vi "DialogCreateMethod.vi"(0 "ClassWriterNative":refnum<class "ClassWriterNative.lvclass">, 1 "ClassItemRefIn":refnum<vi>, 5 "error in (no error)":errorcluster) -> (14 "ClassWriterNative":refnum<class "ClassWriterNative.lvclass">, 15 "ClassItemRefOut":refnum<vi>, 16 "CreateMethodData":T3={"MethodName"="", "RelativeMethodPath"=path "", "MethodDescription"="", "Scope/Visibility"=enum."Use Parent Folder Scope", "MethodTemplateName"="", "IconOut"=[], "RelativeProjectClassPath"="", "OpenViAfterCreation"=FALSE, "DynamicDispatchVi"=FALSE, "ExtraCreateParameters"=variant, "MustOverride"=FALSE, "MustCallParent"=FALSE, "IconDetails"={"IconSize"=enum."1 c-term high", "ImageRows(32)"=32, "ConnectorPaneHeight"=[]}, "AF-Option"=variant, "TemplatePath"=path ""} {"IconOut" format="%x"}, 17 "Cancelled":bool, 19 "error out":errorcluster)   [LabVIEW 2020, in "ClassWriterNative.lvclass"]
uses:
  <resource>/Framework/Providers/Open_GDS/ClassProviders/Provider_LvNativeClass/ClassWriterNative_class/ClassWriterNative.lvclass
  <resource>/Framework/Providers/Open_GDS/ClassProviders/Common/LvIcon_class/GDSLvIcon_ColorControl.ctl
  <resource>/Framework/Providers/Open_GDS/ClassProviders/Provider_BaseClassInterface/CreateMethodData.ctl
  <resource>/Framework/Providers/Open_GDS/ClassProviders/Provider_EndevoGOOP300/GOOP300_SubVIs/GOOP300_MethodScopeType.ctl
  <resource>/Framework/Providers/Open_GDS/ClassProviders/Provider_LvNativeClass/ClassWriterNative_class/IconDetails.ctl
  <resource>/Framework/Providers/Open_GDS/ClassProviders/Provider_LvNativeClass/ClassWriterNative_class/IconSize.ctl
  <resource>/Framework/Providers/Open_GDS/ClassProviders/Common/LvClass_class/GDSLvClass_PlugIn.ctl
  <resource>/Framework/Providers/Open_GDS/ClassProviders/Common/LvClass_class/GDSLvClass_PlugInTypes.ctl
  <resource>/Framework/Providers/Open_GDS/ClassProviders/Provider_LvNativeClass/ClassWriterNative_class/MethodInfo.ctl
  <resource>/Framework/Providers/Open_GDS/ClassProviders/Provider_LvNativeClass/ClassWriterNative_class/MethodType.ctl
  <vilib>/Utility/miscctls.llb/LVPoint32TypeDef.ctl
  <vilib>/picture/picture.llb/imagedata.ctl
  <resource>/Framework/Providers/Open_GDS/ClassProviders/Provider_BaseClassInterface/ClassWriter_class/TemplateSettings.ctl
  <vilib>/Utility/miscctls.llb/LVRectTypeDef.ctl
  <resource>/Framework/Providers/Open_GDS/ClassProviders/Provider_EndevoGOOP400/EndevoG4ProviderName.ctl
  <vilib>/event_ctls.llb/lveventtype.ctl
  <resource>/Framework/Providers/Open_GDS/ClassProviders/Common/IconEditor/private/GDSIconEditor_IconDialog_Input.vi
  <resource>/Framework/Providers/Open_GDS/ClassProviders/Common/LvIcon_class/subvis/GDSLvIcon_TextDataType.ctl
  <resource>/Framework/Providers/Open_GDS/ClassProviders/Common/LvIcon_class/GDSLvIcon_WordCompressionType.ctl
  <resource>/Framework/Providers/Open_GDS/ClassProviders/Common/LvIcon_class/GDSLvIcon_TextAlignment.ctl
  <vilib>/Utility/miscctls.llb/LVPositionTypeDef.ctl
  <vilib>/Utility/miscctls.llb/LVPointTypeDef.ctl
  55204018-4493-42a1-99d2-4693747e47a6.vi
  5ca582aa-8486-41e5-93f7-81c5295e79eb.vi
  <vilib>/Utility/config.llb/Read Key (String).vi
  <vilib>/Comparison/Equal/Equal Functor/Equal Functor.lvclass
  <vilib>/regexp/Match Regular Expression.xnode
  <resource>/Framework/Providers/Open_GDS/ClassProviders/Provider_BaseClassInterface/ClassWriter_class/ClassWriter.lvclass
  <vilib>/Utility/lvfile.llb/NI_FileType.lvlib
  <resource>/Framework/Providers/Open_GDS/ClassProviders/Provider_EndevoGOOP400/ClassWriterGOOP400_class/ClassWriterGOOP400.lvclass
  <vilib>/Utility/config.llb/NI_LVConfig.lvlib
  <resource>/Framework/Providers/Open_GDS/ClassProviders/Provider_EndevoGOOP300/ClassWriterGOOP300_class/ClassWriterGOOP300.lvclass
panel:
  out "MethodTemplateImage":picture
  in  "_AddFolder":bool
  in  "Filter":string
  in  ".vim":bool
  out "_MethodsLlocationOverrideInfo":string=" \n\n" caption="The methods location is controlled by\nthe method you override."
  out "ProductPicture":picture
  out "_IconPreview":picture caption="Icon Preview"
  out "DragIcon":picture
  in  "_AddMessageClass":bool
  in  "FloodFillMask":bool
  out "_IconName":string
  in  "_IconSearchText":string caption="Icon search text"
  in  "_Manage":bool
  in  "_Folders":u16(ring) caption="Folders" items=["<All icons>", "C:\\Users\\Mikael\\Documents\\LabVIEW Data\\Glyphs", "...EW 2010\\resource\\Framework\\Providers\\Icons", "...\\Framework\\Providers\\Symbio_GDS_SVN\\Glyphs", "...e\\Framework\\Providers\\Symbio_GDS_SVN\\Icons"]
  out "Icons":picture
  in  "_MethodIcons":bool
  in  "_TextAlignment":u16(ring) caption="Text Alignment" items=["Center", "Left", "Right"]
  in  "_IconSize":u16(ring) caption="Icon Size" items=["Full", "1 c-term high", "2 c-term high", "3 c-term high"]
  in  "_MustCallParent":bool caption="Must Call Parent"
  in  "_MustOverride":bool caption="Must Override"
  out "_VisibilityAndLlocationGrouping":string caption="Visibility and location"
  out "_IconGrouping":string caption="Icon"
  in  "_MethodSignature":u16(ring) caption="Method signature" items=["No signature", "-", "Add signature"]
  in  "_ShowContextHelp":bool
  in  "Help":bool
  in  "_CreateOpenClass":bool
  in  "_MethodIconName":string caption="Body Text"
  in  "_BodyBk":T1 caption="Body Background"
  in  "_BodyText":T1 caption="Body text"
  in  "_FontCompression":enum16{"Auto", "On", "Off"}(ring) caption="Font Compression"
  in  "_CapitalOnly":bool=TRUE caption="Force Capital Letters"
  out "_DubMethodName":string caption="This method already exists in the class"
  out "_Loading":string caption="Loading..."
  in  "_OverrideMethods":i32(listbox) caption="Override Methods"
  in  "_MethodType":T2(radio) caption="Method Type"
  in  "_Property":string[](tree) caption="Data Fields/Attributes"
  in  "_DynamicDispatch":bool caption="Dynamic Dispatch"
  in  "_Visibility":T7(radio) caption="Visibility"
  in  "_MethodLocation":i32(listbox) caption="Method Location"
  in  "_MethodName":string caption="Method Name"
  in  "_Cancel":bool
  in  "_CreateMethod":bool
  in  "_MethodDescription":string caption="Method description"
  in  "_Method":i32[](listbox) caption="Method Template"
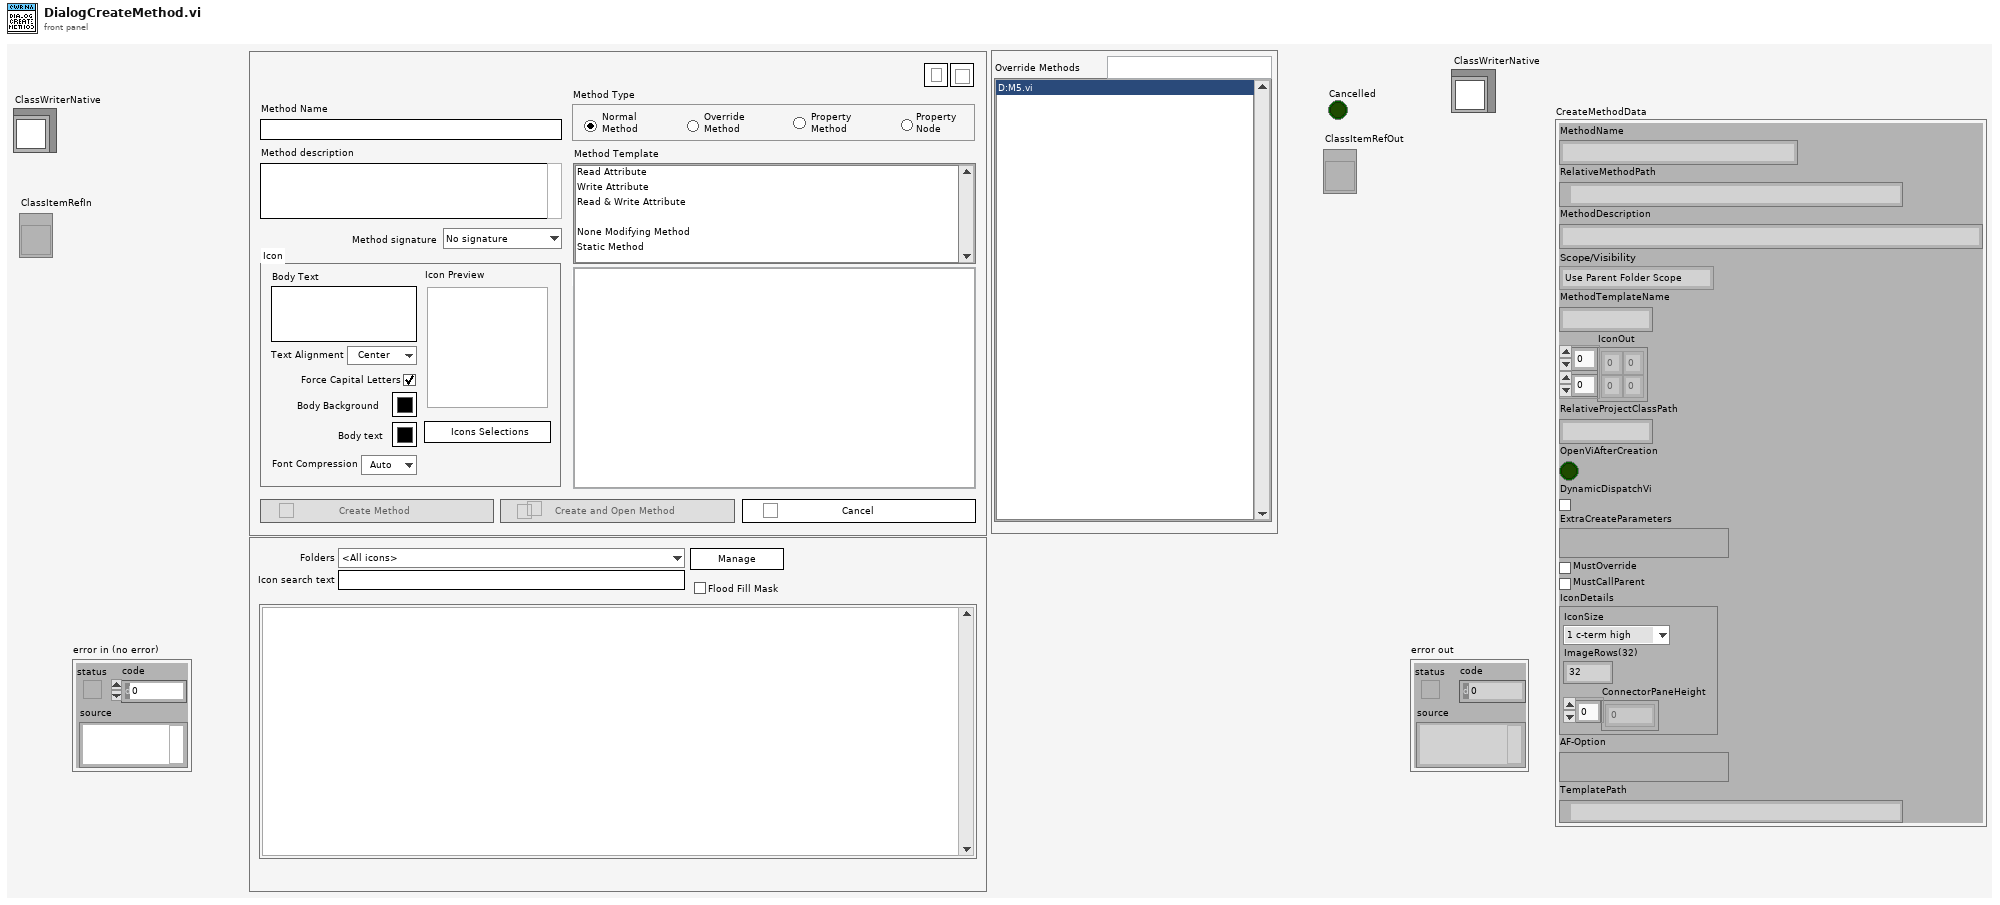
[diagram p1: front panel]
types:
  T1 = typedef "GDSLvIcon_ColorControl.ctl" = cluster{"Decal":bool, "Color":u32}
  T2 = enum32{"Normal Method", "Override Method", "Property Method", "Property Node"}
  T3 = typedef "ClassWriter.lvclass/CreateMethodData.ctl" = cluster{"MethodName":string, "RelativeMethodPath":path, "MethodDescription":string, "Scope/Visibility":T4, "MethodTemplateName":string, "IconOut":u8[][], "RelativeProjectClassPath":string, "OpenViAfterCreation":bool, "DynamicDispatchVi":bool, "ExtraCreateParameters":variant, "MustOverride":bool, "MustCallParent":bool, "IconDetails":T5, "AF-Option":variant, "TemplatePath":path}
  T4 = typedef "GOOP300_MethodScopeType.ctl" = enum16{"Use Parent Folder Scope", "Public", "Protected", "Private", "Community"}
  T5 = typedef "ClassWriterNative.lvclass/IconDetails.ctl" = cluster{"IconSize":T6, "ImageRows(32)":i32, "ConnectorPaneHeight":i32[]}
  T6 = typedef "ClassWriterNative.lvclass/IconSize.ctl" = enum16{"Full", "1 c-term high", "2 c-term high", "3 c-term high"}
  T7 = enum32{"Public", "Community", "Protected", "Private"}
  T8 = cluster{"Font Name":string, "Size":u16, "Bold":bool, "Italic":bool, "Underline":bool, "Strikeout":bool, "Color":u32}
  T9 = cluster{"AttributeNames":string[], "PropertyNode":bool, "FolderNames":string[]}
  T10 = typedef "GDSLvClass_PlugIn.ctl" = cluster{"Type":T11, "ID":string, "Version":string, "Path":path, "Name":string, "Data":variant}
  T11 = typedef "GDSLvClass_PlugInTypes.ctl" = enum16{"DesignPattern", "MethodTypes"}
  T12 = typedef "ClassWriterNative.lvclass/MethodInfo.ctl" = cluster{"Type":T13, "Name":string, "Path":path, "ExtraName":string, "Data":variant}
  T13 = typedef "ClassWriterNative.lvclass/MethodType.ctl" = enum16{"Normal", "MethodPlugIn", "DesignPattern", "AF-Method"}
  T14 = typedef "LVPoint32TypeDef.ctl" = cluster{"Horizontal":i32, "Vertical":i32}
  T15 = typedef "imagedata.ctl" = cluster{"image type":i32, "image depth":i32, "image":u8[], "mask":u8[], "colors":u32[], "Rectangle":cluster{"left":i16, "top":i16, "right":i16, "bottom":i16}}
  T16 = typedef "ClassWriter.lvclass/TemplateSettings.ctl" = cluster{"CommonClassTemplate":bool, "DynamicDispatch":enum8{"False", "True", "Mixed"}, "MustOverride":enum8{"False", "True", "Mixed"}, "MustCallParent":enum8{"False", "True", "Mixed"}, "OnlyNormalMethod":bool, "OnlyPublic":bool}
  T17 = cluster{"Cancel":bool, "FolderNames":string[], "FolderPath":path[], "FolderType":enum32{"invalid scope", "public", "private", "protected", "community"}[], "ClassName":string, "ColorProtected":u32, "ColorPrivate":u32, "ColorPublic":u32, "Frame":u32, "Frame thickness":i32, "HeaderIcon":u8[][], "BodyIconHeight":i32, "BodyIconWidth":i32, "RelFolderPath":path[], "MethodIcon":u8[][], "OverRideLookUpDone":bool, "PropertyLookUpDone":bool, "AllOverrideMethods":path[], "ClassVIs":string[], "Open":bool, "OverrideScope":enum32{"invalid scope", "public", "private", "protected", "community"}[], "Signatures":cluster{"SignatureName":string[], "SignatureText":string[], "Current":i32}, "DesignPatterns":T10[], "NormalMethods":T12[], "OverrideMethods":T12[], "PropertyMethods":T12[], "MethodNames":string[], "ConnectorPaneHeight":i32[], "IconDetails":T5, "Offset":cluster{"X":i32, "Y":i32}, "OldOffset":cluster{"X":i32, "Y":i32}, "TextBounds":cluster{"FirstRow":i32, "FirstColumn":i32, "LastRow":i32, "LastColumn":i32}, "DraggingText":bool, "StartTextDraggingPos":T14, "Folders":path[], "IconPaths":cluster{i32, "path out":path}[], "Icons":T15[], "IconNames":string[], "DraggingIcon":bool, "StartTextDraggingPos 2":T14, "BgIconOffset":cluster{"X":i32, "Y":i32}, "Offset 2":cluster{"X":i32, "Y":i32}, "OldOffset 2":cluster{"X":i32, "Y":i32}, "CurrentIcon":cluster{"BgIcon":u8[][], "BgIconOffset":cluster{"X":i32, "Y":i32}, "BgIconMask":u8[], "ColorsOkayforiconToBeOnTopOf":u8[]}, "BgIconMask":u8[], "BodyIcon":u8[][], "BgIcon":u8[][], "HeaderBkColor":u32, "IconOut":u8[][], "IconSelected":i32, "IconDropped":i32, "Moving":bool, "IconPos":cluster{"left":i16, "top":i16, "right":i16, "bottom":i16}[], "BodyIconOut":u8[][], "AF":bool, "ActorVersion":string, "AF-MethodNames":string[], "AF-Methods":cluster{T12[]}[], "AF-Method":i32, "PropertyNodeMethods":T12[], "MethodLocation":string[][], "MethodCaptionName":string, "IsAPropertyDefinitionVI":bool[], "TemplateSettings":T16, "OverrideMethod":path, "Interface":bool, "RowStart(0)":i32, "ImageRows(32)":i32, "MethodVIs":path[], "MethodItemNames":string[], "OverrideMethodsNames":string[], "OverrideMethodsIdx":i32[]}
  T18 = typedef "LVBoundsTypeDef.ctl" = cluster{"Width":u32, "Height":u32}
  T19 = enum8{"Enabled", "Disabled", "Disabled and Grayed Out"}
  T20 = enum16{"Full", "1 c-term high", "2 c-term high", "3 c-term high", "Off"}
  T21 = typedef "EndevoG4ProviderName.ctl" = enum16{"EndevoGOOP400"}
  T22 = enum32{"invalid scope", "public", "private", "protected", "community"}
  T23 = typedef "LVRectTypeDef.ctl" = cluster{"Left":i16, "Top":i16, "Right":i16, "Bottom":i16}
  T24 = typedef "lveventtype.ctl" = enum32{"Null", "Timeout", "Annotation Menu Selection", "Annotation Menu Selection?", "App Instance Close", "App Instance Close?", "Autoscale Range Change", "Bookmark Info Change", "Cell Edit", "Cell Edit?", "Cursor Grab", "Cursor Grab?", "Cursor Menu Selection", "Cursor Menu Selection?", "Cursor Move", "Cursor Release", "Data Change", "Direction Change", "Display State Change", "Drag Ended", "Drag Enter", "Drag Leave", "Drag Over", "Drag Source Update", "Drag Starting", "Drag Starting?", "Drop", "Exec State Change", "Key Down", "Key Down?", "Key Repeat", "Key Repeat?", "Key Up", "Listbox Double Click", "Menu Activation?", "Menu Selection (App)", "Menu Selection? (App)", "Menu Selection (User)", "Mouse Down", "Mouse Down?", "Mouse Enter", "Mouse Leave", "Mouse Move", "Mouse Up", "Mouse Wheel", "NI Security User Change (App)", "Pane Size", "Panel Close", "Panel Close?", "Panel Resize", "Plot Attribute Change", "Scale Range Change", "Shortcut Menu Activation?", "Shortcut Menu Selection (App)", "Shortcut Menu Selection? (App)", "Shortcut Menu Selection (User)", "Tree Double Click", "Tree Drag", "Tree Drag?", "Tree Drop", "Tree Drop?", "Tree Item Close", "Tree Item Close?", "Tree Item Open", "Tree Item Open?", "User Event", "Value Change"}
  T25 = typedef "GDSIconEditor_IconDialog_Input.vi" = cluster{"HeaderIcon":u8[][], "RowStart(0)":i32, "ImageRows(32)":i32, "FrameThickness(1)":u32, "FrameColor":u32, "IconTextDataType":T26, "BodyTextColor":u32, "BodyBackgroundColor":u32, "BodyIconHeight":i32, "BodyIconWidth":i32, "HeaderBackgroundColor":u32, "BodyIcon":u8[][], "Offset":cluster{"X":i32, "Y":i32}, "CurrentIcon":cluster{"BgIcon":u8[][], "BgIconOffset":cluster{"X":i32, "Y":i32}, "BgIconMask":u8[], "ColorsOkayforiconToBeOnTopOf":u8[]}}
  T26 = typedef "GDSLvIcon_TextDataType.ctl" = cluster{"Text":string, "Allow Only Capital Chars":bool, "Compression":T27, "Alignment":T28}
  T27 = typedef "GDSLvIcon_WordCompressionType.ctl" = enum16{"Auto", "On", "Off"}
  T28 = typedef "GDSLvIcon_TextAlignment.ctl" = enum16{"Center", "Left", "Right"}
  T29 = typedef "LVPositionTypeDef.ctl" = cluster{"Left":i32, "Top":i32}
  T30 = typedef "LVPointTypeDef.ctl" = cluster{"Horizontal":i16, "Vertical":i16}
  T31 = enum32{"invalid scope", "public", "private", "protected", "community"}[]
  T32 = typedef "GOOP400_Options.ctl" = cluster{"FlatFolderStructure":bool}
  T33 = cluster{"Major":u16, "Minor":u16, "Fix":u16, "Build":u16}
  T34 = typedef "AF_ClassType.ctl" = enum16{"NA", "Actor", "Message"}
  T35 = typedef "GDSLvClass_IconSettingsType.ctl" = cluster{"Frame":u32, "Frame thickness":u8, "Header Background":u32, "Header Text":u32, "ColorPublic":u32, "ColorProtected":u32, "ColorPrivate":u32, "Body Text":u32, "ClassBodyIcon":string}
  T36 = cluster{"SignatureName":string[], "SignatureText":string[], "Current":i32}
  T37 = typedef "BaseProvider_IniFileSettings.ctl" = cluster{"ClassFolderSuffix":string, "InterfaceFolderSuffix":string, "InterfaceIcon":string, "FileNamingOption":T38}
  T38 = typedef "BaseProvider_FileNamingOption.ctl" = enum16{"CamelCase", "Space", "Underscore"}
  T39 = typedef "eventvkey.ctl" = enum16{"ASCII", "Enter", "Return", "Shift", "Ctrl", "Alt", "Cmd", "Opt", "Caps", "NumLock", "Clear", "Break", "Up", "Down", "Left", "Right", "Insert", "Delete", "Home", "End", "PageUp", "PageDown", "Escape", "Help", "Pause", "ScrollLock", "F1", "F2", "F3", "F4", "F5", "F6", "F7", "F8", "F9", "F10", "F11", "F12", "F13", "F14", "F15", "F16", "F17", "F18", "F19", "F20", "F21", "F22", "F23", "F24", "Play", "VolumeUp", "VolumeDown", "Mute", "Two Byte Char"}
  T40 = cluster{"BgIcon":u8[][], "BgIconOffset":cluster{"X":i32, "Y":i32}, "BgIconMask":u8[], "ColorsOkayforiconToBeOnTopOf":u8[]}
  T41 = cluster{"left":i16, "top":i16, "right":i16, "bottom":i16}[]
  T42 = typedef "LVMouseTypeDef.ctl" = cluster{"Mouse Position":cluster{"X":i32, "Y":i32}, "Mouse Modifiers":cluster{"Button Down":bool, "Shift Mod":bool, "Menu Mod":bool, "Option Mod":bool}}
  T43 = cluster{"FirstRow":i32, "FirstColumn":i32, "LastRow":i32, "LastColumn":i32}
  T44 = typedef "ColorControl.ctl" = cluster{"Decal":bool, "Color":u32}
  T45 = cluster{"left":i16, "top":i16, "right":i16, "bottom":i16}
  T46 = typedef "NI_LVConfig.lvlib/Config Data RefNum.ctl" = refnum<k1>
  T47 = cluster{"PlugInName":string, "MethodSelected":string}
  T48 = cluster{"SignatureName":string[], "SignatureText":string[], i32}
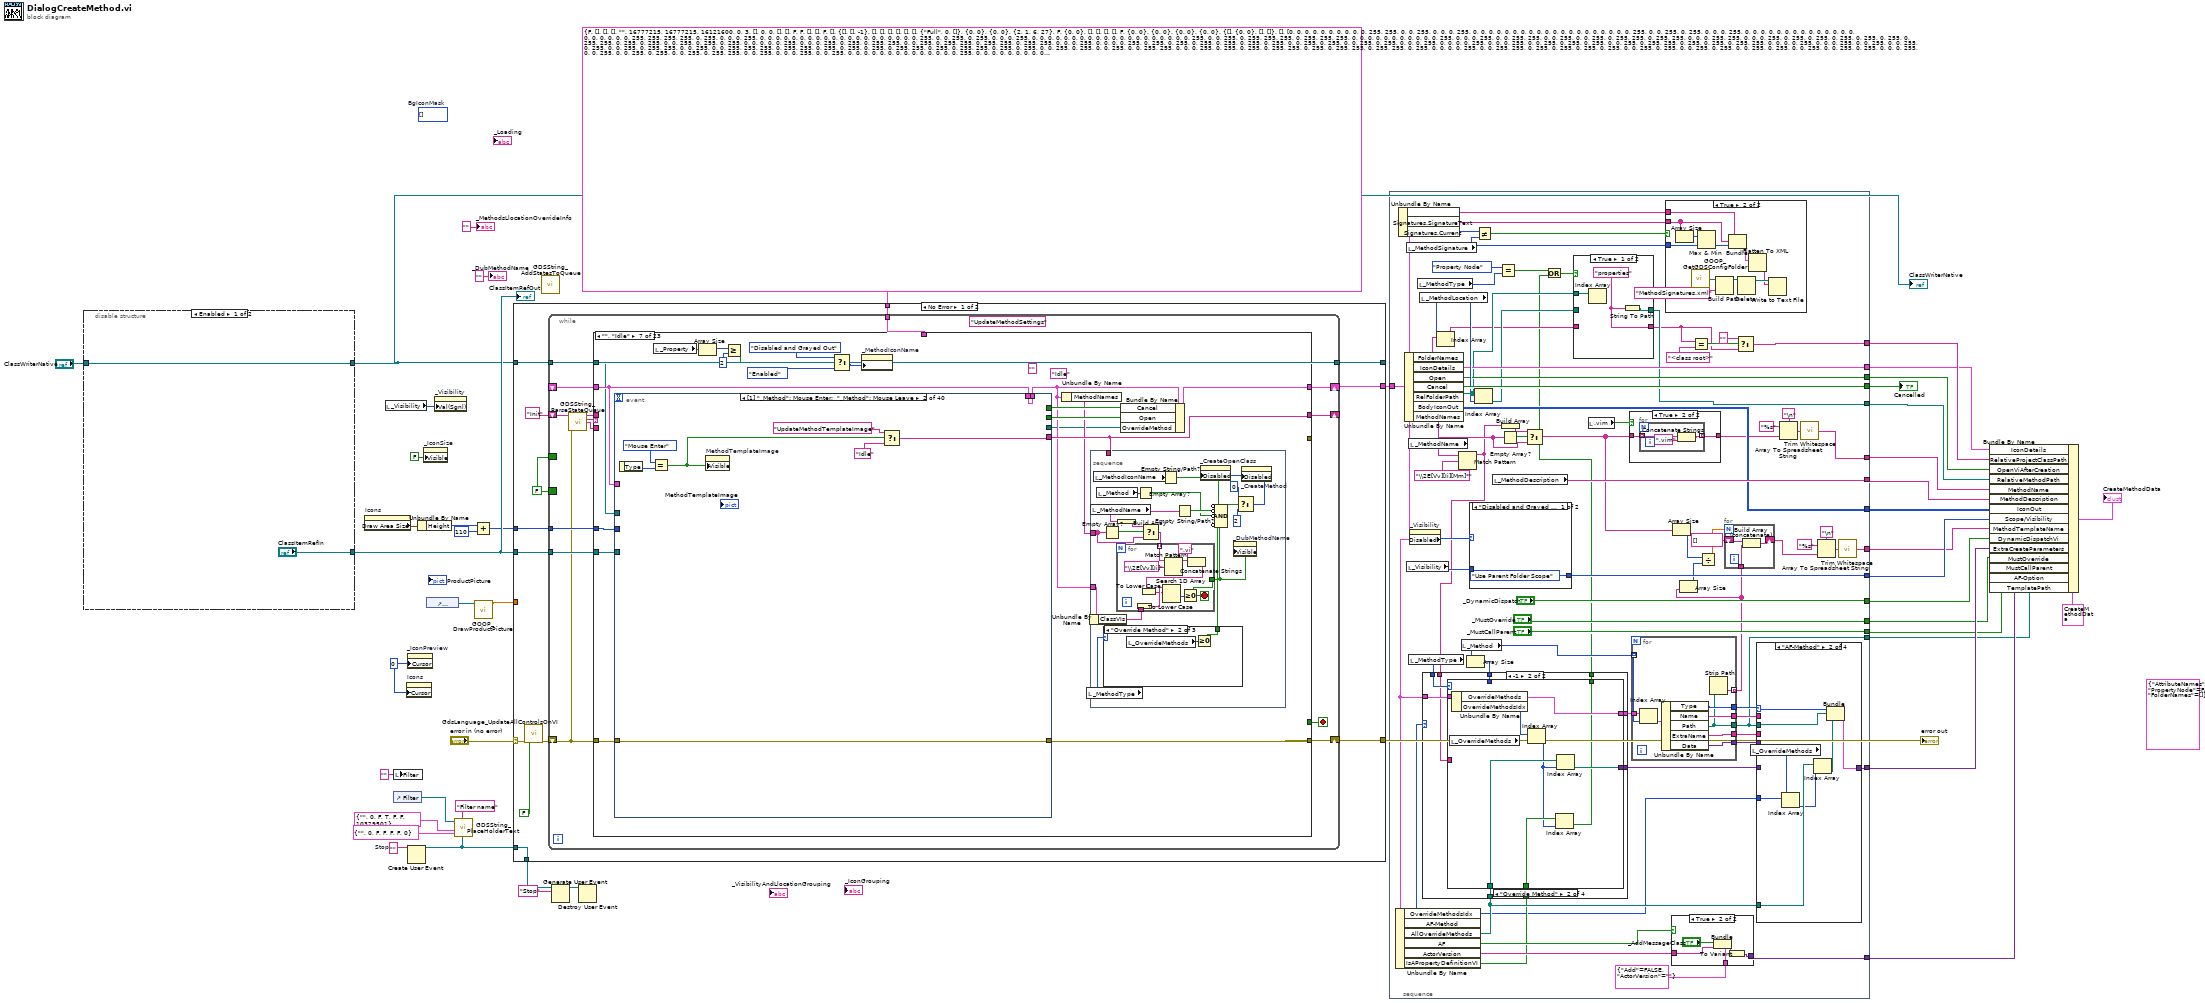
[diagram p0: block diagram]
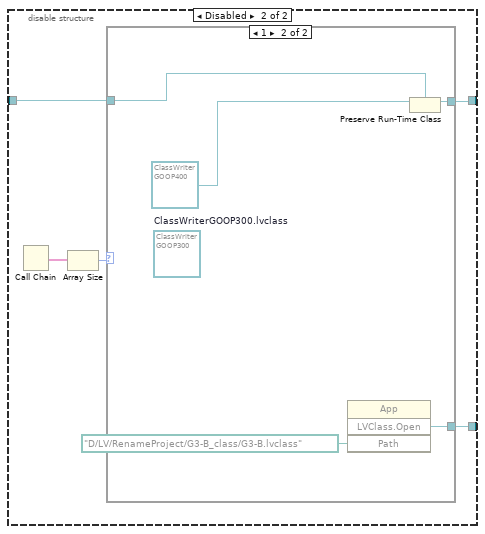
[diagram p2: hidden frame]
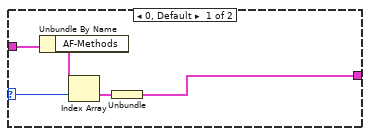
[diagram p6: hidden frame]
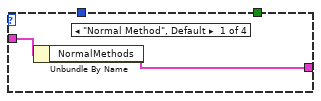
[diagram p7: hidden frame]
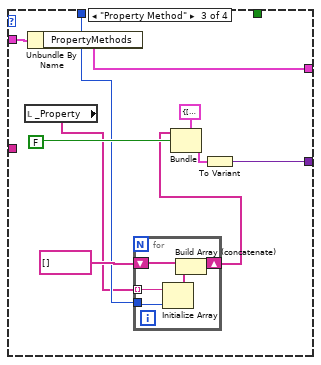
[diagram p8: hidden frame]
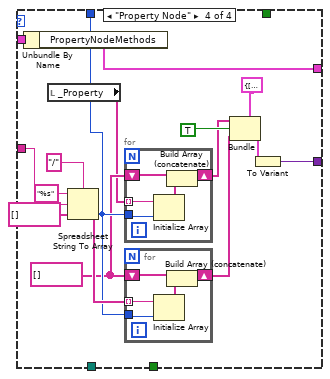
[diagram p9: hidden frame]
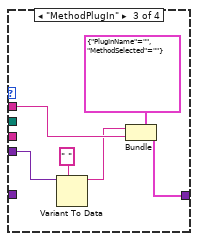
[diagram p12: hidden frame]
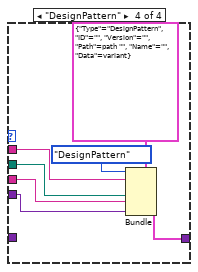
[diagram p13: hidden frame]
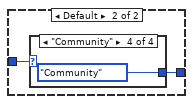
[diagram p15: hidden frame]
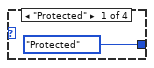
[diagram p16: hidden frame]
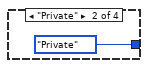
[diagram p17: hidden frame]
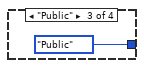
[diagram p18: hidden frame]
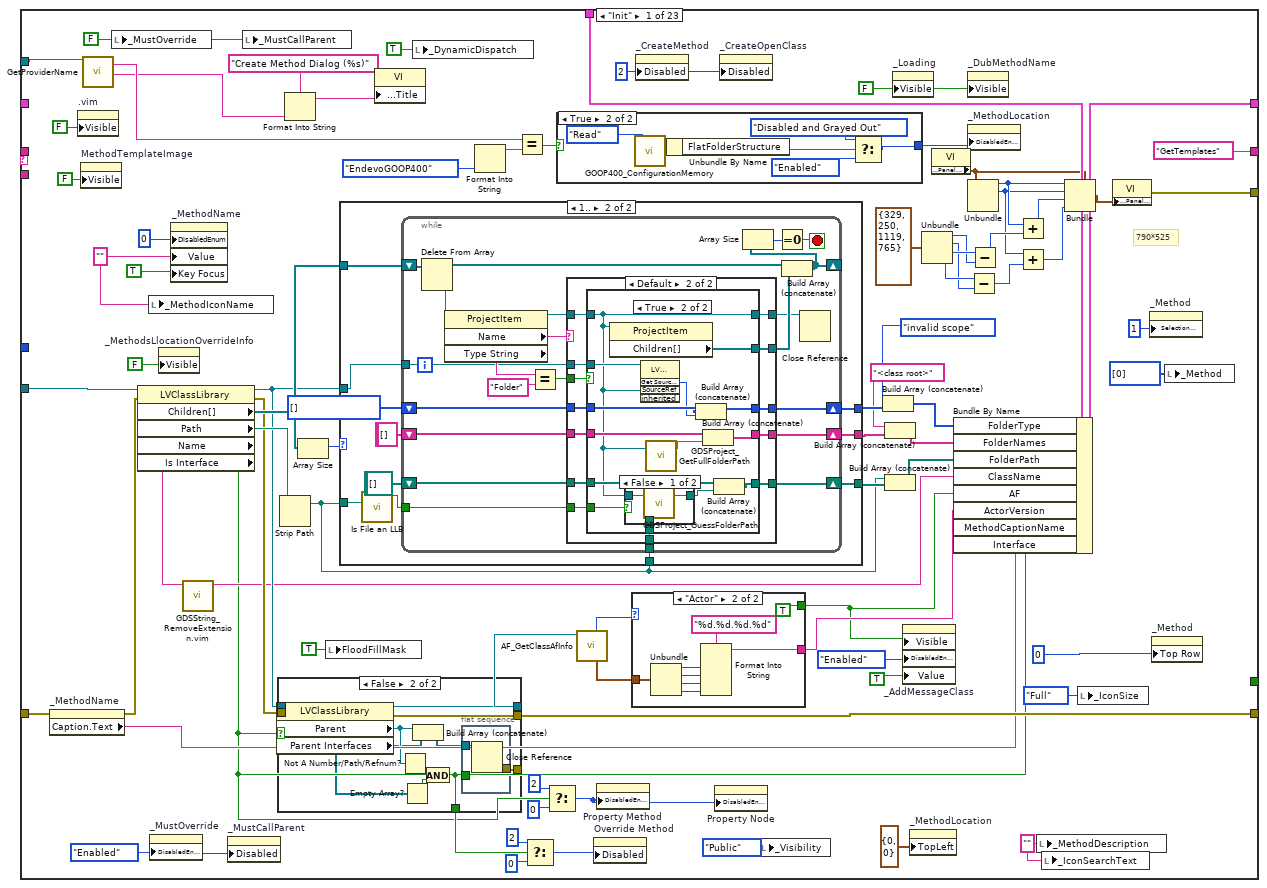
[diagram p19: hidden frame]
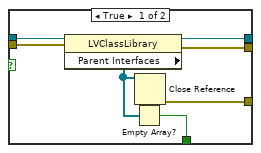
[diagram p20: hidden frame]
diagram:
  w8 = ""  # Stop
  (unwired) T9 {"AttributeNames"=[], "PropertyNode"=FALSE, "FolderNames"=[]} ("cluster")
  w18 = 0 ("Cursor")
  (unwired) u8[] []  # BgIconMask
  n1 = disable-structure shown="Enabled" {
    disable-tunnel: [w47 w52] -> w13
    disable-tunnel: ["ClassItemRefIn" w53] -> w28
    disable-tunnel: "ClassWriterNative" -> [w47 w51]
    frame Enabled {
    }
    frame Disabled {
      n2 = Call Chain() -> (call chain=w50:string[])
      n3 = Array Size(array=w50) -> (size(s)=w49:i32)
      n4 = case shown="1" w49 {
        tunnel: [_ w59] -> w53
        tunnel: [w54 w57] -> w52
        tunnel: w51 -> [w54 w56]
        frame Default {
        }
        frame 1 {
          (unwired) refnum<class "ClassWriterGOOP300.lvclass"> refnum  # ClassWriterGOOP300.lvclass
          n5 = invoke class="App" method="LVClass.Open"("Path"=path "D:/LV/RenameProject/G3-B_class/G3-B.lvclass") -> ("LVClass.Open"=w59:refnum<vi>)  [unwired: 3 in, 3 out]
          n6 = Preserve Run-Time Class(object in=refnum<class "ClassWriterGOOP400.lvclass"> refnum, 2:w56) -> (object out=w57:refnum<class "ClassWriterNative.lvclass">)  [unwired: 1 in, 1 out]
        }
      }
    }
  }
  "ClassWriterNative" <- w13
  "ClassItemRefOut" <- w28
  n7 = property on="Icons" class="Pict"() -> ("Draw Area Size"=w24:T18)  [unwired: 2 in, 2 out]
  n8 = local read "_Visibility"() -> (w11:T7)
  n9 = control-ref of="Filter"() -> (w2:refnum<vi>)
  n10 = local write "Filter"("" ("Filter")) -> ()
  n11 = property on="Icons" class="Pict"("Cursor"=w18) -> ()  [unwired: 2 in, 2 out]
  n12 = property on="_IconPreview" class="Pict"("Cursor"=w18) -> ()  [unwired: 2 in, 2 out]
  n13 = Create User Event(user event datatype=w8) -> (user event=w4:refnum<user-event>)  [unwired: 1 in, 1 out]
  n14 = Unbundle By Name(w24) -> ("Height"=w22:u32)
  n15 = property on="_IconSize" class="Ring (strict)"("Visible"=FALSE) -> ()  [unwired: 2 in, 2 out]
  n16 = control-ref of="ProductPicture"() -> (w17:refnum<vi>)
  n17 = property on="_Visibility" class="RadioBtnsControl (strict)"("Val(Sgnl)"=w11) -> ()  [unwired: 2 in, 2 out]
  n18 = call <resource>:"GDSString_PlaceHolderText.vi"("BooleanUserEventToStopPlaceHolderVI"=w4, "PlaceholderText"="Filter name" ("InterfaceFilter"), "PlaceholderTextFont(Grey,Italic)"=T8 {"Font Name"="", "Size"=0, "Bold"=FALSE, "Italic"=TRUE, "Underline"=FALSE, "Strikeout"=FALSE, "Color"=10329501}, "NormalTextFont(Black)"=T8 {"Font Name"="", "Size"=0, "Bold"=FALSE, "Italic"=FALSE, "Underline"=FALSE, "Strikeout"=FALSE, "Color"=0}, "PlaceholderStringRef"=w2) -> ()  [unwired: 6 in, 1 out]
  n19 = Add(x=w22, y=u32 110) -> (x+y=w21:u32)
  n20 = call <resource>:"GOOP_DrawProductPicture.vi"("ProductPictureControl"=w17) -> ("Zoom Factor"=w16:sgl)  [unwired: 10 in]
  n21 = case shown="No Error" "error in (no error)" {
    selector: "error in (no error)" -> [w66 w2849]
    tunnel: w13 -> [w70 w2848]
    tunnel: [w72 w2849] -> w32
    tunnel: [w71 w2848] -> _
    tunnel: T17 {"Cancel"=FALSE, "FolderNames"=[], "FolderPath"=[], "FolderType"=[], "ClassName"="", "ColorProtected"=16777215, "ColorPrivate"=16777215, "ColorPublic"=16121600, "Frame"=0, "Frame thickness"=3, "HeaderIcon"=[], "BodyIconHeight"=0, "BodyIconWidth"=0, "RelFolderPath"=[], "MethodIcon"=[], "OverRideLookUpDone"=FALSE, "PropertyLookUpDone"=FALSE, "AllOverrideMethods"=[], "ClassVIs"=[], "Open"=FALSE, "OverrideScope"=[], "Signatures"={"SignatureName"=[], "SignatureText"=[], "Current"=-1}, "DesignPatterns"=[], "NormalMethods"=[], "OverrideMethods"=[], "PropertyMethods"=[], "MethodNames"=[], "ConnectorPaneHeight"=[], "IconDetails"={"IconSize"=enum."Full", "ImageRows(32)"=0, "ConnectorPaneHeight"=[]}, "Offset"={"X"=0, "Y"=0}, "OldOffset"={"X"=0, "Y"=0}, "TextBounds"={"FirstRow"=2, "FirstColumn"=1, "LastRow"=6, "LastColumn"=27}, "DraggingText"=FALSE, "StartTextDraggingPos"={"Horizontal"=0, "Vertical"=0}, "Folders"=[], "IconPaths"=[], "Icons"=[], "IconNames"=[], "DraggingIcon"=FALSE, "StartTextDraggingPos 2"={"Horizontal"=0, "Vertical"=0}, "BgIconOffset"={"X"=0, "Y"=0}, "Offset 2"={"X"=0, "Y"=0}, "OldOffset 2"={"X"=0, "Y"=0}, "CurrentIcon"={"BgIcon"=[], "BgIconOffset"={"X"=0, "Y"=0}, "BgIconMask"=[], "ColorsOkayforiconToBeOnTopOf"=[]}, "BgIconMask"=[], "BodyIcon"=[[0, 0, 0, 0, 0, 0, 0, 0, 0, 0, 255, 255, 0, 0, 255, 0, 0, 0, 255, 0, 0, 0, 0, 0, 0, 0, 0, 0, 0, 0], [0, 0, 0, 0, 0, 0, 0, 0, 0, 255, 0, 0, 255, 0, 255, 0, 0, 0, 255, 0, 0, 0, 0, 0, 0, 0, 0, 0, 0, 0], [0, 0, 0, 0, 0, 0, 0, 0, 0, 255, 255, 255, 255, 0, 255, 0, 0, 0, 255, 0, 0, 0, 0, 0, 0, 0, 0, 0, 0, 0], [0, 0, 0, 0, 0, 0, 0, 0, 0, 255, 0, 0, 255, 0, 255, 0, 0, 0, 255, 0, 0, 0, 0, 0, 0, 0, 0, 0, 0, 0], [0, 0, 0, 0, 0, 0, 0, 0, 0, 255, 0, 0, 255, 0, 255, 255, 255, 0, 255, 255, 255, 0, 0, 0, 0, 0, 0, 0, 0, 0], [0, 0, 255, 0, 0, 0, 255, 0, 0, 255, 255, 0, 0, 255, 0, 0, 255, 0, 255, 255, 0, 255, 255, 0, 0, 0, 255, 255, 0, 0], [0, 255, 0, 255, 0, 255, 0, 255, 0, 255, 0, 255, 0, 255, 255, 0, 255, 0, 255, 0, 0, 255, 0, 255, 0, 255, 0, 0, 0, 0], [0, 255, 0, 0, 0, 255, 0, 255, 0, 255, 255, 0, 0, 255, 0, 255, 255, 0, 255, 255, 0, 255, 255, 0, 0, 0, 255, 0, 0, 0], [0, 255, 0, 255, 0, 255, 0, 255, 0, 255, 0, 255, 0, 255, 0, 0, 255, 0, 255, 0, 0, 255, 0, 255, 0, 0, 0, 255, 0, 0], [0, 0, 255, 0, 0, 0, 255, 0, 0, 255, 0, 255, 0, 255, 0, 0, 255, 0, 255, 255, 0, 255, 0, 255, 0, 255, 255, 0, 0, 0], [0, 255, 0, 0, 0, 255, 0, 0, 255, 0, 0, 255, 0, 255, 0, 0, 255, 0, 255, 255, 0, 0, 255, 0, 0, 255, 255, 255, 0, 255], [255, 0, 255, 0, 255, 0, 255, 0, 255, 255, 0, 255, 0, 255, 255, 0, 255, 0, 255, 0, 0, 255, 0, 255, 0, 0, 255, 0, 0, 255], [255, 0, 0, 0, 255, 0, 255, 0, 255, 0, 255, 255, 0, 255, 0, 255, 255, 0, 255, 255, 0, 255, 0, 0, 0, 0, 255, 0, 0, 255], [255, 0, 255, 0, 255, 0, 255, 0, 255, 0, 0, 255, 0, 255, 0, 0, 255, 0, 255, 0, 0, 255, 0, 255, 0, 0, 255, 0, 0, 255], [0, 255, 0, 0, 0, 255, 0, 0, 255, 0, 0, 255, 0, 255, 0, 0, 255, 0, 255, 255, 0, 0, 255, 0, 0, 0, 255, 0, 0, 255], [0, 0, 0, 0, 0, 0, 0, 0, 0, 0, 0, 0, 0, 0, 255, 0, 0, 0, 0, 0, 0, 0, 0, 0, 0, 0, 0, 0, 0, 0], [0, 0, 0, 0, 0, 0, 0, 0, 0, 0, 0, 0, 0, 255, 0, 0, 0, 0, 0, 0, 0, 0, 0, 0, 0, 0, 0, 0, 0, 0], [0, 0, 0, 0, 0, 0, 0, 0, 0, 0, 0, 0, 0, 255, 255, 0, 0, 0, 0, 0, 0, 0, 0, 0, 0, 0, 0, 0, 0, 0], [0, 0, 0, 0, 0, 0, 0, 0, 0, 0, 0, 0, 0, 255, 0, 255, 0, 0, 0, 0, 0, 0, 0, 0, 0, 0, 0, 0, 0, 0], [0, 0, 0, 0, 0, 0, 0, 0, 0, 0, 0, 0, 0, 0, 255, 0, 0, 0, 0, 0, 0, 0, 0, 0, 0, 0, 0, 0, 0, 0], [0, 0, 0, 0, 0, 0, 0, 0, 0, 0, 0, 0, 0, 0, 0, 0, 0, 0, 0, 0, 0, 0, 0, 0, 0, 0, 0, 0, 0, 0], [0, 0, 0, 0, 0, 0, 0, 0, 0, 0, 0, 0, 0, 0, 0, 0, 0, 0, 0, 0, 0, 0, 0, 0, 0, 0, 0, 0, 0, 0]], "BgIcon"=[], "HeaderBkColor"=0, "IconOut"=[], "IconSelected"=0, "IconDropped"=-1, "Moving"=FALSE, "IconPos"=[], "BodyIconOut"=[], "AF"=TRUE, "ActorVersion"="", "AF-MethodNames"=[], "AF-Methods"=[], "AF-Method"=-1, "PropertyNodeMethods"=[], "MethodLocation"=[], "MethodCaptionName"=" ", "IsAPropertyDefinitionVI"=[], "TemplateSettings"={"CommonClassTemplate"=FALSE, "DynamicDispatch"=enum."False", "MustOverride"=enum."False", "MustCallParent"=enum."False", "OnlyNormalMethod"=FALSE, "OnlyPublic"=FALSE}, "OverrideMethod"=path "", "Interface"=TRUE, "RowStart(0)"=0, "ImageRows(32)"=32, "MethodVIs"=[], "MethodItemNames"=[], "OverrideMethodsNames"=[], "OverrideMethodsIdx"=[]} ("output cluster") -> [w69 _]
    tunnel: w28 -> [w68 _]
    tunnel: [w67 _] -> w44
    tunnel: w21 -> [w62 _]
    tunnel: w16 -> [_ _]
    tunnel: [w60 w2847] -> w5
    tunnel: w4 -> [w60 w2847]
    frame No Error {
      w61 = FALSE
      n22 = call <resource>:"GdsLanguage_UpdateAllControlsOnVI.vi"("error in (no error)"=w66, "CreateLanguageFile(Use this to create a languageFile)"=FALSE) -> ("error out"=w65:errorcluster)  [unwired: 16 in, 1 out]
      n23 = while {
        shift-right: [w84] -> w72
        shift-left: w65 -> [w74]
        shift-right: [w79] -> _
        shift-left: "Init" -> [w77]
        shift-right: [w85] -> w67
        shift-left: _ -> [w86]
        tunnel: w70 -> [w83]
        tunnel: [w83] -> w71
        tunnel: w69 -> [w82]
        tunnel: w68 -> [w81]
        tunnel: w62 -> [w80]
        border: w61 -> [_]
        border: w61 -> [_]
        stop <- w78 stop-if-true
        (unwired) "UpdateMethodSettings"
        n24 = call <resource>:"GDSString_ParseStateQueue.vi"("State Queue"=w77, "Error In (no error)"=w74) -> ("Remaining States"=w75:string, "Current State"=w73:string, "Arguments"=w76:string)  [unwired: 9 in, 2 out]
        n25 = case shown="\"\", \"Idle\"" w73 {
          selector: w73 -> [_ _ _ _ _ _ _ _ _ _ _ _ _ w1978 _ _ _ _ _ _ _ w2798 _]
          tunnel: w86 -> [_ w275 w357 w392 w409 w479 w512 w1702 w1777 w1828 w1839 w1928 w1972 w1981 w2109 w2422 w2460 w2487 w2582 w2688 w2741 w2796 w2842]
          tunnel: [w166 w309 w356 w391 w443 w476 w525 w1702 w1777 w1826 w1838 w1927 w1973 w1980 w2147 w2421 w2459 w2514 w2585 w2690 w2751 w2796 w2845] -> w85
          tunnel: w74 -> [w103 w306 w361 w385 w444 w486 w509 w1730 w1800 w1824 w1842 w1931 w1970 w1982 w2146 w2427 w2463 w2522 w2587 w2693 w2745 w2794 w2843]
          tunnel: [w109 w280 w361 w384 w403 w486 w510 w1730 w1800 w1824 w1841 w1930 w1970 w1979 w2145 w2420 w2454 w2523 w2587 w2692 w2737 w2794 w2843] -> w84
          tunnel: w83 -> [w128 w307 _ _ _ _ w508 _ _ _ _ _ _ _ _ _ w2456 _ _ _ _ _ _]
          tunnel: ["GetTemplates" w310 w352 "GetClassColors" "UpdateMethodSignatures" "UpdateIcon" w526 w1731 w1783 "UpdateIcon:2" ("y") "ReadIcons" "DrawIcons" ("y") "Generate icon" "Idle" ("y") "Exit" "Idle" "UpdateIcon" w2527 "Idle" "Idle" ("item tag") "Idle" ("item tag") w2797 "Exit"] -> w79
          tunnel: w82 -> [w164 _ _ _ _ _ _ _ _ _ _ _ _ _ _ _ _ _ _ _ _ _ _]
          tunnel: w81 -> [w165 w304 w365 w387 w413 _ w507 _ _ _ _ _ _ _ _ w2426 w2462 _ w2596 _ _ _ _]
          tunnel: w80 -> [_ _ _ _ _ _ w520 _ _ _ _ _ _ _ _ _ _ _ _ _ _ _ _]
          tunnel: [w95 _ _ _ _ _ _ _ _ _ _ _ _ _ _ _ _ _ _ _ _ _ _] -> _
          tunnel: [_ _ _ _ _ _ _ _ _ _ _ _ _ _ _ _ _ _ _ _ _ _ TRUE ("Cancel")] -> w78
          tunnel: w76 -> [_ _ _ _ _ _ _ _ _ _ _ _ _ _ _ _ _ _ _ _ _ _ _]
          tunnel: w75 -> [_ _ w351 _ _ _ _ w1731 w1783 _ _ _ _ _ _ _ _ _ _ _ _ _ _]
          frame "Init" {
            w100 = FALSE ("Dynamic dispatch")
            w123 = T19."Enabled" ("Disabled")
            w112 = "" ("Method description")
            w139 = FALSE ("Visible")
            w131 = u8 2 ("Disabled")
            w132 = "" ("Method Name")
            # "790*525"
            n26 = property on="_MethodName" class="Str"(error in=w103) -> (error out=w102:errorcluster, "Caption.Text"=w101:string)  [unwired: 1 in, 1 out]
            n27 = property on=".vim" class="Bool (strict)"("Visible"=FALSE) -> ()  [unwired: 2 in, 2 out]
            n28 = property on="MethodTemplateImage" class="Pict"("Visible"=FALSE) -> ()  [unwired: 2 in, 2 out]
            n29 = call-dynamic "GetProviderName.vi"("ClassWriterNative in"=w128) -> ("ProviderName"=w90:string, "TranslatedProviderName"=w87:string)  [unwired: 15 in, 2 out]
            n30 = local write "_MustOverride"(w100) -> ()
            n31 = property class="LVClassLibrary"(reference=w165, error in=w102) -> (reference out=w138:refnum<vi>, error out=w137:errorcluster, "Children[]"=w162:refnum<vi>[], "Path"=w153:path, "Name"=w98:string, "Is Interface"=w92:bool)
            n32 = local write "_MethodIconName"(w132) -> ()
            n33 = property on="_MustOverride" class="Bool (strict)"("DisabledEnum"=w123) -> ()  [unwired: 2 in, 2 out]
            n34 = property on="_MethodsLlocationOverrideInfo" class="Str"("Visible"=FALSE) -> ()  [unwired: 2 in, 2 out]
            n35 = property on="_MethodName" class="Str"("DisabledEnum"=u8 0 ("Disabled"), "Value"=w132, "Key Focus"=TRUE) -> ()  [unwired: 2 in, 2 out]
            n36 = call "GDSString_RemoveExtension.vim"("NameWithExtension"=w98) -> ("NameWithoutExtension"=w97:string)  [unwired: 9 in, 1 out]
            n37 = property on="_MustCallParent" class="Bool (strict)"("Disabled"=w123) -> ()  [unwired: 2 in, 2 out]
            n38 = local write "_MustCallParent"(w100) -> ()
            n39 = case shown="False" w92 {
              tunnel: w138 -> [w174 w185]
              tunnel: w137 -> [w173 w184]
              tunnel: [w171 w183] -> w109
              tunnel: [w170 w182] -> w108
              tunnel: [w169 w175] -> w96
              tunnel: [w168 w181] -> _
              frame True {
                n40 = property class="LVClassLibrary"(reference=w174, error in=w173) -> (reference out=w170:refnum<vi>, error out=w171:errorcluster, "Parent Interfaces"=w172:refnum<vi>[])
                n41 = Empty Array?(array=w172) -> (empty?=w169:bool)
                n42 = Close Reference(reference=w172) -> (error out=w168:errorcluster)  [unwired: 1 in]
              }
              frame False {
                n43 = property class="LVClassLibrary"(reference=w185, error in=w184) -> (reference out=w182:refnum<vi>, error out=w183:errorcluster, "Parent"=w179:refnum<vi>, "Parent Interfaces"=w178:refnum<vi>[])
                n44 = Not A Number/Path/Refnum?(number/path/refnum=w179) -> (NaN/Path/Refnum?=w177:bool)
                n45 = Empty Array?(array=w178) -> (empty?=w176:bool)
                n46 = Build Array (concatenate)(w179, w178) -> (w180:refnum<vi>[])
                n47 = And(x=w177, y=w176) -> (x .and. y?=w175:bool)
                n48 = flat-sequence {
                  tunnel: [w187] -> w181
                  tunnel: w180 -> [w186]
                  tunnel: w175 -> [_]
                  frame #0 {
                    n49 = Close Reference(reference=w186) -> (error out=w187:errorcluster)  [unwired: 1 in]
                  }
                }
              }
            }
            n50 = Strip Path(path=w153) -> (stripped path=w124:path)  [unwired: 1 out]
            n51 = Format Into String(format string="Create Method Dialog (%s)", w87) -> (resulting string=w130:string)  [unwired: 2 in, 1 out]
            n52 = Array Size(array=w162) -> (size(s)=w161:i32)
            n53 = local write "FloodFillMask"(TRUE ("FloodFillMask")) -> ()
            n54 = case shown="1.." w161 {
              tunnel: w162 -> [_ w213]
              tunnel: [_ w211] -> w159
              tunnel: [_ w210] -> w155
              tunnel: [_ w207] -> w157
              tunnel: w138 -> [_ w206]
              tunnel: w124 -> [_ w205]
              tunnel: w124 -> [_ w203]
              frame 0, Default {
              }
              frame 1.. {
                w208 = T31 [] items=["invalid scope", "public", "private", "protected", "community"]
                (unwired) path[] []
                (unwired) string[] []
                n55 = call <vilib>:"Is File an LLB.vi"("path"=w205) -> ("Is LLB?"=w204:bool)  [unwired: 9 in, 1 out]
                n56 = while {
                  shift-right: [w216] -> _
                  shift-left: w213 -> [w235]
                  shift-right: [w225] -> w211
                  shift-left: path[] [] -> [w224]
                  shift-right: [w218] -> w210
                  shift-left: string[] [] -> [w221]
                  shift-right: [w219] -> w207
                  shift-left: w208 -> [w220]
                  tunnel: w206 -> [w217]
                  tunnel: w204 -> [w215]
                  tunnel: w203 -> [w214]
                  stop <- w232 stop-if-true
                  n57 = Delete From Array(array=w235) -> (deleted portion=w231:refnum<vi>, array with subset deleted=w234:refnum<vi>[])  [unwired: 2 in]
                  n58 = property class="ProjectItem"(reference=w231) -> (reference out=w227:refnum<vi>, "Name"=w222:string, "Type String"=w230:string)  [unwired: 1 in, 1 out]
                  n59 = Equal?(x=w230, y="Folder") -> (x = y?=w228:bool)
                  n60 = case shown="Default" w222 {
                    tunnel: w228 -> [_ w252]
                    tunnel: w227 -> [w238 w251]
                    tunnel: [_ w250] -> w226
                    tunnel: [w236 w243] -> w218
                    tunnel: [w239 w249] -> w225
                    tunnel: w224 -> [w239 w248]
                    tunnel: [w238 w247] -> w223
                    tunnel: w221 -> [w236 w246]
                    tunnel: w220 -> [w237 w245]
                    tunnel: [w237 w244] -> w219
                    tunnel: w217 -> [_ w242]
                    tunnel: w215 -> [_ w241]
                    tunnel: w214 -> [_ w240]
                    frame "Util", "Utils" {
                    }
                    frame Default {
                      n61 = case shown="True" w252 {
                        tunnel: w251 -> [w255 w260]
                        tunnel: [_ w270] -> w250
                        tunnel: [w253 w269] -> w243
                        tunnel: w248 -> [w256 w267]
                        tunnel: [w256 w268] -> w249
                        tunnel: [w255 w260] -> w247
                        tunnel: w246 -> [w253 w263]
                        tunnel: w245 -> [w254 w265]
                        tunnel: [w254 w264] -> w244
                        tunnel: w242 -> [_ w262]
                        tunnel: w241 -> [_ w258]
                        tunnel: w240 -> [_ w257]
                        frame False {
                        }
                        frame True {
                          n62 = property class="ProjectItem"(reference=w260) -> ("Children[]"=w270:refnum<vi>[])  [unwired: 1 in, 2 out]
                          n63 = case shown="False" w258 {
                            tunnel: [w272 w273] -> w266
                            tunnel: w260 -> [w271 _]
                            tunnel: w257 -> [_ w273]
                            frame False {
                              n64 = call <resource>:"GDSProject_GuessFolderPath.vi"("ProjectItem"=w271) -> ("Path"=w272:path)  [unwired: 15 in, 3 out]
                            }
                            frame True {
                            }
                          }
                          n65 = invoke class="LVClassLibrary" method="Get Source Scope"(reference=w262, "SourceRef"=w260) -> ("GetSourceScope"=w261:T22)  [unwired: 3 in, 4 out]
                          n66 = call <resource>:"GDSProject_GetFullFolderPath.vi"("Folder Item"=w260) -> ("ProjectClassPath"=w259:string)  [unwired: 17 in, 1 out]
                          n67 = Build Array (concatenate)(w265, w261) -> (w264:T31)
                          n68 = Build Array (concatenate)(w263, w259) -> (w269:string[])
                          n69 = Build Array (concatenate)(w267, w266) -> (w268:path[])
                        }
                      }
                    }
                  }
                  n70 = Build Array (concatenate)(w234, w226) -> (w216:refnum<vi>[])
                  n71 = Array Size(array=w216) -> (size(s)=w233:i32)
                  n72 = Equal To 0?(x=w233) -> (x = 0?=w232:bool)
                  n73 = Close Reference(reference=w223) -> ()  [unwired: 1 in, 1 out]
                }
              }
            }
            n74 = property class="VI"("Front Panel.Title"=w130) -> ()  [unwired: 2 in, 2 out]
            n75 = local write "_DynamicDispatch"(TRUE ("Dynamic dispatch")) -> ()
            n76 = Format Into String(EndevoG4ProviderName."EndevoGOOP400" ("ProviderName")) -> (resulting string=w119:string)  [unwired: 3 in, 1 out]
            n77 = Equal?(x=w90, y=w119) -> (x = y?=w118:bool)
            n78 = Select(t=u8 2 ("Disabled"), s=w96, f=u8 0 ("Disabled")) -> (s? t:f=w136:u8)
            n79 = Select(t=u8 2 ("Disabled"), s=w92, f=u8 0 ("Disabled")) -> (s? t:f=w91:u8)
            n80 = case shown="True" w118 {
              tunnel: [T19."Enabled" ("Disabled") w198] -> w117
              frame False {
              }
              frame True {
                n81 = call <resource>:"GOOP400_ConfigurationMemory.vi"("Action"=enum16{"Read", "Load", "Save"}."Read") -> ("OptionsOut"=w201:T32)  [unwired: 17 in, 1 out]
                n82 = Unbundle By Name(w201) -> ("FlatFolderStructure"=w200:bool)
                n83 = Select(t=T19."Disabled and Grayed Out", s=w200, f=T19."Enabled" ("Disabled")) -> (s? t:f=w198:T19)
              }
            }
            n84 = call <resource>:"AF_GetClassAfInfo.vi"("DeriveFromClassRef"=w108) -> ("AF Library Version"=w107:T33, "ClassType"=w105:T34)  [unwired: 5 in, 4 out]
            n85 = property on="Override Method" class="Bool (strict)"("Disabled"=w136) -> ()  [unwired: 2 in, 2 out]
            n86 = property on="Property Method" class="Bool (strict)"("DisabledEnum"=w91) -> ()  [unwired: 2 in, 2 out]
            n87 = case shown="\"Actor\"" w105 {
              tunnel: w107 -> [_ w190]
              tunnel: [_ w189] -> w106
              tunnel: [_ TRUE ("LimitToSpecificProviderTypeOfSameType(True)")] -> w104
              frame "NA", Default {
              }
              frame "Actor" {
                n88 = Unbundle(w190) -> ("Major"=w194:u16, "Minor"=w193:u16, "Fix"=w192:u16, "Build"=w191:u16)
                n89 = Format Into String(format string="%d.%d.%d.%d", w194, w193, w192, w191) -> (resulting string=w189:string)  [unwired: 2 in, 1 out]
              }
            }
            n90 = property on="_CreateMethod" class="Bool"("Disabled"=w131) -> ()  [unwired: 2 in, 2 out]
            n91 = property on="Property Node" class="Bool (strict)"("DisabledEnum"=w91) -> ()  [unwired: 2 in, 2 out]
            n92 = property on="_CreateOpenClass" class="Bool"("Disabled"=w131) -> ()  [unwired: 2 in, 2 out]
            n93 = local write "_Visibility"(T7."Public" ("_Visibility")) -> ()
            n94 = Build Array (concatenate)(T22."invalid scope" ("Source Scope:Get"), w157) -> (w156:T31)
            n95 = Build Array (concatenate)("<class root>" ("Name"), w155) -> (w160:string[])
            n96 = Build Array (concatenate)(w124, w159) -> (w158:path[])
            n97 = property on="_Loading" class="Str"("Visible"=w139) -> ()  [unwired: 2 in, 2 out]
            n98 = property on="_AddMessageClass" class="Bool (strict)"("Visible"=w104, "DisabledEnum"=T19."Enabled" ("Disabled"), "Value"=TRUE ("LimitToSpecificProviderTypeOfSameType(True)")) -> ()  [unwired: 2 in, 2 out]
            n99 = property on="_MethodLocation" class="MCListbox (strict)"("TopLeft"=cluster{"Row":u32, "Column":u32} {"Row"=0, "Column"=0} ("Top Left Visible Cell")) -> ()  [unwired: 2 in, 2 out]
            n100 = Unbundle(T23 {"Left"=329, "Top"=250, "Right"=1119, "Bottom"=765} ("Front Panel Window:Panel Bounds")) -> ("Left"=w150:i16, "Top"=w148:i16, "Right"=w151:i16, "Bottom"=w149:i16)
            n101 = property class="VI"() -> ("Front Panel.PanelBounds"=w145:T23)  [unwired: 2 in, 2 out]
            n102 = Bundle By Name(cluster=w164, "FolderType"=w156, "FolderNames"=w160, "FolderPath"=w158, "ClassName"=w97, "AF"=w104, "ActorVersion"=w106, "MethodCaptionName"=w101, "Interface"=w92) -> (w166:T17)
            n103 = property on="_DubMethodName" class="Str"("Visible"=w139) -> ()  [unwired: 2 in, 2 out]
            n104 = property on="_MethodLocation" class="MCListbox (strict)"("DisabledEnum"=w117) -> ()  [unwired: 2 in, 2 out]
            n105 = Unbundle(w145) -> ("Left"=w144:i16, "Top"=w143:i16)  [unwired: 2 out]
            n106 = Subtract(x=w149, y=w148) -> (x-y=w146:i16)
            n107 = Subtract(x=w151, y=w150) -> (x-y=w147:i16)
            n108 = Add(x=w144, y=w147) -> (x+y=w142:i16)
            n109 = Add(x=w143, y=w146) -> (x+y=w141:i16)
            n110 = local write "_MethodDescription"(w112) -> ()
            n111 = local write "_IconSearchText"(w112) -> ()
            n112 = Bundle(cluster=w145, "Left"=w144, "Top"=w143, "Right"=w142, "Bottom"=w141) -> (w140:T23)
            n113 = local write "_IconSize"(T20."Full" ("_IconSize")) -> ()
            n114 = property class="VI"("Front Panel.PanelBounds"=w140) -> (error out=w95:errorcluster)  [unwired: 2 in, 1 out]
            n115 = property on="_Method" class="LstBox (strict)"("Selection Mode"=1) -> ()  [unwired: 2 in, 2 out]
            n116 = property on="_Method" class="LstBox (strict)"("Top Row"=u8 0 ("Disabled")) -> ()  [unwired: 2 in, 2 out]
            n117 = local write "_Method"(i32[] [0] ("_Method")) -> ()
          }
          frame "GetTemplates" {
            n118 = call <resource>:"GetAllMethodsTypesForClass.vi"("ClassWriterNative"=w307, "ClassItemRefIn"=w304, "error in"=w306) -> ("DesignPattern"=w305:T10[], "NormalMethods"=w300:T12[], "OverrideMethods"=w303:T12[], "PropertyMethods"=w302:T12[], "ConnectorPaneHeight"=w299:i32[], "TemplateSettings"=w296:T16, "PropertyNodeMethods"=w298:T12[], "error out"=w280:errorcluster)  [unwired: 4 in, 1 out]
            n119 = Unbundle By Name(w296) -> ("OnlyNormalMethod"=w295:bool, "DynamicDispatch"=w291:enum8{"False", "True", "Mixed"}, "MustOverride"=w284:enum8{"False", "True", "Mixed"}, "MustCallParent"=w283:enum8{"False", "True", "Mixed"}, "OnlyPublic"=w282:bool)
            n120 = case shown="False" w282 {
              tunnel: [w313 w314] -> w281
              tunnel: [T19."Enabled" ("Disabled") w314] -> w278
              frame False {
                n121 = property on="_MethodLocation" class="MCListbox (strict)"() -> ("DisabledEnum"=w313:T19)  [unwired: 2 in, 2 out]
              }
              frame True {
                w314 = T19."Disabled and Grayed Out" ("Disabled")
              }
            }
            n122 = Array Size(array=w298) -> (size(s)=w297:i32)
            n123 = case shown="False" w295 {
              tunnel: w297 -> [w336 _]
              tunnel: [w335 T19."Enabled" ("Disabled")] -> w294
              tunnel: [T19."Enabled" ("Disabled") T19."Disabled and Grayed Out" ("Disabled")] -> w293
              tunnel: [T2."Normal Method" ("_MethodType") T2."Normal Method" ("_MethodType")] -> w292
              frame False {
                n124 = case shown="0" w336 {
                  tunnel: [T19."Enabled" ("Disabled") T19."Disabled and Grayed Out" ("Disabled")] -> w335
                  frame Default {
                  }
                  frame 0 {
                  }
                }
              }
              frame True {
              }
            }
            n125 = property on="_MethodLocation" class="MCListbox (strict)"("DisabledEnum"=w281) -> ()  [unwired: 2 in, 2 out]
            n126 = property on="_Visibility" class="RadioBtnsControl (strict)"("Disabled"=w278, "Value"=T7."Public" ("_Visibility")) -> ()  [unwired: 2 in, 2 out]
            n127 = for {
              tunnel: w300 -> [w344] mode=indexing
              tunnel: [w345] -> w301 mode=indexing
              tunnel: [w343] -> w276 mode=indexing
              tunnel: [w342] -> w277 mode=indexing
              n128 = Unbundle(w344) -> ("Name"=w343:string, "Path"=w342:path)  [unwired: 3 out]
              n129 = case shown="\"\"" w343 {
                tunnel: [0 -1] -> w345
                frame Default {
                }
                frame "" {
                }
              }
            }
            n130 = case shown="\"Mixed\"" w291 {
              tunnel: [T19."Enabled" ("Disabled") T19."Disabled and Grayed Out" ("Disabled") T19."Disabled and Grayed Out" ("Disabled")] -> w290
              tunnel: [TRUE TRUE FALSE] -> w289
              frame "Mixed" {
              }
              frame "True" {
              }
              frame "False" {
              }
            }
            n131 = case shown="\"Mixed\"" w284 {
              tunnel: [T19."Enabled" ("Disabled") T19."Disabled and Grayed Out" ("Disabled") T19."Disabled and Grayed Out" ("Disabled")] -> w287
              tunnel: [FALSE TRUE FALSE] -> w288
              frame "Mixed" {
              }
              frame "True" {
              }
              frame "False" {
              }
            }
            n132 = case shown="\"Mixed\"" w283 {
              tunnel: [T19."Enabled" ("Disabled") T19."Disabled and Grayed Out" ("Disabled") T19."Disabled and Grayed Out" ("Disabled")] -> w286
              tunnel: [FALSE TRUE FALSE] -> w285
              frame "Mixed" {
              }
              frame "True" {
              }
              frame "False" {
              }
            }
            n133 = property on="_Method" class="LstBox (strict)"("Item Names"=w276, "Item Symbols"=w301) -> ()  [unwired: 2 in, 2 out]
            n134 = Bundle By Name(cluster=w275, "DesignPatterns"=w305, "NormalMethods"=w300, "OverrideMethods"=w303, "PropertyMethods"=w302, "MethodVIs"=w277, "MethodItemNames"=w276, "ConnectorPaneHeight"=w299, "PropertyNodeMethods"=w298, "TemplateSettings"=w296) -> (w309:T17)
            n135 = Array Size(array=w300) -> (size(s)=w308:i32)
            n136 = property on="_MethodType" class="RadioBtnsControl (strict)"("DisabledEnum"=w293, "Value"=w292) -> ()  [unwired: 2 in, 2 out]
            n137 = property on="_DynamicDispatch" class="Bool (strict)"("Disabled"=w290, "Value"=w289) -> ()  [unwired: 2 in, 2 out]
            n138 = property on="_MustOverride" class="Bool (strict)"("Disabled"=w287, "Value"=w288) -> ()  [unwired: 2 in, 2 out]
            n139 = property on="_MustCallParent" class="Bool (strict)"("Disabled"=w286, "Value"=w285) -> ()  [unwired: 2 in, 2 out]
            n140 = Unbundle By Name(w275) -> ("Interface"=w274:bool)
            n141 = case shown="1.." w308 {
              tunnel: ["Exit" "UpdateScopeList"] -> w310
              frame 0, Default {
                n142 = One Button Dialog(message="No method templates where found for this class" ("format string")) -> ()  [unwired: 1 in, 1 out]
              }
              frame 1.. {
              }
            }
            n143 = case shown="False" w274 {
              tunnel: w294 -> [w311 _]
              frame False {
                n144 = property on="Property Node" class="Bool (strict)"("DisabledEnum"=w311) -> ()  [unwired: 2 in, 2 out]
              }
              frame True {
              }
            }
          }
          frame "UpdateScopeList" {
            n145 = property class="LVClassLibrary"(reference=w365) -> ("Path"=w360:path)  [unwired: 1 in, 2 out]
            n146 = Unbundle By Name(w357) -> ("FolderNames"=w363:string[], "FolderPath"=w364:path[], "FolderType"=w362:T31)
            n147 = Strip Path(path=w360) -> (stripped path=w359:path)  [unwired: 1 out]
            n148 = for {
              tunnel: w364 -> [w380] mode=indexing
              tunnel: w359 -> [w379]
              tunnel: w363 -> [w366] mode=indexing
              tunnel: w362 -> [w370] mode=indexing
              tunnel: [w372] -> w354 mode=indexing
              tunnel: [w367] -> w355 mode=indexing
              n149 = Path To String(path=w379) -> (string=w377:string)
              n150 = Path To String(path=w380) -> (string=w378:string)
              n151 = Search and Replace String(input string=w378, search string=w377) -> (result string=w376:string)  [unwired: 6 in, 3 out]
              n152 = case shown="Default" w370 {
                selector: w370 -> [_ w383]
                tunnel: ["<any scope>" w382] -> w369
                frame "invalid scope" {
                }
                frame Default {
                  n153 = Format Into String(w383) -> (resulting string=w382:string)  [unwired: 3 in, 1 out]
                }
              }
              n154 = String Subset(string=w376, offset (0)=1) -> (substring=w368:string)  [unwired: 1 in]
              n155 = String To Path(string=w368) -> (path=w367:path)
              n156 = Empty String/Path?(string/path=w368) -> (empty?=w374:bool)
              n157 = Select(t=".", s=w374, f=w368) -> (s? t:f=w371:string)
              n158 = Build Array(w366, w371, w369) -> (w372:string[])
            }
            n159 = Bundle By Name(cluster=w357, "RelFolderPath"=w355, "MethodLocation"=w354) -> (w356:T17)
            n160 = property on="_MethodLocation" class="MCListbox (strict)"("ItemNames"=w354, "Value"=0 ("Method Location")) -> ()  [unwired: 2 in, 2 out]
            n161 = call <resource>:"GDSString_AddStatesToQueue.vi"("EmptyQueueNextState"="GetCurrentClassMethods", "State(s) in (\"\")"=w351) -> ("States Out"=w352:string)  [unwired: 13 in]
          }
          frame "GetCurrentClassMethods" {
            n162 = invoke class="LVClassLibrary" method="Get All Descendents"(reference=w387, error in=w385, "Type"="VI") -> (error out=w384:errorcluster, "All Descendents"=w388:refnum<vi>[])  [unwired: 4 in, 5 out]
            n163 = for {
              tunnel: w388 -> [w402] mode=indexing
              tunnel: [w394] -> w386 mode=indexing
              n164 = property class="ProjectItem"(reference=w402) -> (reference out=w397:refnum<vi>, error out=w399:errorcluster, "Reference"=w396:refnum<vi>)  [unwired: 1 in]
              n165 = property class="VI"(reference=w396, error in=w399) -> (reference out=w400:refnum<vi>, error out=w401:errorcluster, "Name"=w395:string)
              n166 = Close Reference(reference=w400, error in (no error)=w401) -> (error out=w398:errorcluster)
              n167 = Close Reference(reference=w397, error in (no error)=w398) -> ()  [unwired: 1 out]
              n168 = Match Pattern(string=w395, regular expression=":") -> (after substring=w394:string)  [unwired: 1 in, 3 out]
            }
            n169 = Bundle By Name(cluster=w392, "ClassVIs"=w386) -> (w391:T17)
          }
          frame "GetClassColors" {
            w434 = u8 32 ("x")
            n170 = Unbundle By Name(w409) -> ("Interface"=w408:bool)
            n171 = call <resource>:"GDSLvClass_ReadClassColors.vi"("Library Refnum"=w413, "error in (no error)"=w444) -> ("LvClassIconSettings"=w425:T35, "error out"=w435:errorcluster)  [unwired: 12 in, 4 out]
            n172 = Unbundle By Name(w425) -> ("ColorProtected"=w422:u32, "ColorPrivate"=w423:u32, "ColorPublic"=w418:u32, "Frame"=w424:u32, "Frame thickness"=w421:u8, "Body Text"=w420:u32)
            n173 = case shown="False" w408 {
              tunnel: w435 -> [w445 w456]
              tunnel: w413 -> [w446 w455]
              tunnel: [w446 w454] -> w410
              tunnel: [_ w452] -> w407
              tunnel: [_ w451] -> w406
              tunnel: [_ w450] -> w405
              tunnel: [w445 w447] -> w404
              frame True {
              }
              frame False {
                n174 = property class="LVClassLibrary"(reference=w455, error in=w456) -> (reference out=w454:refnum<vi>, error out=w453:errorcluster, "Member Data"=w449:refnum<vi>)
                n175 = call <resource>:"GDSLvIcon_AnalyseViIcon.vi"("ViRef/LvCLassRef/LvLibRef/ViPath/2D_Image"=w449, "error in (no error)"=w453) -> ("ValidHeaderIcon"=w452:bool, "HeaderIcon"=w451:u8[][], "HeaderBkColor"=w450:u32, "error out"=w448:errorcluster)  [unwired: 5 in, 9 out]
                n176 = Close Reference(reference=w449, error in (no error)=w448) -> (error out=w447:errorcluster)
              }
            }
            n177 = Equal?(x=w418, y=w420) -> (x = y?=w431:bool)
            n178 = Bundle(FALSE, "ColorPublic"=w418) -> (w419:cluster{bool, "ColorPublic":u32})  [unwired: 1 in]
            n179 = Equal?(x=u32 0 ("Frame"), y=w418) -> (x = y?=w430:bool)
            n180 = local write "_BodyBk"(w419) -> ()
            n181 = Select(t=u32 16777215 ("Frame"), s=w430, f=u32 0 ("Frame")) -> (s? t:f=w426:u32)
            n182 = Select(t=w426, s=w431, f=w420) -> (s? t:f=w415:u32)
            n183 = Bundle(FALSE, "Body Text"=w415) -> (w414:cluster{bool, "Body Text":u32})  [unwired: 1 in]
            n184 = local write "_BodyText"(w414) -> ()
            n185 = case shown="False" w407 {
              tunnel: w406 -> [_ w473]
              tunnel: w405 -> [_ w472]
              tunnel: [w459 w473] -> w412
              tunnel: [w460 w472] -> w411
              tunnel: w404 -> [w466 w471]
              tunnel: w410 -> [w465 _]
              tunnel: [w464 w471] -> w403
              frame False {
                n186 = call <resource>:"GDSLvIcon_AnalyseViIcon.vi"("ViRef/LvCLassRef/LvLibRef/ViPath/2D_Image"=w465, "error in (no error)"=w466) -> ("ValidHeaderIcon"=w463:bool, "HeaderIcon"=w462:u8[][], "HeaderBkColor"=w461:u32, "BodyIcon"=w458:u8[][], "BodyBkColor"=w457:u32, "error out"=w464:errorcluster)  [unwired: 5 in, 7 out]
                n187 = case shown="False" w463 {
                  tunnel: w462 -> [_ w469]
                  tunnel: [w467 w470] -> w460
                  tunnel: w461 -> [_ w470]
                  tunnel: [w468 w469] -> w459
                  tunnel: w458 -> [w468 _]
                  tunnel: w457 -> [w467 _]
                  frame False {
                  }
                  frame True {
                  }
                }
              }
              frame True {
              }
            }
            n188 = Array Size(array=w412) -> (size(s)=w441:i32[])
            n189 = Multiply(x=w421, y=u8 2) -> (x*y=w437:u8)
            n190 = Index Array(array=w441) -> (element #1=w438:i32)  [unwired: 2 in, 1 out]
            n191 = Add(x=w438, y=w437) -> (x+y=w436:i32)
            n192 = Increment(x=w436) -> (x+1=w433:i32)
            n193 = Subtract(x=w434, y=w433) -> (x-y=w432:i32)
            n194 = Subtract(x=w434, y=w437) -> (x-y=w439:u8)
            n195 = Bundle By Name(cluster=w409, "ColorProtected"=w422, "ColorPrivate"=w423, "ColorPublic"=w418, "Frame"=w424, "Frame thickness"=w421, "HeaderBkColor"=w411, "HeaderIcon"=w412, "BodyIconHeight"=w432, "BodyIconWidth"=w439) -> (w443:T17)
          }
          frame "UpdateMethodSignatures" {
            w489 = 0  # Current
            w491 = string[] []  # SignatureText
            w492 = string[] []  # SignatureName
            n196 = call <resource>:"GOOP_GetGDSConfigFolder.vi"() -> ("GDSFolderPath"=w496:path)
            n197 = Build Path(base path=w496, name or relative path="MethodSignatures.xml") -> (appended path=w494:path)
            n198 = Read from Text File(file (use dialog)=w494) -> (text=w493:string)  [unwired: 3 in, 3 out]
            n199 = Bundle("SignatureName"=w492, "SignatureText"=w491, "Current"=w489) -> (w490:T36)  [unwired: 1 in]
            n200 = Unflatten From XML(xml string=w493, type=w490) -> (value=w488:T36)  [unwired: 1 in, 1 out]
            n201 = Unbundle By Name(w479) -> ("Signatures.Current"=w475:i32)
            n202 = Unbundle By Name(w488) -> ("SignatureName"=w483:string[], "Current"=w481:i32, "SignatureText"=w474:string[])
            n203 = Greater Or Equal To 0?(x=w475) -> (x >= 0?=w478:bool)
            n204 = Array Size(array=w483) -> (size(s)=w482:i32)
            n205 = Bundle By Name(cluster=w479, "Signatures"=w488) -> (w477:T17)
            n206 = Max & Min(x=w482, y=w481) -> (min(x,y)=w480:i32)  [unwired: 1 out]
            n207 = case shown="False" w478 {
              tunnel: w477 -> [w498 w501]
              tunnel: [w498 w500] -> w476
              tunnel: w475 -> [_ w499]
              frame False {
              }
              frame True {
                n208 = Bundle By Name(cluster=w501, "Signatures.Current"=w499) -> (w500:T17)
              }
            }
            n209 = Build Array (concatenate)("No signature", w483, string[] ["-", "Add signature"] ("array")) -> (w484:string[])
            n210 = case shown="1.." w480 {
              selector: w480 -> [_ w506]
              tunnel: w474 -> [_ w505]
              frame 0, Default {
              }
              frame 1.. {
                n211 = Decrement(x=w506) -> (x-1=w502:i32)
                n212 = Index Array(array=w505, index=w502) -> (element=w504:string)
                n213 = call <resource>:"UpdateMethodSignatureText.vi"("TagCodedStringIn"=w504) -> ("StringOut"=w503:string)  [unwired: 10 in]
                n214 = local write "_MethodDescription"(w503) -> ()
              }
            }
            n215 = property on="_MethodSignature" class="Ring (strict)"("Strings []"=w484, "Value"=w480) -> ()  [unwired: 2 in, 2 out]
          }
          frame "", "Idle" {
            (unwired) "Idle"
            (unwired) ""
            n216 = event shown="[1] \"_Method\": Mouse Enter;  \"_Method\": Mouse Leave" {
              selector: _ -> [_ _ _ _ _ _ _ _ _ _ _ _ _ _ _ _ _ _ _ _ _ _ _ _ _ _ _ _ _ _ _ _ _ _ _ _ _ _ _ _]
              dyn-events: _ -> [_ _ _ _ _ _ _ _ _ _ _ _ _ _ _ _ _ _ _ _ _ _ _ _ _ _ _ _ _ _ _ _ _ _ _ _ _ _ _ _]
              timeout: _ -> [_ _ _ _ _ _ _ _ _ _ _ _ _ _ _ _ _ _ _ _ _ _ _ _ _ _ _ _ _ _ _ _ _ _ _ _ _ _ _ _]
              tunnel: [w574 w599 w622 w674 w750 "Idle" w803 "ReadIcons" "DrawIcons:NoBusy" ("y") "GetImageData" ("y") w839 "Idle" ("t") "Idle" ("t") "UpdateIcon:2" ("y") w907 "Exit" "Exit" w961 w986 "UpdateIconFromParentMethod" "Idle" w1070 "Idle" "UpdateMethodSettings\nUpdateIcon" "UpdateIcon" w1374 "Idle" "Idle" w1447 "Idle" "UpdateIcon" "UpdateMethodSettings\nUpdateIcon" "UpdateIcon" w1546 "UpdateMethodSettings\nUpdateIcon" "Idle" w1635 "UpdateMethodSettings" ("y") "Idle" "Idle"] -> w526
              tunnel: [_ _ _ _ _ _ _ _ _ _ _ _ _ _ _ TRUE w951 _ _ _ _ _ _ _ _ _ _ _ _ _ _ _ _ _ _ _ _ _ _ _] -> w524
              tunnel: w512 -> [w573 _ w624 w669 w752 w797 _ _ _ w816 w834 w874 w882 w891 w905 _ _ _ _ w1037 w1056 _ _ w1135 _ w1376 w1432 w1439 w1446 w1471 _ w1487 _ w1545 w1549 w1584 w1614 _ _ _]
              tunnel: [_ _ _ _ _ _ _ _ _ _ _ _ _ _ _ _ _ "_CreateOpenClass" _ _ _ _ _ _ _ _ _ _ _ _ _ _ _ _ _ _ _ _ _ _] -> w523
              tunnel: w512 -> [w571 w605 w626 w672 w754 w801 w807 w810 w813 w819 w838 w877 w883 w889 w895 w946 w950 w962 w977 w1030 w1059 w1076 w1105 w1116 w1371 w1379 w1436 w1442 w1449 w1474 w1485 w1494 w1538 w1547 w1556 w1585 w1617 w1693 w1695 w1699]
              tunnel: [w570 w605 w625 w673 w753 w800 w807 w810 w813 w818 w837 w876 w883 w890 w895 w946 w950 w962 w976 w1030 w1055 w1075 w1105 w1115 w1371 w1378 w1435 w1441 w1448 w1473 w1483 w1494 w1538 w1547 w1556 w1585 w1616 w1693 w1695 w1699] -> w522
              tunnel: w520 -> [_ _ _ w675 _ _ _ _ _ _ _ _ _ _ _ _ _ _ _ _ _ _ _ _ _ _ _ _ _ _ _ _ _ _ _ _ _ _ _ _]
              tunnel: [_ _ _ _ w749 w796 _ _ _ w815 w835 w873 w880 _ _ _ _ _ _ w1028 _ _ _ _ _ _ _ w1438 w1445 w1470 _ _ _ w1541 _ w1583 _ _ _ _] -> w511
              tunnel: [w568 w604 w606 w671 w748 w795 w802 w808 w811 w814 w833 w872 w879 w886 w894 w945 w949 w953 w969 w1029 w1058 w1073 w1104 w1112 w1370 w1373 w1430 w1437 w1444 w1469 w1481 w1486 w1537 w1540 w1548 w1582 w1598 w1692 w1694 w1698] -> w510
              tunnel: w509 -> [w568 w604 w606 w670 w748 w795 w802 w808 w811 w814 w833 w872 w879 w886 w894 w945 w949 w953 w969 w1029 w1058 w1072 w1104 w1112 w1370 w1373 w1430 w1437 w1444 w1469 w1481 w1486 w1537 w1540 w1548 w1582 w1598 w1692 w1694 w1698]
              tunnel: w508 -> [_ w598 _ _ _ _ _ _ _ _ _ _ _ _ _ _ _ _ _ _ _ _ _ _ _ _ _ _ _ _ _ _ _ _ _ _ _ _ _ _]
              tunnel: [_ w598 _ _ _ _ _ _ _ _ _ _ _ _ _ _ _ _ _ _ _ _ _ _ _ _ _ _ _ _ _ _ _ _ _ _ _ _ _ _] -> _
              tunnel: w507 -> [_ _ _ _ _ _ _ _ _ _ _ _ _ _ _ _ _ _ _ _ _ w1071 _ _ _ _ _ _ _ _ _ _ _ _ _ _ _ _ _ _]
              event "_Method": Value Change {
                n217 = event-data() -> ()  [unwired: 1 in, 1 out]
                n218 = local read "_MethodType"() -> (w575:T2)
                n219 = case shown="\"Property Method\", \"Property Node\"" w575 {
                  selector: w575 -> [_ _ w585]
                  tunnel: "_Method" -> [_ _ w589]
                  tunnel: ["UpdateMethodTemplateImage" "UpdateMethodTemplateImage" "UpdateMethodTemplateImage\nUpdateIcon"] -> w574
                  tunnel: w573 -> [_ _ _]
                  tunnel: [_ _ w586] -> w569
                  frame "Normal Method" {
                  }
                  frame "Override Method" {
                  }
                  frame "Property Method", "Property Node" {
                    n220 = call <resource>:"BaseProvider_IniFileSettings.vi"() -> ("IniFileSettings"=w579:T37)  [unwired: 18 in, 1 out]
                    n221 = local read "_Property"() -> (w590:string[])
                    n222 = Unbundle By Name(w579) -> ("FileNamingOption"=w578:T38)
                    n223 = property on="_Method" class="LstBox (strict)"() -> ("Item Names"=w587:string[])  [unwired: 2 in, 2 out]
                    n224 = Equal?(x=w585, y=T2."Property Node") -> (x = y?=w581:bool)
                    n225 = call <resource>:"CreateMethodNames.vi"("_Method"=w589, "FileNamingOption"=w578, "_Property"=w590, "Item Names"=w587, "Use Read/Write"=w581) -> ("MethodNames"=w586:string[], "Attribute/PropertyNames"=w582:string[])
                    n226 = Index Array(array=w586) -> (element=w583:string)  [unwired: 1 in]
                    n227 = case shown="True" w581 {
                      tunnel: w583 -> [w591 _]
                      tunnel: [w591 w592] -> w580
                      tunnel: w582 -> [_ w596]
                      frame False {
                      }
                      frame True {
                        n228 = Array To Spreadsheet String(delimiter (Tab)="/", array=w596, 3:"%s" ("format string")) -> (spreadsheet string=w593:string)
                        n229 = call <vilib>:"Trim Whitespace.vi"("string"=w593) -> ("trimmed string"=w592:string)  [unwired: 1 in]
                      }
                    }
                    n230 = local write "_MethodIconName"(w583) -> ()
                    n231 = local write "_MethodName"(w580) -> ()
                  }
                }
                n232 = Bundle By Name(cluster=w571, "MethodNames"=w569) -> (w570:T17)
              }
              event "_Method": Mouse Enter; "_Method": Mouse Leave {
                n233 = event-data() -> ("Type"=w603:T24)  [unwired: 1 in]
                n234 = Equal?(x=lveventtype."Mouse Enter" ("y"), y=w603) -> (x = y?=w602:bool)
                n235 = property on="MethodTemplateImage" class="Pict"("Visible"=w602) -> ()  [unwired: 2 in, 2 out]
                n236 = Select(t="UpdateMethodTemplateImage", s=w602, f="Idle") -> (s? t:f=w599:string)
              }
              event Key Down? {
                (unwired) TRUE
                n237 = event-data() -> ("VKey"=w621:T39, "PlatMods.Ctrl"=w610:bool)  [unwired: 1 in]
                n238 = property on="_MethodName" class="Str"() -> ("Key Focus"=w607:bool)  [unwired: 2 in, 2 out]
                n239 = property on="_FontCompression" class="Enum (strict)"() -> ("Key Focus"=w620:bool)  [unwired: 2 in, 2 out]
                n240 = property on="_TextAlignment" class="Ring (strict)"() -> ("Key Focus"=w619:bool)  [unwired: 2 in, 2 out]
                n241 = property on="_IconSize" class="Ring (strict)"() -> ("Key Focus"=w618:bool)  [unwired: 2 in, 2 out]
                n242 = property on="_MethodLocation" class="MCListbox (strict)"() -> ("Key Focus"=w617:bool)  [unwired: 2 in, 2 out]
                n243 = property on="_OverrideMethods" class="LstBox (strict)"() -> ("Key Focus"=w616:bool)  [unwired: 2 in, 2 out]
                n244 = property on="_Property" class="Tree (strict)"() -> ("Key Focus"=w615:bool)  [unwired: 2 in, 2 out]
                n245 = property on="_MethodDescription" class="Str"() -> ("Key Focus"=w614:bool)  [unwired: 2 in, 2 out]
                n246 = property on="_MethodIconName" class="Str"() -> ("Key Focus"=w613:bool)  [unwired: 2 in, 2 out]
                n247 = property on="_Method" class="LstBox (strict)"() -> ("Key Focus"=w612:bool)  [unwired: 2 in, 2 out]
                n248 = property on="_MethodSignature" class="Ring (strict)"() -> ("Key Focus"=w611:bool)  [unwired: 2 in, 2 out]
                n249 = Unbundle By Name(w624) -> ("Offset.X"=w628:i32, "Offset.Y"=w627:i32)
                n250 = Compound Arithmetic op=OR(w620, w619, w618, w617, w616, w615, w615, w614, w613, w612, w611, w607) -> (w609:bool)
                n251 = Compound Arithmetic op=OR(w610, invert w609) -> (w608:bool)
                n252 = case shown="True" w608 {
                  tunnel: w626 -> [w630 w634]
                  tunnel: [w630 w638] -> w625
                  tunnel: w621 -> [_ w637]
                  tunnel: w627 -> [_ w631]
                  tunnel: w628 -> [_ w632]
                  tunnel: ["Idle" w636] -> w622
                  tunnel: [_ w635] -> w623
                  frame False {
                  }
                  frame True {
                    n253 = Bundle By Name(cluster=w634, "OldOffset.X"=w632, "OldOffset.Y"=w631) -> (w633:T17)
                    n254 = case shown="\"Left\"" w637 {
                      tunnel: w633 -> [w645 w647 w654 w661 w668]
                      tunnel: [w644 w647 w653 w660 w667] -> w638
                      tunnel: w631 -> [w643 _ w652 w658 w665]
                      tunnel: w632 -> [w641 _ w650 w659 w666]
                      tunnel: ["UpdateIcon" "Idle" "UpdateIcon" "UpdateIcon" "UpdateIcon"] -> w636
                      tunnel: [TRUE _ TRUE TRUE TRUE] -> w635
                      frame "Up" {
                        n255 = Decrement(x=w643) -> (x-1=w642:i32)
                        n256 = Bundle By Name(cluster=w645, "Offset.X"=w641, "Offset.Y"=w642) -> (w644:T17)
                      }
                      frame Default {
                      }
                      frame "Down" {
                        n257 = Increment(x=w652) -> (x+1=w651:i32)
                        n258 = Bundle By Name(cluster=w654, "Offset.X"=w650, "Offset.Y"=w651) -> (w653:T17)
                      }
                      frame "Left" {
                        n259 = Decrement(x=w659) -> (x-1=w657:i32)
                        n260 = Bundle By Name(cluster=w661, "Offset.X"=w657, "Offset.Y"=w658) -> (w660:T17)
                      }
                      frame "Right" {
                        n261 = Increment(x=w666) -> (x+1=w664:i32)
                        n262 = Bundle By Name(cluster=w668, "Offset.X"=w664, "Offset.Y"=w665) -> (w667:T17)
                      }
                    }
                  }
                }
                n263 = event-data("Discard?"=w623) -> ()  [unwired: 1 in, 1 out]
              }
              event "_MethodIcons": Value Change {
                n264 = event-data() -> ()  [unwired: 1 in, 1 out]
                n265 = disable-structure shown="Disabled" {
                  disable-tunnel: w675 -> [w681 _]
                  disable-tunnel: [w679 w721] -> w674
                  disable-tunnel: w672 -> [_ w723]
                  disable-tunnel: [_ w722] -> w673
                  disable-tunnel: [_ w720] -> w671
                  disable-tunnel: w670 -> [_ w719]
                  disable-tunnel: w669 -> [_ w718]
                  frame Disabled {
                    n266 = property class="VI"() -> ("Front Panel.WinBounds"=w677:T23)  [unwired: 2 in, 2 out]
                    n267 = Bundle By Name(cluster=T23 {"Left"=0, "Top"=0, "Right"=0, "Bottom"=0} ("y"), "Bottom"=w681) -> (w682:T23)
                    n268 = feedback #1() -> (w676:T23)  [unwired: 1 in]
                    n269 = feedback-in #1(w677) -> ()
                    n270 = case shown="True" {
                      selector: _ -> [_ _]
                      tunnel: w681 -> [_ _]
                      tunnel: w682 -> [w686 w699]
                      tunnel: [w685 w698] -> _
                      tunnel: ["Idle" "UpdateIconFolderList"] -> w679
                      tunnel: w677 -> [_ w696]
                      tunnel: w676 -> [w683 _]
                      frame False {
                        n271 = property class="VI"() -> ("Front Panel.WinBounds"=w687:T23)  [unwired: 2 in, 2 out]
                        n272 = Subtract(x=w687, y=w686) -> ()  [unwired: 1 out]
                        n273 = property class="VI"("Front Panel.WinBounds"=w683) -> (error out=w685:errorcluster)  [unwired: 2 in, 1 out]
                      }
                      frame True {
                        w688 = i16 50 ("y")
                        n274 = property class="App"() -> ("Disp.WkSpace"=w694:T23)  [unwired: 2 in, 2 out]
                        n275 = Add(x=w696, y=w699) -> (x+y=w692:T23)
                        n276 = Unbundle By Name(w692) -> ("Bottom"=w689:i16)
                        n277 = Unbundle By Name(w694) -> ("Bottom"=w690:i16)
                        n278 = Add(x=w689, y=w688) -> (x+y=w695:i16)
                        n279 = Greater?(x=w695, y=w690) -> (0:w693:bool)
                        n280 = case shown="True" w693 {
                          tunnel: w692 -> [w700 w709]
                          tunnel: [w700 w708] -> w691
                          tunnel: w690 -> [_ w705]
                          tunnel: w689 -> [_ w704]
                          tunnel: w688 -> [_ w701]
                          frame False {
                          }
                          frame True {
                            n281 = Subtract(x=w704, y=w705) -> (x-y=w703:i16)
                            n282 = Add(x=w703, y=w701) -> (x+y=w702:i16)
                            n283 = Bundle By Name(cluster=T23 {"Left"=0, "Top"=0, "Right"=0, "Bottom"=0} ("y"), "Top"=w702, "Bottom"=w702) -> (w706:T23)
                            n284 = Subtract(x=w709, y=w706) -> (x-y=w708:T23)
                          }
                        }
                        n285 = property class="VI"("Front Panel.WinBounds"=w691) -> (error out=w698:errorcluster)  [unwired: 2 in, 1 out]
                      }
                    }
                    n286 = local write "_IconName"("") -> ()
                  }
                  frame Enabled {
                    n287 = Unbundle By Name(w718) -> ("HeaderIcon"=w711:u8[][])
                    n288 = Unbundle By Name(w718) -> ("RowStart(0)"=w727:i32, "ImageRows(32)"=w728:i32, "Frame thickness"=w726:i32, "Frame"=w729:u32)
                    n289 = Unbundle By Name(w718) -> ("BodyIconHeight"=w732:i32, "BodyIconWidth"=w733:i32, "HeaderBkColor"=w734:u32, "Offset"=w740:cluster{"X":i32, "Y":i32}, "CurrentIcon"=w710:T40)
                    n290 = local read "_FontCompression"() -> (w715:enum16{"Auto", "On", "Off"})
                    n291 = local read "_MethodIconName"() -> (w717:string)
                    n292 = local read "_TextAlignment"() -> (w714:u16)
                    n293 = local read "_CapitalOnly"() -> (w716:bool)
                    n294 = local read "_BodyText"() -> (w713:T1)
                    n295 = local read "_BodyBk"() -> (w712:T1)
                    n296 = Unbundle By Name(w713) -> ("Color"=w730:u32)
                    n297 = Unbundle By Name(w712) -> ("Color"=w731:u32)
                    n298 = Bundle By Name(cluster=T25 {"HeaderIcon"=[], "RowStart(0)"=0, "ImageRows(32)"=32, "FrameThickness(1)"=1, "FrameColor"=0, "IconTextDataType"={"Text"="", "Allow Only Capital Chars"=FALSE, "Compression"=enum."Auto", "Alignment"=enum."Center"}, "BodyTextColor"=0, "BodyBackgroundColor"=0, "BodyIconHeight"=0, "BodyIconWidth"=0, "HeaderBackgroundColor"=0, "BodyIcon"=[[0, 0, 0, 0, 0, 0, 0, 0, 0, 0, 255, 255, 0, 0, 255, 0, 0, 0, 255, 0, 0, 0, 0, 0, 0, 0, 0, 0, 0, 0], [0, 0, 0, 0, 0, 0, 0, 0, 0, 255, 0, 0, 255, 0, 255, 0, 0, 0, 255, 0, 0, 0, 0, 0, 0, 0, 0, 0, 0, 0], [0, 0, 0, 0, 0, 0, 0, 0, 0, 255, 255, 255, 255, 0, 255, 0, 0, 0, 255, 0, 0, 0, 0, 0, 0, 0, 0, 0, 0, 0], [0, 0, 0, 0, 0, 0, 0, 0, 0, 255, 0, 0, 255, 0, 255, 0, 0, 0, 255, 0, 0, 0, 0, 0, 0, 0, 0, 0, 0, 0], [0, 0, 0, 0, 0, 0, 0, 0, 0, 255, 0, 0, 255, 0, 255, 255, 255, 0, 255, 255, 255, 0, 0, 0, 0, 0, 0, 0, 0, 0], [0, 0, 255, 0, 0, 0, 255, 0, 0, 255, 255, 0, 0, 255, 0, 0, 255, 0, 255, 255, 0, 255, 255, 0, 0, 0, 255, 255, 0, 0], [0, 255, 0, 255, 0, 255, 0, 255, 0, 255, 0, 255, 0, 255, 255, 0, 255, 0, 255, 0, 0, 255, 0, 255, 0, 255, 0, 0, 0, 0], [0, 255, 0, 0, 0, 255, 0, 255, 0, 255, 255, 0, 0, 255, 0, 255, 255, 0, 255, 255, 0, 255, 255, 0, 0, 0, 255, 0, 0, 0], [0, 255, 0, 255, 0, 255, 0, 255, 0, 255, 0, 255, 0, 255, 0, 0, 255, 0, 255, 0, 0, 255, 0, 255, 0, 0, 0, 255, 0, 0], [0, 0, 255, 0, 0, 0, 255, 0, 0, 255, 0, 255, 0, 255, 0, 0, 255, 0, 255, 255, 0, 255, 0, 255, 0, 255, 255, 0, 0, 0], [0, 255, 0, 0, 0, 255, 0, 0, 255, 0, 0, 255, 0, 255, 0, 0, 255, 0, 255, 255, 0, 0, 255, 0, 0, 255, 255, 255, 0, 255], [255, 0, 255, 0, 255, 0, 255, 0, 255, 255, 0, 255, 0, 255, 255, 0, 255, 0, 255, 0, 0, 255, 0, 255, 0, 0, 255, 0, 0, 255], [255, 0, 0, 0, 255, 0, 255, 0, 255, 0, 255, 255, 0, 255, 0, 255, 255, 0, 255, 255, 0, 255, 0, 0, 0, 0, 255, 0, 0, 255], [255, 0, 255, 0, 255, 0, 255, 0, 255, 0, 0, 255, 0, 255, 0, 0, 255, 0, 255, 0, 0, 255, 0, 255, 0, 0, 255, 0, 0, 255], [0, 255, 0, 0, 0, 255, 0, 0, 255, 0, 0, 255, 0, 255, 0, 0, 255, 0, 255, 255, 0, 0, 255, 0, 0, 0, 255, 0, 0, 255], [0, 0, 0, 0, 0, 0, 0, 0, 0, 0, 0, 0, 0, 0, 255, 0, 0, 0, 0, 0, 0, 0, 0, 0, 0, 0, 0, 0, 0, 0], [0, 0, 0, 0, 0, 0, 0, 0, 0, 0, 0, 0, 0, 255, 0, 0, 0, 0, 0, 0, 0, 0, 0, 0, 0, 0, 0, 0, 0, 0], [0, 0, 0, 0, 0, 0, 0, 0, 0, 0, 0, 0, 0, 255, 255, 0, 0, 0, 0, 0, 0, 0, 0, 0, 0, 0, 0, 0, 0, 0], [0, 0, 0, 0, 0, 0, 0, 0, 0, 0, 0, 0, 0, 255, 0, 255, 0, 0, 0, 0, 0, 0, 0, 0, 0, 0, 0, 0, 0, 0], [0, 0, 0, 0, 0, 0, 0, 0, 0, 0, 0, 0, 0, 0, 255, 0, 0, 0, 0, 0, 0, 0, 0, 0, 0, 0, 0, 0, 0, 0], [0, 0, 0, 0, 0, 0, 0, 0, 0, 0, 0, 0, 0, 0, 0, 0, 0, 0, 0, 0, 0, 0, 0, 0, 0, 0, 0, 0, 0, 0], [0, 0, 0, 0, 0, 0, 0, 0, 0, 0, 0, 0, 0, 0, 0, 0, 0, 0, 0, 0, 0, 0, 0, 0, 0, 0, 0, 0, 0, 0]], "Offset"={"X"=0, "Y"=0}, "CurrentIcon"={"BgIcon"=[], "BgIconOffset"={"X"=0, "Y"=0}, "BgIconMask"=[], "ColorsOkayforiconToBeOnTopOf"=[]}} ("IconInfo"), "HeaderIcon"=w711, "RowStart(0)"=w727, "ImageRows(32)"=w728, "FrameThickness(1)"=w726, "FrameColor"=w729, "IconTextDataType.Text"=w717, "IconTextDataType.Allow Only Capital Chars"=w716, "IconTextDataType.Compression"=w715, "IconTextDataType.Alignment"=w714, "BodyTextColor"=w730, "BodyBackgroundColor"=w731, "BodyIconHeight"=w732, "BodyIconWidth"=w733, "HeaderBackgroundColor"=w734, "Offset"=w740, "CurrentIcon"=w710) -> (w725:T25)
                    n299 = call <resource>:"GDSIconEditor_IconDialog.vi"("error in (no error)"=w719, "IconInfo"=w725) -> ("error out"=w720:errorcluster, "Icon exist"=w739:bool, "CurrentIcon"=w738:T40, "Cancelled"=w737:bool, "Offset"=w736:cluster{"X":i32, "Y":i32}, "BodyIcon"=w735:u8[][])  [unwired: 4 in]
                    n300 = case shown="False" w737 {
                      tunnel: w723 -> [w746 w747]
                      tunnel: [w745 w747] -> w722
                      tunnel: w735 -> [w744 _]
                      tunnel: w736 -> [w743 _]
                      tunnel: w738 -> [w742 _]
                      tunnel: w739 -> [_ _]
                      tunnel: ["Generate icon" _] -> w721
                      frame False {
                        n301 = Bundle By Name(cluster=w746, "BodyIcon"=w744, "Offset"=w743, "CurrentIcon"=w742) -> (w745:T17)
                      }
                      frame True {
                      }
                    }
                  }
                }
              }
              event Mouse Move {
                n302 = event-data() -> ("Coords"=w751:T14)  [unwired: 1 in]
                n303 = Unbundle By Name(w752) -> ("DraggingText"=w756:bool, "DraggingIcon"=w755:bool)
                n304 = Unbundle By Name(w752) -> ("OverrideMethod"=w749:path, "StartTextDraggingPos"=w757:T14)
                n305 = case shown="False" w755 {
                  tunnel: w754 -> [w763 w787]
                  tunnel: [w762 w786] -> w753
                  tunnel: w751 -> [w759 w782]
                  tunnel: w752 -> [w758 _]
                  tunnel: [w761 "UpdateIcon:2" ("y")] -> w750
                  tunnel: w756 -> [w764 _]
                  tunnel: w757 -> [w760 _]
                  frame False {
                    n306 = case shown="False" w764 {
                      tunnel: w763 -> [w766 w780]
                      tunnel: [w766 w779] -> w762
                      tunnel: ["Idle" "Generate icon"] -> w761
                      tunnel: w760 -> [_ w776]
                      tunnel: w759 -> [_ w777]
                      tunnel: w758 -> [_ w775]
                      frame False {
                      }
                      frame True {
                        n307 = Subtract(x=w777, y=w776) -> (x-y=w772:T14)
                        n308 = Unbundle By Name(w775) -> ("Offset.X"=w770:i32, "Offset.Y"=w769:i32)
                        n309 = Divide(x=w772, y=u8 4 ("f")) -> (x/y=w771:cluster{"Horizontal":dbl, "Vertical":dbl})
                        n310 = Unbundle By Name(w771) -> ("Horizontal"=w768:dbl, "Vertical"=w767:dbl)
                        n311 = Bundle By Name(cluster=w780, "Offset.X"=w770, "Offset.Y"=w769) -> (w774:T17)
                        n312 = Bundle By Name(cluster=w774, "Offset.X"=w768, "Offset.Y"=w767) -> (w779:T17)
                      }
                    }
                  }
                  frame True {
                    n313 = property on="DragIcon" class="Pict"() -> ("Draw Area Size"=w792:T18)  [unwired: 2 in, 2 out]
                    n314 = property on="_IconPreview" class="Pict"() -> ("Position"=w790:T29)  [unwired: 2 in, 2 out]
                    n315 = Divide(x=w792, y=2.0 ("Waveform Chart")) -> (x/y=w793:cluster{"Width":dbl, "Height":dbl})
                    n316 = Add(x=w790, y=T29 {"Left"=0, "Top"=16}) -> (x+y=w789:T29)
                    n317 = Subtract(x=w782, y=w793) -> (x-y=w781:cluster{dbl, dbl})
                    n318 = Subtract(x=w781, y=w789) -> (x-y=w784:cluster{dbl, dbl})
                    n319 = property on="DragIcon" class="Pict"("Position"=w781) -> ()  [unwired: 2 in, 2 out]
                    n320 = Divide(x=w784, y=u8 4 ("Disabled")) -> (x/y=w783:cluster{dbl, dbl})
                    n321 = Bundle By Name(cluster=w787, "BgIconOffset"=w783) -> (w786:T17)
                  }
                }
              }
              event Mouse Up; Mouse Leave {
                w798 = FALSE ("DraggingText")
                n322 = event-data() -> ()  [unwired: 1 in, 1 out]
                n323 = Unbundle By Name(w797) -> ("OverrideMethod"=w796:path)
                n324 = property on="DragIcon" class="Pict"("Visible"=w798) -> ()  [unwired: 2 in, 2 out]
                n325 = Bundle By Name(cluster=w801, "DraggingText"=w798) -> (w800:T17)
              }
              event "_Manage": Value Change {
                n326 = event-data() -> ()  [unwired: 1 in, 1 out]
                n327 = call <resource>:"GDSLvIcon_ManageIconFolderDialog.vi"() -> ("Cancelled"=w806:bool)  [unwired: 10 in, 1 out]
                n328 = Select(t="Idle", s=w806, f="UpdateIconFolderList" ("y")) -> (s? t:f=w803:string)
              }
              event "_Folders": Value Change {
                n329 = event-data() -> ()  [unwired: 1 in, 1 out]
              }
              event "_IconSearchText": Value Change {
                n330 = event-data() -> ()  [unwired: 1 in, 1 out]
              }
              event "DragIcon": Mouse Down {
                n331 = event-data() -> ("Coords"=w817:T14)  [unwired: 1 in]
                n332 = Unbundle By Name(w816) -> ("OverrideMethod"=w815:path)
                n333 = property on="DragIcon" class="Pict"() -> ("Draw Area Size"=w831:T18)  [unwired: 2 in, 2 out]
                n334 = Divide(x=w831, y=2) -> (x/y=w829:cluster{"Width":dbl, "Height":dbl})
                n335 = property on="_IconPreview" class="Pict"() -> ("Position"=w827:T29)  [unwired: 2 in, 2 out]
                n336 = Subtract(x=w817, y=w829) -> (x-y=w823:cluster{dbl, dbl})
                n337 = Add(x=w827, y=T29 {"Left"=0, "Top"=16}) -> (x+y=w826:T29)
                n338 = Subtract(x=w823, y=w826) -> (x-y=w824:cluster{dbl, dbl})
                n339 = Divide(x=w824, y=u8 4 ("Disabled")) -> (x/y=w822:cluster{dbl, dbl})
                n340 = property on="DragIcon" class="Pict"("Position"=w823, "Visible"=TRUE) -> ()  [unwired: 2 in, 2 out]
                n341 = Bundle By Name(cluster=w819, "DraggingIcon"=TRUE ("Draging"), "BgIconOffset"=w822) -> (w818:T17)
              }
              event "DragIcon", "Icons": Mouse Move {
                n342 = event-data() -> ("Coords"=w836:T14)  [unwired: 1 in]
                n343 = Unbundle By Name(w834) -> ("DraggingIcon"=w840:bool)
                n344 = Unbundle By Name(w834) -> ("OverrideMethod"=w835:path)
                n345 = case shown="False" w840 {
                  tunnel: w838 -> [w853 w871]
                  tunnel: [w852 w871] -> w837
                  tunnel: [w850 "Idle" ("t")] -> w839
                  tunnel: w836 -> [w848 _]
                  tunnel: w834 -> [w845 _]
                  frame False {
                    n346 = Unbundle By Name(w845) -> ("IconPos"=w854:T41)
                    n347 = property on="Icons" class="Pict"() -> ("Position"=w849:T29)  [unwired: 2 in, 2 out]
                    n348 = property on="Icons" class="Pict"() -> ("Origin"=w844:T30)  [unwired: 2 in, 2 out]
                    n349 = Subtract(x=w848, y=w849) -> (x-y=w843:T14)
                    n350 = Add(x=w844, y=w843) -> (x+y=w842:T14)
                    n351 = for {
                      tunnel: w854 -> [w864] mode=indexing
                      tunnel: w842 -> [w866]
                      tunnel: [w856] -> w851
                      tunnel: [w855] -> w847
                      i -> [w855]
                      stop <- w856 stop-if-true
                      n352 = Unbundle(w864) -> ("left"=w863:i16, "top"=w859:i16, "right"=w862:i16, "bottom"=w861:i16)
                      n353 = Unbundle(w866) -> ("Horizontal"=w865:i32, "Vertical"=w860:i32)
                      n354 = In Range and Coerce(upper limit=w862, x=w865, lower limit=w863) -> (In Range?=w857:bool)  [unwired: 1 out]
                      n355 = In Range and Coerce(upper limit=w861, x=w860, lower limit=w859) -> (In Range?=w858:bool)  [unwired: 1 out]
                      n356 = And(x=w857, y=w858) -> (x .and. y?=w856:bool)
                    }
                    n357 = Select(t=w847, s=w851, f=-1) -> (s? t:f=w841:i32)
                    n358 = case shown="True" w851 {
                      tunnel: ["Idle" ("t") "ShowDragIcon" ("t")] -> w850
                      frame False {
                        n359 = property on="DragIcon" class="Pict"("Visible"=FALSE) -> ()  [unwired: 2 in, 2 out]
                      }
                      frame True {
                      }
                    }
                    n360 = Bundle By Name(cluster=w853, "IconSelected"=w841) -> (w852:T17)
                  }
                  frame True {
                  }
                }
              }
              event "DragIcon": Mouse Up {
                w878 = FALSE ("Draging")
                n361 = event-data() -> ()  [unwired: 1 in, 3 out]
                n362 = Unbundle By Name(w874) -> ("OverrideMethod"=w873:path)
                n363 = Bundle By Name(cluster=w877, "DraggingIcon"=w878) -> (w876:T17)
                n364 = property on="DragIcon" class="Pict"("Visible"=w878) -> ()  [unwired: 2 in, 2 out]
              }
              event "DragIcon": Mouse Leave {
                n365 = event-data() -> ()  [unwired: 1 in, 1 out]
                n366 = Unbundle By Name(w882) -> ("OverrideMethod"=w880:path, "DraggingIcon"=w881:bool)
                n367 = case shown="False" w881 {
                  selector: w881 -> [w885 _]
                  frame False {
                    n368 = property on="DragIcon" class="Pict"("Visible"=w885) -> ()  [unwired: 2 in, 2 out]
                  }
                  frame True {
                  }
                }
              }
              event "FloodFillMask": Value Change {
                n369 = event-data() -> ()  [unwired: 1 in, 1 out]
                n370 = Unbundle By Name(w891) -> ("BgIcon"=w892:u8[][])
                n371 = call <resource>:"GDSIconEditor_CreateImageMask.vi"("Flood Fill"="FloodFillMask", "8-bit pixmap"=w892) -> ("Array"=w893:u8[])
                n372 = Bundle By Name(cluster=w889, "BgIconMask"=w893) -> (w890:T17)
              }
              event "_MethodSignature": Value Change {
                n373 = event-data() -> ("OldVal"=w904:u16)  [unwired: 1 in]
                n374 = Unbundle By Name(w905) -> ("Signatures.SignatureText"=w897:string[])  [unwired: 1 out]
                n375 = local read "_MethodDescription"() -> (w900:string)
                n376 = property on="_MethodSignature" class="Ring (strict)"() -> ("Strings []"=w911:string[])  [unwired: 2 in, 2 out]
                n377 = Decrement(x=w904) -> (x-1=w896:u16)
                n378 = Index Array(array=w897, index=w896) -> (element=w903:string)
                n379 = Greater Than 0?(x=w904) -> (x > 0?=w898:bool)
                n380 = Array Size(array=w911) -> (size(s)=w910:i32)
                n381 = call <resource>:"UpdateMethodSignatureText.vi"("TagCodedStringIn"=w903) -> ("StringOut"=w902:string)  [unwired: 10 in]
                n382 = Decrement(x=w910) -> (x-1=w909:i32)
                n383 = String Length(string=w902) -> (length=w901:i32)
                n384 = String Length(string=w900) -> (length=w899:i32)
                n385 = Equal?(x="_MethodSignature", y=w909) -> (x = y?=w908:bool)
                n386 = case shown="True" w908 {
                  tunnel: ["Idle" w942] -> w907
                  tunnel: "_MethodSignature" -> [w927 _]
                  tunnel: w901 -> [w925 _]
                  tunnel: w900 -> [w920 _]
                  tunnel: w899 -> [w926 _]
                  tunnel: w898 -> [w923 _]
                  tunnel: w897 -> [w921 _]
                  frame False {
                    n387 = Subtract(x=w926, y=w925) -> (x-y=w924:i32)
                    n388 = String Subset(string=w920, length (rest)=w924) -> (substring=w922:string)  [unwired: 1 in]
                    n389 = Select(t=w922, s=w923, f=w920) -> (s? t:f=w919:string)
                    n390 = String To Byte Array(string=w919) -> (unsigned byte array=w918:u8[])
                    n391 = Delete From Array(array=w918) -> (deleted portion=w917:u8)  [unwired: 2 in, 1 out]
                    n392 = Greater?(x=w917, y=u8 32) -> (0:w915:bool)
                    n393 = Select(t="\r", s=w915, f="") -> (s? t:f=w914:string)
                    n394 = case shown="0" w927 {
                      selector: w927 -> [w936 _]
                      tunnel: w921 -> [w935 _]
                      tunnel: w919 -> [w930 w938]
                      tunnel: w914 -> [w929 w937]
                      frame 1.., Default {
                        n395 = Decrement(x=w936) -> (x-1=w931:u16)
                        n396 = Index Array(array=w935, index=w931) -> (element=w934:string)
                        n397 = call <resource>:"UpdateMethodSignatureText.vi"("TagCodedStringIn"=w934) -> ("StringOut"=w933:string)  [unwired: 10 in]
                        n398 = Concatenate Strings(w930, w929, w933) -> (w932:string)
                        n399 = local write "_MethodDescription"(w932) -> ()
                      }
                      frame 0 {
                        n400 = Concatenate Strings(w938, w937) -> (w939:string)
                        n401 = local write "_MethodDescription"(w939) -> ()
                      }
                    }
                  }
                  frame True {
                    n402 = local write "_MethodSignature"(0) -> ()
                    n403 = call <resource>:"MethodSignatureDialogvi.vi"() -> ("Cancelled"=w941:bool)  [unwired: 11 in]
                    n404 = case shown="True" w941 {
                      tunnel: ["UpdateMethodSignatures" "Idle"] -> w942
                      frame False {
                      }
                      frame True {
                      }
                    }
                  }
                }
              }
              event "_Cancel": Value Change {
                n405 = event-data() -> ()  [unwired: 1 in, 2 out]
              }
              event Panel Close? {
                w951 = TRUE
                n406 = event-data() -> ()  [unwired: 1 in, 4 out]
                n407 = event-data("Discard?"=w951) -> ()  [unwired: 1 in, 1 out]
              }
              event "_CreateMethod", "_CreateOpenClass": Value Change {
                w957 = 2 ("y")
                n408 = event-data() -> ()  [unwired: 1 in, 2 out]
                n409 = local read "_Method"() -> (w963:i32[])
                n410 = local read "_Property"() -> (w960:string[])
                n411 = Array Size(array=w963) -> (size(s)=w959:i32)
                n412 = Array Size(array=w960) -> (size(s)=w958:i32)
                n413 = Greater Or Equal?(x=w959, y=w957) -> (x >= y?=w956:bool)
                n414 = Greater Or Equal?(x=w958, y=w957) -> (x >= y?=w955:bool)
                n415 = Or(x=w956, y=w955) -> (x .or. y?=w954:bool)
                n416 = case shown="True" w954 {
                  tunnel: ["Exit" "CreateMethodIcons"] -> w961
                  frame False {
                  }
                  frame True {
                    (unwired) "UpdateIcon:Quit"
                  }
                }
              }
              event "_Property": Value Change {
                n417 = event-data() -> ()  [unwired: 1 in, 1 out]
                n418 = property on="_Method" class="LstBox (strict)"() -> ("Item Names"=w973:string[])  [unwired: 2 in, 2 out]
                n419 = local read "_Method"() -> (w975:i32[])
                n420 = call <resource>:"BaseProvider_IniFileSettings.vi"() -> ("IniFileSettings"=w968:T37)  [unwired: 18 in, 1 out]
                n421 = local read "_MethodType"() -> (w972:T2)
                n422 = Unbundle By Name(w968) -> ("FileNamingOption"=w967:T38)
                n423 = Empty String/Path?(string/path="_Property") -> (empty?=w981:bool[])
                n424 = Index Array(array=w975) -> (element=w979:i32)  [unwired: 1 in]
                n425 = Equal?(x="_Property", y="ClassAttribute" ("Left Cell String(Main name)")) -> (x = y?=w982:bool[])
                n426 = Equal?(x="_Property", y="ObjectAttribute" ("Left Cell String(Main name)")) -> (x = y?=w983:bool[])
                n427 = Compound Arithmetic op=OR(w983, w982, w981) -> (w980:bool[])
                n428 = Index Array(array=w973, index=w979) -> (element=w987:string)
                n429 = Equal?(x=w972, y=T2."Property Node") -> (x = y?=w970:bool)
                n430 = Or Array Elements(Boolean array=w980) -> (logical OR=w978:bool)
                n431 = case shown="False" w978 {
                  tunnel: w987 -> [w996 _]
                  tunnel: [w995 "UpdateIcon"] -> w986
                  tunnel: w977 -> [w994 w1020]
                  tunnel: [w993 w1019] -> w976
                  tunnel: w975 -> [w992 _]
                  tunnel: "_Property" -> [w991 _]
                  tunnel: w973 -> [w990 _]
                  tunnel: w970 -> [w989 _]
                  tunnel: w967 -> [w988 _]
                  frame False {
                    n432 = case shown="Default" w996 {
                      tunnel: ["UpdateIcon" "Idle"] -> w995
                      tunnel: w994 -> [w1007 w1017]
                      tunnel: [w1006 w1016] -> w993
                      tunnel: w992 -> [w1004 _]
                      tunnel: w991 -> [w1003 _]
                      tunnel: w990 -> [w1002 _]
                      tunnel: w989 -> [w1001 _]
                      tunnel: w988 -> [w997 _]
                      frame Default {
                        n433 = call <resource>:"CreateMethodNames.vi"("_Method"=w1004, "FileNamingOption"=w997, "_Property"=w1003, "Item Names"=w1002, "Use Read/Write"=w1001) -> ("MethodNames"=w1005:string[], "Attribute/PropertyNames"=w998:string[])
                        n434 = Index Array(array=w1005) -> (element=w1000:string)  [unwired: 1 in]
                        n435 = case shown="True" w1001 {
                          tunnel: w1000 -> [w1009 _]
                          tunnel: [w1009 w1010] -> w999
                          tunnel: w998 -> [_ w1014]
                          frame False {
                          }
                          frame True {
                            n436 = Array To Spreadsheet String(delimiter (Tab)="/", array=w1014, 3:"%s" ("format string")) -> (spreadsheet string=w1011:string)
                            n437 = call <vilib>:"Trim Whitespace.vi"("string"=w1011) -> ("trimmed string"=w1010:string)  [unwired: 1 in]
                          }
                        }
                        n438 = local write "_MethodIconName"(w1000) -> ()
                        n439 = Bundle By Name(cluster=w1007, "MethodNames"=w1005) -> (w1006:T17)
                        n440 = local write "_MethodName"(w999) -> ()
                      }
                      frame "" {
                        n441 = Bundle By Name(cluster=w1017, "MethodNames"=string[] []) -> (w1016:T17)
                      }
                    }
                  }
                  frame True {
                    w1022 = "" ("Method Name")
                    n442 = local write "_MethodName"(w1022) -> ()
                    n443 = local write "_MethodIconName"(w1022) -> ()
                    n444 = Bundle By Name(cluster=w1020, "MethodNames"=string[] []) -> (w1019:T17)
                  }
                }
              }
              event "_OverrideMethods": Value Change {
                n445 = event-data() -> ()  [unwired: 1 in, 4 out]
                n446 = local read "_OverrideMethods"() -> (w1025:i32)
                n447 = Unbundle By Name(w1037) -> ("OverrideScope"=w1039:T31, "AllOverrideMethods"=w1041:path[], "OverrideMethodsIdx"=w1026:i32[])
                n448 = Unbundle By Name(w1037) -> ("ColorProtected"=w1036:u32, "ColorPrivate"=w1035:u32, "ColorPublic"=w1034:u32)
                n449 = Index Array(array=w1026, index=w1025) -> (element=w1024:i32)
                n450 = Index Array(array=w1041, index=w1024) -> (element=w1028:path)
                n451 = Index Array(array=w1039, index=w1024) -> (element=w1038:T22)
                n452 = case shown="\"invalid scope\", Default" w1038 {
                  tunnel: [w1042 w1043 w1044] -> w1031
                  tunnel: w1036 -> [_ w1043 _]
                  tunnel: w1034 -> [w1042 _ _]
                  tunnel: w1035 -> [_ _ w1044]
                  frame "invalid scope", Default {
                  }
                  frame "protected" {
                  }
                  frame "private" {
                  }
                }
                n453 = call <vilib>:"Get File Extension.vi"("file"=w1028) -> ("filename without extension"=w1027:string)  [unwired: 6 in, 4 out]
                n454 = local read "_BodyBk"() -> (w1032:T1)
                n455 = local write "_MethodName"(w1027) -> ()
                n456 = local write "_MethodIconName"(w1027) -> ()
                n457 = Bundle(cluster=w1032, "Color"=w1031) -> (w1033:T1)  [unwired: 1 in]
                n458 = call <vilib>:"Set Busy.vi"() -> ()  [unwired: 10 in, 2 out]
                n459 = local write "_BodyBk"(w1033) -> ()
              }
              event "Filter": Value Change {
                n460 = event-data() -> ()  [unwired: 1 in, 6 out]
                n461 = Unbundle By Name(w1056) -> ("OverrideMethodsNames"=w1051:string[])
                n462 = call <vilib>:"Trim Whitespace.vi"("string"="Filter") -> ("trimmed string"=w1049:string)  [unwired: 1 in]
                n463 = Empty String/Path?(string/path=w1049) -> (empty?=w1047:bool)
                n464 = Equal?(x=w1049, y="Filter name" ("InterfaceFilter")) -> (x = y?=w1046:bool)
                n465 = Or(x=w1047, y=w1046) -> (x .or. y?=w1045:bool)
                n466 = for {
                  tunnel: w1051 -> [w1063] mode=indexing
                  tunnel: w1049 -> [w1066]
                  tunnel: [w1063] -> w1050 mode=indexing if=w1061
                  tunnel: [w1062] -> w1053 mode=indexing if=w1061
                  tunnel: w1045 -> [w1060]
                  i -> [w1062]
                  n467 = Match Pattern(string=w1063, regular expression=w1066) -> (offset past match=w1065:i32)  [unwired: 1 in, 3 out]
                  n468 = Greater Or Equal To 0?(x=w1065) -> (x >= 0?=w1064:bool)
                  n469 = Or(x=w1064, y=w1060) -> (x .or. y?=w1061:bool)
                }
                n470 = property on="_OverrideMethods" class="LstBox (strict)"("Item Names"=w1050, "Top Row"=0) -> ()  [unwired: 2 in, 2 out]
                n471 = Bundle By Name(cluster=w1059, "OverrideMethodsIdx"=w1053) -> (w1055:T17)
              }
              event "_AddFolder": Value Change {
                n472 = event-data() -> ()  [unwired: 1 in, 6 out]
                n473 = call <resource>:"NewFolderDialog.vi"("error in"=w1072, "ClassItemRefIn"=w1071) -> ("error out"=w1073:errorcluster, "FolderNameOut"=w1069:string, "FolderSourceScope"=w1068:T22, "Cancelled"=w1074:bool, "FolderPath"=w1067:path)  [unwired: 5 in]
                n474 = case shown="False" w1074 {
                  tunnel: w1076 -> [w1088 w1103]
                  tunnel: [w1089 w1103] -> w1075
                  tunnel: [w1079 _] -> w1070
                  tunnel: w1069 -> [w1082 _]
                  tunnel: w1068 -> [w1084 _]
                  tunnel: w1067 -> [w1083 _]
                  frame False {
                    n475 = Unbundle By Name(w1088) -> ("FolderNames"=w1081:string[], "FolderPath"=w1086:path[], "FolderType"=w1085:T31)
                    n476 = call "Search Unsorted 1D Array.vim"("element"=w1082, "unsorted 1D array"=w1081) -> ("index of element"=w1080:i32)  [unwired: 9 in]
                    n477 = case shown="-1" w1080 {
                      tunnel: [w1092 w1102] -> w1087
                      tunnel: w1086 -> [w1091 w1101]
                      tunnel: [w1091 w1100] -> w1077
                      tunnel: w1085 -> [w1090 w1099]
                      tunnel: [w1090 w1098] -> w1078
                      tunnel: w1084 -> [_ w1097]
                      tunnel: w1083 -> [_ w1096]
                      tunnel: w1082 -> [_ w1095]
                      tunnel: w1081 -> [w1092 w1094]
                      tunnel: [_ "UpdateScopeList\nIdle"] -> w1079
                      frame 0, Default {
                      }
                      frame -1 {
                        n478 = Build Array (concatenate)(w1094, w1095) -> (w1102:string[])
                        n479 = Build Array (concatenate)(w1101, w1096) -> (w1100:path[])
                        n480 = Build Array (concatenate)(w1099, w1097) -> (w1098:T31)
                      }
                    }
                    n481 = Bundle By Name(cluster=w1088, "FolderNames"=w1087, "FolderPath"=w1077, "FolderType"=w1078) -> (w1089:T17)
                  }
                  frame True {
                  }
                }
              }
              event "_MethodDescription": Value Change {
                n482 = event-data() -> ()  [unwired: 1 in, 2 out]
              }
              event "_MethodName": Value Change {
                w1127 = TRUE ("ignore case? (F)")
                n483 = event-data() -> ()  [unwired: 1 in, 2 out]
                n484 = Unbundle By Name(w1135) -> ("ClassName"=w1118:string)
                n485 = local read "_MethodType"() -> (w1114:T2)
                n486 = case shown="Default" w1114 {
                  tunnel: [w1141 w1143] -> w1129
                  tunnel: "_MethodName" -> [w1141 w1142]
                  frame "Property Node" {
                  }
                  frame Default {
                    n487 = call <resource>:"GOOP300_RemoveUnwantedChars.vi"("StringIn"=w1142) -> ("StringOut"=w1143:string)  [unwired: 10 in]
                  }
                }
                n488 = Concatenate Strings(w1118, "[_ ]*" ("string")) -> (w1123:string)
                n489 = Match Pattern(string=w1129, regular expression="\\2E[Vv][Ii][Mm]*") -> (before substring=w1117:string, match substring=w1111:string)  [unwired: 1 in, 2 out]
                n490 = Concatenate Strings("^" ("string"), w1123) -> (w1126:string)
                n491 = Concatenate Strings(w1123, "$" ("string")) -> (w1122:string)
                n492 = To Lower Case(string=w1111) -> (all lower case string=w1110:string)
                n493 = xnode "Match Regular Expression"("input string"=w1117, "regular expression"=w1126, "ignore case? (F)"=w1127) -> ("before match"=w1132:string, "after match"=w1131:string)  [unwired: 3 in, 3 out]
                n494 = Concatenate Strings(w1132, w1131) -> (w1128:string)
                n495 = Match Pattern(string=w1110, regular expression="vim") -> (offset past match=w1108:i32)  [unwired: 1 in, 3 out]
                n496 = Greater Or Equal To 0?(x=w1108) -> (x >= 0?=w1107:bool)
                n497 = xnode "Match Regular Expression"("input string"=w1128, "regular expression"=w1122, "ignore case? (F)"=w1127) -> ("before match"=w1121:string, "after match"=w1120:string)  [unwired: 3 in, 3 out]
                n498 = case shown="True" w1107 {
                  tunnel: w1117 -> [_ w1136]
                  frame False {
                  }
                  frame True {
                    n499 = local write "_MethodName"(w1136) -> ()
                  }
                }
                n500 = property on=".vim" class="Bool (strict)"("Visible"=w1107, "Value"=w1107) -> ()  [unwired: 2 in, 2 out]
                n501 = Concatenate Strings(w1121, w1120) -> (w1113:string)
                n502 = case shown="\"Property Node\"" w1114 {
                  tunnel: w1113 -> [w1137 w1140]
                  tunnel: [w1137 w1138] -> _
                  frame Default {
                    n503 = local write "_MethodIconName"(w1137) -> ()
                  }
                  frame "Property Node" {
                    n504 = Match Pattern(string=w1140, regular expression="/") -> (before substring=w1138:string)  [unwired: 1 in, 3 out]
                  }
                }
                n505 = case shown="Default" w1114 {
                  tunnel: w1116 -> [w1144 w1147]
                  tunnel: [w1144 w1146] -> w1115
                  frame "Property Node" {
                  }
                  frame Default {
                    n506 = Bundle By Name(cluster=w1147, "MethodNames"=string[] []) -> (w1146:T17)
                  }
                }
              }
              event "_MethodIconName": Value Change {
                n507 = event-data() -> ()  [unwired: 1 in, 6 out]
              }
              event "_IconPreview": Mouse Down {
                w1392 = 4 ("y")
                n508 = event-data() -> ("Coords"=w1377:T14)  [unwired: 1 in]
                n509 = property on="_IconPreview" class="Pict"() -> ("Mouse"=w1381:T42)  [unwired: 2 in, 2 out]
                n510 = Unbundle By Name(w1376) -> ("IconDropped"=w1375:i32, "TextBounds"=w1383:T43)
                n511 = Unbundle(w1383) -> ("FirstRow"=w1385:i32, "FirstColumn"=w1386:i32, "LastRow"=w1384:i32, "LastColumn"=w1382:i32)
                n512 = Unbundle By Name(w1381) -> ("Mouse Position.X"=w1391:i32, "Mouse Position.Y"=w1389:i32)
                n513 = Divide(x=w1391, y=w1392) -> (x/y=w1393:dbl)
                n514 = Divide(x=w1389, y=w1392) -> (x/y=w1390:dbl)
                n515 = In Range and Coerce(upper limit=w1384, x=w1390, lower limit=w1385) -> (In Range?=w1387:bool)  [unwired: 1 out]
                n516 = In Range and Coerce(upper limit=w1382, x=w1393, lower limit=w1386) -> (In Range?=w1388:bool)  [unwired: 1 out]
                n517 = And(x=w1387, y=w1388) -> (x .and. y?=w1380:bool)
                n518 = case shown="False" w1380 {
                  tunnel: w1379 -> [w1396 w1422]
                  tunnel: [w1395 w1421] -> w1378
                  tunnel: w1377 -> [w1398 w1420]
                  tunnel: w1376 -> [_ w1419]
                  tunnel: w1375 -> [w1397 _]
                  tunnel: [w1394 "Idle"] -> w1374
                  frame False {
                    n519 = case shown="0.." w1397 {
                      selector: w1397 -> [_ w1402]
                      tunnel: w1396 -> [w1400 w1416]
                      tunnel: [w1400 w1415] -> w1395
                      tunnel: ["Idle" ("y") "ShowDragIcon:UpdateIcon" ("y")] -> w1394
                      tunnel: w1398 -> [_ w1401]
                      frame Default {
                      }
                      frame 0.. {
                        n520 = property on="DragIcon" class="Pict"() -> ("Draw Area Size"=w1413:T18)  [unwired: 2 in, 2 out]
                        n521 = Divide(x=w1413, y=2) -> (x/y=w1411:cluster{"Width":dbl, "Height":dbl})
                        n522 = Subtract(x=w1401, y=w1411) -> (x-y=w1405:cluster{dbl, dbl})
                        n523 = property on="_IconPreview" class="Pict"() -> ("Position"=w1409:T29)  [unwired: 2 in, 2 out]
                        n524 = property on="DragIcon" class="Pict"("Position"=w1405) -> ()  [unwired: 2 in, 2 out]
                        n525 = Add(x=w1409, y=T29 {"Left"=0, "Top"=16}) -> (x+y=w1408:T29)
                        n526 = Subtract(x=w1405, y=w1408) -> (x-y=w1406:cluster{dbl, dbl})
                        n527 = Divide(x=w1406, y=u8 4 ("Disabled")) -> (x/y=w1404:cluster{dbl, dbl})
                        n528 = Bundle By Name(cluster=w1416, "IconSelected"=w1402, "DraggingIcon"=TRUE ("Draging"), "BgIconOffset"=w1404) -> (w1415:T17)
                      }
                    }
                  }
                  frame True {
                    n529 = Unbundle By Name(w1419) -> ("Offset.X"=w1424:i32, "Offset.Y"=w1425:i32)
                    n530 = Bundle("X"=w1424, "Y"=w1425) -> (w1428:cluster{"X":i32, "Y":i32})  [unwired: 1 in]
                    n531 = Multiply(x=w1428, y=4) -> (x*y=w1429:cluster{"X":i32, "Y":i32})
                    n532 = Subtract(x=w1420, y=w1429) -> (x-y=w1427:T14)
                    n533 = Bundle By Name(cluster=w1422, "DraggingIcon"=FALSE, "DraggingText"=TRUE, "StartTextDraggingPos"=w1427) -> (w1421:T17)
                  }
                }
              }
              event "_IconPreview": Mouse Up {
                w1433 = FALSE ("DraggingText")
                n534 = event-data() -> ()  [unwired: 1 in, 3 out]
                n535 = Unbundle By Name(w1432) -> ("IconSelected"=w1431:i32)
                n536 = Bundle By Name(cluster=w1436, "IconDropped"=w1431, "DraggingText"=w1433, "DraggingIcon"=w1433, "Moving"=w1433) -> (w1435:T17)
                n537 = property on="DragIcon" class="Pict"("Visible"=w1433) -> ()  [unwired: 2 in, 2 out]
              }
              event "_IconPreview": Mouse Leave {
                n538 = event-data() -> ()  [unwired: 1 in, 1 out]
                n539 = Unbundle By Name(w1439) -> ("OverrideMethod"=w1438:path)
                n540 = Bundle By Name(cluster=w1442, "DraggingText"=FALSE) -> (w1441:T17)
              }
              event "_IconPreview": Mouse Move {
                n541 = event-data() -> ("Coords"=w1450:T14)  [unwired: 1 in]
                n542 = Unbundle By Name(w1446) -> ("DraggingText"=w1452:bool)
                n543 = Unbundle By Name(w1446) -> ("OverrideMethod"=w1445:path)
                n544 = Unbundle By Name(w1446) -> ("StartTextDraggingPos"=w1451:T14)
                n545 = case shown="False" w1452 {
                  tunnel: w1449 -> [w1454 w1468]
                  tunnel: [w1454 w1467] -> w1448
                  tunnel: ["Idle" "UpdateIcon"] -> w1447
                  tunnel: w1451 -> [_ w1464]
                  tunnel: w1450 -> [_ w1465]
                  tunnel: w1446 -> [_ w1463]
                  frame False {
                  }
                  frame True {
                    n546 = Subtract(x=w1465, y=w1464) -> (x-y=w1460:T14)
                    n547 = Unbundle By Name(w1463) -> ("Offset.X"=w1458:i32, "Offset.Y"=w1457:i32)
                    n548 = Divide(x=w1460, y=u8 4 ("f")) -> (x/y=w1459:cluster{"Horizontal":dbl, "Vertical":dbl})
                    n549 = Unbundle By Name(w1459) -> ("Horizontal"=w1456:dbl, "Vertical"=w1455:dbl)
                    n550 = Bundle By Name(cluster=w1468, "OldOffset.X"=w1458, "OldOffset.Y"=w1457) -> (w1462:T17)
                    n551 = Bundle By Name(cluster=w1462, "Offset.X"=w1456, "Offset.Y"=w1455) -> (w1467:T17)
                  }
                }
              }
              event "_IconPreview": Mouse Enter {
                n552 = event-data() -> ()  [unwired: 1 in, 1 out]
                n553 = Unbundle By Name(w1471) -> ("OverrideMethod"=w1470:path)
                n554 = Unbundle By Name(w1471) -> ("DraggingIcon"=w1476:bool, "IconDropped"=w1475:i32)
                n555 = case shown="True" w1476 {
                  tunnel: w1474 -> [w1479 w1480]
                  tunnel: [w1478 w1480] -> w1473
                  tunnel: w1475 -> [w1477 _]
                  frame False {
                    n556 = Bundle By Name(cluster=w1479, "IconSelected"=w1477) -> (w1478:T17)
                  }
                  frame True {
                  }
                }
              }
              event "_IconSize", "_TextAlignment": Value Change {
                n557 = event-data() -> ()  [unwired: 1 in, 6 out]
                n558 = Bundle By Name(cluster=w1485, "Offset"=cluster{"X":i32, "Y":i32} {"X"=0, "Y"=0}) -> (w1483:T17)
              }
              event "_MethodLocation": Value Change {
                (unwired) T19."Disabled and Grayed Out" ("Disabled")
                n559 = event-data() -> ()  [unwired: 1 in, 2 out]
                n560 = Unbundle By Name(w1487) -> ("ColorPublic"=w1500:u32, "ColorPrivate"=w1499:u32, "ColorProtected"=w1498:u32, "AF"=w1490:bool)
                n561 = Unbundle By Name(w1487) -> ("FolderType"=w1505:T31)
                n562 = Index Array(array=w1505, index="_MethodLocation") -> (element=w1503:T22)
                n563 = case shown="\"private\"" w1503 {
                  tunnel: [T19."Enabled" ("Disabled") T19."Disabled and Grayed Out" ("Disabled") T19."Disabled and Grayed Out" ("Disabled") T19."Disabled and Grayed Out" ("Disabled") T19."Disabled and Grayed Out" ("Disabled")] -> w1502
                  tunnel: [T7."Public" ("_Visibility") T7."Public" ("_Visibility") T7."Community" ("_Visibility") T7."Private" ("_Visibility") T7."Protected" ("_Visibility")] -> w1501
                  tunnel: w1500 -> [w1516 w1521 w1526 _ _]
                  tunnel: [w1516 w1521 w1526 w1531 w1536] -> w1495
                  tunnel: w1499 -> [_ _ _ w1531 _]
                  tunnel: w1498 -> [_ _ _ _ w1536]
                  tunnel: [TRUE TRUE FALSE FALSE FALSE] -> w1489
                  tunnel: [T19."Enabled" ("Disabled") T19."Enabled" ("Disabled") T19."Disabled and Grayed Out" ("Disabled") T19."Disabled and Grayed Out" ("Disabled") T19."Disabled and Grayed Out" ("Disabled")] -> w1488
                  frame "invalid scope", Default {
                  }
                  frame "public" {
                  }
                  frame "community" {
                  }
                  frame "private" {
                  }
                  frame "protected" {
                  }
                }
                n564 = local read "_MethodType"() -> (w1491:T2)
                n565 = local read "_BodyBk"() -> (w1496:T1)
                n566 = case shown="Default" w1491 {
                  tunnel: w1488 -> [w1508 _]
                  tunnel: w1489 -> [w1507 _]
                  tunnel: [w1508 T19."Disabled and Grayed Out" ("Disabled")] -> w1493
                  tunnel: [w1507 _] -> w1492
                  frame Default {
                  }
                  frame "Override Method" {
                  }
                }
                n567 = property on="_Visibility" class="RadioBtnsControl (strict)"("Disabled"=w1502) -> ()  [unwired: 2 in, 2 out]
                n568 = Bundle(cluster=w1496, "Color"=w1495) -> (w1497:T1)  [unwired: 1 in]
                n569 = local write "_Visibility"(w1501) -> ()
                n570 = local write "_BodyBk"(w1497) -> ()
                n571 = case shown="True" w1490 {
                  tunnel: w1492 -> [_ w1511]
                  tunnel: w1493 -> [_ w1510]
                  frame False {
                  }
                  frame True {
                    n572 = property on="_AddMessageClass" class="Bool (strict)"("DisabledEnum"=w1510, "Value"=w1511) -> ()  [unwired: 2 in, 2 out]
                  }
                }
              }
              event "_FontCompression", "_CapitalOnly": Value Change {
                n573 = event-data() -> ()  [unwired: 1 in, 2 out]
              }
              event Value Change {
                n574 = event-data() -> ()  [unwired: 1 in, 6 out]
                n575 = Unbundle By Name(w1545) -> ("OverrideMethod"=w1541:path)
                n576 = Empty String/Path?(string/path=w1541) -> (empty?=w1544:bool)
                n577 = Select(t="UpdateIcon", s=w1544, f="UpdateIconFromParentMethod") -> (s? t:f=w1546:string)
              }
              event "_Visibility": Value Change {
                (unwired) T7."Community" ("_Visibility")
                n578 = event-data() -> ()  [unwired: 1 in, 2 out]
                n579 = Unbundle By Name(w1549) -> ("ColorProtected"=w1562:u32, "ColorPrivate"=w1560:u32, "ColorPublic"=w1561:u32, "AF"=w1550:bool)
                n580 = case shown="\"Private\"" "_Visibility" {
                  tunnel: [w1572 w1575 w1578 w1581] -> w1558
                  tunnel: w1562 -> [_ w1575 _ _]
                  tunnel: w1561 -> [w1572 _ _ w1581]
                  tunnel: w1560 -> [_ _ w1578 _]
                  tunnel: [T19."Enabled" ("Disabled") T19."Disabled and Grayed Out" ("Disabled") T19."Disabled and Grayed Out" ("Disabled") T19."Disabled and Grayed Out" ("Disabled")] -> w1555
                  tunnel: [TRUE FALSE FALSE FALSE] -> w1554
                  frame "Public", Default {
                  }
                  frame "Protected" {
                  }
                  frame "Private" {
                  }
                  frame "Community" {
                  }
                }
                n581 = local read "_MethodType"() -> (w1551:T2)
                n582 = case shown="Default" w1551 {
                  tunnel: w1555 -> [w1566 _]
                  tunnel: w1554 -> [w1565 _]
                  tunnel: [w1566 T19."Disabled and Grayed Out" ("Disabled")] -> w1553
                  tunnel: [w1565 _] -> w1552
                  frame Default {
                  }
                  frame "Override Method" {
                  }
                }
                n583 = local read "_BodyBk"() -> (w1557:T1)
                n584 = Bundle(cluster=w1557, "Color"=w1558) -> (w1559:T1)  [unwired: 1 in]
                n585 = local write "_BodyBk"(w1559) -> ()
                n586 = case shown="True" w1550 {
                  tunnel: w1552 -> [_ w1569]
                  tunnel: w1553 -> [_ w1568]
                  frame False {
                  }
                  frame True {
                    n587 = property on="_AddMessageClass" class="Bool (strict)"("DisabledEnum"=w1568, "Value"=w1569) -> ()  [unwired: 2 in, 2 out]
                  }
                }
              }
              event Mouse Enter; Mouse Leave {
                n588 = event-data() -> ("Type"=w1589:T24, "CtlRef"=w1594:refnum<vi>)  [unwired: 1 in, 1 out]
                n589 = Unbundle By Name(w1584) -> ("OverrideMethod"=w1583:path)
                n590 = Equal?(x=w1589, y=lveventtype."Mouse Enter") -> (x = y?=w1587:bool)
                n591 = property class="Clust (strict)"(reference=w1594) -> (reference out=w1593:refnum<vi>, error out=w1592:errorcluster, "Value"=w1591:T44)  [unwired: 1 in]
                n592 = Bundle By Name(cluster=w1591, "Decal"=w1587) -> (w1590:T44)
                n593 = property class="Clust (strict)"(reference=w1593, error in=w1592, "Value"=w1590) -> ()  [unwired: 2 out]
              }
              event "_MethodType": Value Change {
                (unwired) T23 {"Left"=329, "Top"=250, "Right"=1087, "Bottom"=690} ("Front Panel Window:Panel Bounds")
                # "width = 1108"
                n594 = event-data() -> ("OldVal"=w1604:T2, "NewVal"=w1602:T2)  [unwired: 1 in]
                n595 = Unbundle By Name(w1614) -> ("AF"=w1613:bool, "MethodCaptionName"=w1601:string, "MethodLocation"=w1603:string[][])
                n596 = case shown="\"Property Node\"" w1604 {
                  tunnel: w1603 -> [_ w1641]
                  frame Default {
                  }
                  frame "Property Node" {
                    n597 = property on="_MethodLocation" class="MCListbox (strict)"("ItemNames"=w1641, "Value"=0 ("_MethodLocation")) -> ()  [unwired: 2 in, 2 out]
                  }
                }
                n598 = local read "_Visibility"() -> (w1612:T7)
                n599 = case shown="\"Property Method\"" "_MethodType" {
                  tunnel: [w1661 w1670 w1679 w1690] -> w1623
                  tunnel: T23 {"Left"=329, "Top"=250, "Right"=1437, "Bottom"=775} ("Front Panel Window:Panel Bounds") -> [_ w1670 w1679 w1690]
                  tunnel: T23 {"Left"=329, "Top"=250, "Right"=1119, "Bottom"=775} ("Front Panel Window:Panel Bounds") -> [w1661 _ _ _]
                  tunnel: ["Idle" "UpdateMethodSettings\nUpdateOverRideMethods" "UpdateProperties" "UpdateProperties"] -> w1635
                  tunnel: w1614 -> [w1659 w1668 w1677 w1688]
                  tunnel: [w1657 w1664 w1675 w1686] -> w1621
                  tunnel: [_ u8 2 ("Disabled") _ _] -> w1620
                  tunnel: [_ TRUE _ _] -> w1619
                  tunnel: [1 ("Selection Mode") 1 ("Selection Mode") 3 ("Selection Mode") 3 ("Selection Mode")] -> w1618
                  tunnel: [TRUE ("LimitToSpecificProviderTypeOfSameType(True)") FALSE ("LimitToSpecificProviderTypeOfSameType(True)") TRUE ("LimitToSpecificProviderTypeOfSameType(True)") TRUE ("LimitToSpecificProviderTypeOfSameType(True)")] -> w1608
                  tunnel: [T19."Enabled" ("Disabled") T19."Disabled and Grayed Out" ("Disabled") T19."Enabled" ("Disabled") T19."Enabled" ("Disabled")] -> w1609
                  tunnel: [w1653 _ FALSE FALSE] -> w1605
                  frame "Normal Method", Default {
                    n600 = local read "_MethodName"() -> (w1654:string)
                    n601 = Unbundle By Name(w1659) -> ("AF"=w1653:bool, "NormalMethods"=w1657:T12[])
                    n602 = property on="_MethodName" class="Str"("Val(Sgnl)"=w1654) -> ()  [unwired: 2 in, 2 out]
                  }
                  frame "Override Method" {
                    n603 = Unbundle By Name(w1668) -> ("OverrideMethods"=w1664:T12[])
                  }
                  frame "Property Method" {
                    w1671 = "" ("Method Name")
                    n604 = Unbundle By Name(w1677) -> ("PropertyMethods"=w1675:T12[])
                    n605 = local write "_MethodName"(w1671) -> ()
                    n606 = local write "_MethodIconName"(w1671) -> ()
                  }
                  frame "Property Node" {
                    w1682 = "" ("Method Name")
                    n607 = Unbundle By Name(w1688) -> ("PropertyNodeMethods"=w1686:T12[])
                    n608 = local write "_MethodName"(w1682) -> ()
                    n609 = local write "_MethodIconName"(w1682) -> ()
                    n610 = property on="_MethodLocation" class="MCListbox (strict)"("ItemNames"=string[][] [["properties", "properties", "<any scope>"]] ("Item Names"), "Value"=0 ("_MethodLocation")) -> ()  [unwired: 2 in, 2 out]
                  }
                }
                n611 = Equal?(x=w1612, y=T7."Public" ("_Visibility")) -> (x = y?=w1610:bool)
                n612 = property on="_MethodName" class="Str"("Disabled"=w1620) -> ()  [unwired: 2 in, 2 out]
                n613 = case shown="False" w1610 {
                  tunnel: w1609 -> [_ w1644]
                  tunnel: w1608 -> [_ w1643]
                  tunnel: [T19."Disabled and Grayed Out" ("Disabled") w1644] -> w1607
                  tunnel: [_ w1643] -> w1606
                  frame False {
                  }
                  frame True {
                  }
                }
                n614 = local write "_AddMessageClass"(w1605) -> ()
                n615 = property class="VI"() -> ("Front Panel.PanelBounds"=w1628:T23)  [unwired: 2 in, 2 out]
                n616 = property on="_MethodsLlocationOverrideInfo" class="Str"("Visible"=w1619) -> ()  [unwired: 2 in, 2 out]
                n617 = Unbundle(w1623) -> ("Left"=w1633:i16, "Top"=w1631:i16, "Right"=w1634:i16, "Bottom"=w1632:i16)
                n618 = property on="_Method" class="LstBox (strict)"("Selection Mode"=w1618) -> ()  [unwired: 2 in, 2 out]
                n619 = case shown="\"Property Node\"" w1602 {
                  tunnel: w1601 -> [_ w1639]
                  tunnel: ["Property Name" ("MethodCaptionName") w1639] -> w1600
                  frame "Property Node" {
                  }
                  frame Default {
                  }
                }
                n620 = Unbundle(w1628) -> ("Left"=w1627:i16, "Top"=w1626:i16)  [unwired: 2 out]
                n621 = Subtract(x=w1632, y=w1631) -> (x-y=w1629:i16)
                n622 = Subtract(x=w1634, y=w1633) -> (x-y=w1630:i16)
                n623 = for {
                  tunnel: w1621 -> [w1649] mode=indexing
                  tunnel: [w1650] -> w1622 mode=indexing
                  tunnel: [w1648] -> w1596 mode=indexing
                  tunnel: [w1647] -> w1597 mode=indexing
                  n624 = Unbundle(w1649) -> ("Name"=w1648:string, "Path"=w1647:path)  [unwired: 3 out]
                  n625 = case shown="\"\"" w1648 {
                    tunnel: [0 -1] -> w1650
                    frame Default {
                    }
                    frame "" {
                    }
                  }
                }
                n626 = case shown="True" w1613 {
                  tunnel: w1606 -> [_ w1646]
                  tunnel: w1607 -> [_ w1645]
                  frame False {
                  }
                  frame True {
                    n627 = property on="_AddMessageClass" class="Bool (strict)"("DisabledEnum"=w1645, "Value"=w1646) -> ()  [unwired: 2 in, 2 out]
                  }
                }
                n628 = Add(x=w1627, y=w1630) -> (x+y=w1625:i16)
                n629 = Add(x=w1626, y=w1629) -> ()  [unwired: 1 out]
                n630 = local write ".vim"(FALSE (".vim")) -> ()
                n631 = Bundle(cluster=w1628, "Left"=w1627, "Top"=w1626, "Right"=w1625) -> (w1624:T23)  [unwired: 1 in]
                n632 = Bundle By Name(cluster=w1617, "MethodNames"=string[] [], "MethodVIs"=w1597, "MethodItemNames"=w1596) -> (w1616:T17)
                n633 = property class="VI"("Front Panel.PanelBounds"=w1624) -> ()  [unwired: 2 in, 2 out]
                n634 = property on="_MethodName" class="Str"("Caption.Text"=w1600) -> ()  [unwired: 2 in, 2 out]
                n635 = property on="_Method" class="LstBox (strict)"("Item Names"=w1596, "Item Symbols"=w1622) -> ()  [unwired: 2 in, 2 out]
              }
              event ".vim": Value Change {
                n636 = event-data() -> ()  [unwired: 1 in, 4 out]
              }
              event "Help": Value Change {
                n637 = event-data() -> ()  [unwired: 1 in, 2 out]
                n638 = call <resource>:"GOOP_HelpMain.vi"() -> ()  [unwired: 12 in]
              }
              event "_ShowContextHelp": Value Change {
                n639 = event-data() -> ("NewVal"=w1697:bool)  [unwired: 1 in]
                n640 = Control Help Window(1:w1697) -> ()  [unwired: 1 in]
              }
            }
            n641 = local read "_Property"() -> (w518:string[])
            n642 = Array Size(array=w518) -> (size(s)=w517:i32)
            n643 = Greater Or Equal?(x=w517, y=2) -> (x >= y?=w516:bool)
            n644 = Select(t=T19."Disabled and Grayed Out" ("Disabled"), s=w516, f=T19."Enabled" ("Disabled")) -> (s? t:f=w513:T19)
            n645 = property on="_MethodIconName" class="Str"("DisabledEnum"=w513) -> ()  [unwired: 2 in, 2 out]
            n646 = Unbundle By Name(w522) -> ("MethodNames"=w521:string[])
            n647 = stacked-sequence {
              tunnel: w526 -> [_]
              tunnel: w522 -> [w536]
              tunnel: w521 -> [w531]
              frame #0 {
                n648 = local read "_MethodType"() -> (w538:T2)
                n649 = Unbundle By Name(w536) -> ("ClassVIs"=w528:string[])
                n650 = local read "_MethodName"() -> (w527:string)
                n651 = local read "_MethodIconName"() -> (w540:string)
                n652 = local read "_Method"() -> (w539:i32[])
                n653 = Empty Array?(array=w531) -> (empty?=w533:bool)
                n654 = case shown="\"Override Method\"" w538 {
                  tunnel: [TRUE w557 w567] -> w537
                  frame "Normal Method", Default {
                  }
                  frame "Override Method" {
                    n655 = local read "_OverrideMethods"() -> (w558:i32)
                    n656 = Greater Or Equal To 0?(x=w558) -> (x >= 0?=w557:bool)
                  }
                  frame "Property Method", "Property Node" {
                    n657 = local read "_Property"() -> (w560:string[])
                    n658 = Equal?(x=w560, y="ClassAttribute" ("Left Cell String(Main name)")) -> (x = y?=w564:bool[])
                    n659 = Empty String/Path?(string/path=w560) -> (empty?=w566:bool[])
                    n660 = Equal?(x=w560, y="ObjectAttribute" ("Left Cell String(Main name)")) -> (x = y?=w563:bool[])
                    n661 = Compound Arithmetic op=OR(w566, w563, w564) -> (w565:bool[])
                    n662 = Or Array Elements(Boolean array=w565) -> (logical OR=w559:bool)
                    n663 = Not(x=w559) -> (.not. x?=w567:bool)
                  }
                }
                n664 = Build Array(w527) -> (w532:string[])
                n665 = Empty Array?(array=w539) -> (empty?=w534:bool)
                n666 = Select(t=w532, s=w533, f=w531) -> (s? t:f=w530:string[])
                n667 = for {
                  tunnel: w528 -> [w552]
                  tunnel: [w546] -> w529
                  tunnel: w530 -> [w548] mode=indexing
                  stop <- w546 stop-if-true
                  n668 = To Lower Case(string=w552) -> (all lower case string=w550:string[])
                  n669 = Match Pattern(string=w548, regular expression="\\2E[Vv][Ii]") -> (before substring=w554:string)  [unwired: 1 in, 3 out]
                  n670 = Concatenate Strings(w554, ".vi" ("string")) -> (w547:string)
                  n671 = To Lower Case(string=w547) -> (all lower case string=w549:string)
                  n672 = Search 1D Array(1D array=w550, element=w549) -> (index of element=w551:i32)  [unwired: 1 in]
                  n673 = Greater Or Equal To 0?(x=w551) -> (x >= 0?=w546:bool)
                }
                n674 = Empty String/Path?(string/path=w540) -> (empty?=w542:bool)
                n675 = Empty String/Path?(string/path=w527) -> (empty?=w541:bool)
                n676 = Compound Arithmetic op=AND(invert w542, invert w541, invert w534, w537, invert w529) -> (w543:bool)
                n677 = property on="_DubMethodName" class="Str"("Visible"=w529) -> ()  [unwired: 2 in, 2 out]
                n678 = Select(t=u8 0, s=w543, f=u8 2 ("Disabled")) -> (s? t:f=w535:u8)
                n679 = property on="_CreateOpenClass" class="Bool"("Disabled"=w535) -> ()  [unwired: 2 in, 2 out]
                n680 = property on="_CreateMethod" class="Bool"("Disabled"=w535) -> ()  [unwired: 2 in, 2 out]
              }
            }
            n681 = Bundle By Name(cluster=w522, "Cancel"=w524, "Open"=w523, "OverrideMethod"=w511) -> (w525:T17)
          }
          frame "UpdateMethodSettings" {
            n682 = local read "_MethodLocation"() -> (w1701:i32)
            n683 = Unbundle By Name(w1702) -> ("FolderType"=w1703:T31)
            n684 = local read "_Visibility"() -> (w1729:T7)
            n685 = case shown="\"Community\"" w1729 {
              tunnel: [TRUE TRUE FALSE FALSE] -> w1724
              tunnel: [w1768 w1770 w1772 w1774] -> w1725
              frame "Public", Default {
                n686 = call <resource>:"GDSControl_Enable.vi"() -> ("Enable Property"=w1768:T19)  [unwired: 11 in]
              }
              frame "Protected" {
                n687 = call <resource>:"GDSControl_Enable.vi"() -> ("Enable Property"=w1770:T19)  [unwired: 11 in]
              }
              frame "Private" {
                n688 = call <resource>:"GDSControl_Disable.vi"() -> ("Enable Property"=w1772:T19)  [unwired: 11 in]
              }
              frame "Community" {
                n689 = call <resource>:"GDSControl_Disable.vi"() -> ("Enable Property"=w1774:T19)  [unwired: 11 in]
              }
            }
            n690 = Index Array(array=w1703, index=w1701) -> ()  [unwired: 1 out]
            n691 = Unbundle By Name(w1702) -> ("TemplateSettings.MustCallParent"=w1726:enum8{"False", "True", "Mixed"}, "TemplateSettings.MustOverride"=w1727:enum8{"False", "True", "Mixed"}, "TemplateSettings.DynamicDispatch"=w1728:enum8{"False", "True", "Mixed"})
            n692 = case shown="\"Mixed\"" w1726 {
              tunnel: [TRUE ("Value") FALSE w1754] -> w1710
              tunnel: w1725 -> [_ _ w1755]
              tunnel: [w1750 w1752 w1755] -> w1711
              frame "True" {
                n693 = call <resource>:"GDSControl_Disable.vi"() -> ("Enable Property"=w1750:T19)  [unwired: 11 in]
              }
              frame "False" {
                n694 = call <resource>:"GDSControl_Disable.vi"() -> ("Enable Property"=w1752:T19)  [unwired: 11 in]
              }
              frame "Mixed" {
                n695 = property on="_MustCallParent" class="Bool (strict)"() -> ("Value"=w1754:bool)  [unwired: 2 in, 2 out]
              }
            }
            n696 = case shown="\"Mixed\"" w1727 {
              tunnel: [TRUE ("Value") FALSE w1760] -> w1715
              tunnel: w1725 -> [_ _ w1761]
              tunnel: [w1756 w1758 w1761] -> w1714
              frame "True" {
                n697 = call <resource>:"GDSControl_Disable.vi"() -> ("Enable Property"=w1756:T19)  [unwired: 11 in]
              }
              frame "False" {
                n698 = call <resource>:"GDSControl_Disable.vi"() -> ("Enable Property"=w1758:T19)  [unwired: 11 in]
              }
              frame "Mixed" {
                n699 = property on="_MustOverride" class="Bool (strict)"() -> ("Value"=w1760:bool)  [unwired: 2 in, 2 out]
              }
            }
            n700 = case shown="\"Mixed\"" w1728 {
              tunnel: w1724 -> [w1763 _ w1766]
              tunnel: [w1763 FALSE w1766] -> w1712
              tunnel: w1725 -> [_ _ w1767]
              tunnel: [w1762 w1764 w1767] -> w1713
              frame "True" {
                n701 = call <resource>:"GDSControl_Disable.vi"() -> ("Enable Property"=w1762:T19)  [unwired: 11 in]
              }
              frame "False" {
                n702 = call <resource>:"GDSControl_Disable.vi"() -> ("Enable Property"=w1764:T19)  [unwired: 11 in]
              }
              frame "Mixed" {
              }
            }
            n703 = local read "_MethodType"() -> (w1716:T2)
            n704 = case shown="\"Override Method\"" w1716 {
              tunnel: w1711 -> [w1737 _]
              tunnel: [w1737 w1740] -> w1709
              tunnel: w1710 -> [w1736 _]
              tunnel: [w1736 TRUE ("Value")] -> w1708
              tunnel: w1714 -> [w1734 _]
              tunnel: [w1734 w1740] -> w1707
              tunnel: w1715 -> [w1735 w1739]
              tunnel: [w1735 w1739] -> w1706
              tunnel: w1713 -> [w1733 _]
              tunnel: [w1733 w1740] -> w1705
              tunnel: w1712 -> [w1732 w1738]
              tunnel: [w1732 w1738] -> w1704
              frame Default {
              }
              frame "Override Method" {
                n705 = call <resource>:"GDSControl_Disable.vi"() -> ("Enable Property"=w1740:T19)  [unwired: 11 in]
              }
            }
            n706 = local read ".vim"() -> (w1723:bool)
            n707 = case shown="True" w1723 {
              tunnel: w1709 -> [w1747 _]
              tunnel: [w1747 w1748] -> w1722
              tunnel: w1708 -> [w1746 _]
              tunnel: [w1746 w1749] -> w1721
              tunnel: w1707 -> [w1744 _]
              tunnel: [w1744 w1748] -> w1718
              tunnel: w1706 -> [w1745 _]
              tunnel: [w1745 w1749] -> w1717
              tunnel: w1705 -> [w1743 _]
              tunnel: [w1743 w1748] -> w1720
              tunnel: w1704 -> [w1742 _]
              tunnel: [w1742 w1749] -> w1719
              frame False {
              }
              frame True {
                w1749 = FALSE ("Value")
                n708 = call <resource>:"GDSControl_Disable.vi"() -> ("Enable Property"=w1748:T19)  [unwired: 11 in]
              }
            }
            n709 = property on="_MustOverride" class="Bool (strict)"("DisabledEnum"=w1718, "Value"=w1717) -> ()  [unwired: 2 in, 2 out]
            n710 = property on="_DynamicDispatch" class="Bool (strict)"("Disabled"=w1720, "Value"=w1719) -> ()  [unwired: 2 in, 2 out]
            n711 = property on="_MustCallParent" class="Bool (strict)"("Disabled"=w1722, "Value"=w1721) -> ()  [unwired: 2 in, 2 out]
          }
          frame "UpdateMethodTemplateImage" {
            n712 = Unbundle By Name(w1777) -> ("MethodItemNames"=w1799:string[])
            n713 = local read "_Method"() -> (w1782:i32[])
            n714 = Unbundle By Name(w1777) -> ("MethodVIs"=w1786:path[])
            n715 = Index Array(array=w1782) -> (element=w1785:i32)  [unwired: 1 in]
            n716 = property on="MethodTemplateImage" class="Pict"() -> ("Draw Area Size"=w1781:T18)  [unwired: 2 in, 2 out]
            n717 = Index Array(array=w1799, index=w1785) -> (element=w1798:string)
            n718 = Index Array(array=w1786, index=w1785) -> (element=w1784:path)
            n719 = call <resource>:"GetMethodImage.vi"("MethodVI"=w1784, "MethodName"=w1798) -> ("MethodImage"=w1778:T15)  [unwired: 8 in, 1 out]
            n720 = Unbundle By Name(w1781) -> ("Width"=w1797:u32, "Height"=w1796:u32)
            n721 = To Word Integer(number=w1797) -> (16bit integer=w1790:i16)
            n722 = Unbundle By Name(w1778) -> ("Rectangle.right"=w1789:i16, "Rectangle.bottom"=w1787:i16)
            n723 = To Word Integer(number=w1796) -> (16bit integer=w1788:i16)
            n724 = Unbundle By Name(w1778) -> ("Rectangle"=w1795:T45)
            n725 = Subtract(x=w1790, y=w1789) -> (x-y=w1792:i16)
            n726 = Subtract(x=w1788, y=w1787) -> (x-y=w1793:i16)
            n727 = Max & Min(x=w1792, y=w1793) -> (min(x,y)=w1791:i16)  [unwired: 1 out]
            n728 = case shown="..-1" w1791 {
              tunnel: w1795 -> [_ w1817]
              tunnel: w1778 -> [w1809 w1815]
              tunnel: [w1809 w1813] -> w1794
              tunnel: w1793 -> [_ w1812]
              tunnel: w1792 -> [_ w1811]
              tunnel: [w1802 1.0] -> w1780
              tunnel: w1790 -> [w1808 _]
              tunnel: w1789 -> [w1807 _]
              tunnel: w1788 -> [w1806 _]
              tunnel: w1787 -> [w1805 _]
              tunnel: [T30 {"Horizontal"=0, "Vertical"=0} ("Origin") _] -> w1779
              frame ..-1 {
                n729 = Divide(x=w1808, y=w1807) -> (x/y=w1804:dbl)
                n730 = Divide(x=w1806, y=w1805) -> (x/y=w1803:dbl)
                n731 = Max & Min(x=w1804, y=w1803) -> (min(x,y)=w1802:dbl)  [unwired: 1 out]
              }
              frame Default {
                n732 = expression code="x/2"(w1811) -> (w1819:i16)
                n733 = expression code="y/2"(w1812) -> (w1818:i16)
                n734 = Bundle(w1819, w1818, w1819, w1818) -> (w1816:cluster{i16, i16, i16, i16})  [unwired: 1 in]
                n735 = Add(x=w1817, y=w1816) -> (x+y=w1814:cluster{i16, i16, i16, i16})
                n736 = Bundle By Name(cluster=w1815, "Rectangle"=w1814) -> (w1813:T15)
              }
            }
            n737 = call <vilib>:"Draw Flattened Pixmap.vi"("image data"=w1794) -> ("new picture"=w1776:picture)  [unwired: 8 in]
            n738 = property on="MethodTemplateImage" class="Pict"("ZoomFactor"=w1780, "Origin"=w1779, "Value"=w1776) -> ()  [unwired: 2 in, 2 out]
          }
          frame "GetImageData" {
            # "Create White mask Color, When Mouse Down"
            n739 = Unbundle By Name(w1828) -> ("Icons"=w1832:T15[], "IconSelected"=w1831:i32)
            n740 = Index Array(array=w1832, index=w1831) -> (element=w1820:T15)
            n741 = call <resource>:"GDSIconEditor_ShrinkImage.vi"("image data"=w1820) -> ("image subset"=w1821:T15)  [unwired: 9 in]
            n742 = call <resource>:"GDSIconEditor_ImageDataTo8Bit.vi"("image data"=w1821) -> ("NoMaskFound"=w1822:bool, "8-bit pixmap"=w1823:u8[][], "mask"=w1830:u8[])  [unwired: 7 in, 1 out]
            n743 = property on="FloodFillMask" class="Bool (strict)"("Visible"=w1822) -> ()  [unwired: 2 in, 2 out]
            n744 = case shown="True" w1822 {
              tunnel: w1823 -> [_ w1836]
              tunnel: w1830 -> [w1833 _]
              tunnel: [w1833 w1835] -> w1827
              frame False {
              }
              frame True {
                n745 = local read "FloodFillMask"() -> (w1834:bool)
                n746 = call <resource>:"GDSIconEditor_CreateImageMask.vi"("Flood Fill"=w1834, "8-bit pixmap"=w1836) -> ("Array"=w1835:u8[])
              }
            }
            n747 = call <vilib>:"Draw Flattened Pixmap.vi"("image data"=w1821) -> ("new picture"=→"DragIcon":picture)  [unwired: 8 in]
            n748 = Bundle By Name(cluster=w1828, "BgIcon"=w1823, "BgIconMask"=w1827) -> (w1826:T17)
          }
          frame "UpdateIconFolderList" {
            # "C:\\Users\\Mikael\\Documents\\LabVIEW Data\\Glyphs"
            n749 = VI Library() -> (path=w1870:path)
            n750 = Strip Path(path=w1870) -> (stripped path=w1858:path)  [unwired: 1 out]
            n751 = call <resource>:"GOOP_GetProviderIniFilePath.vi"() -> ("ProviderMainFolder"=w1881:path)  [unwired: 10 in, 1 out]
            n752 = call <resource>:"GOOP_GetGDSConfigFolder.vi"() -> ("GDSFolderPath"=w1843:path)
            n753 = call <vilib>:"Set Busy.vi"("error in (no error)"=w1842) -> ("error out"=w1841:errorcluster)  [unwired: 9 in, 1 out]
            n754 = Build Path(base path=w1843, name or relative path="IconFolder.txt") -> (appended path=w1851:path)
            n755 = Build Path(base path=w1858, name or relative path="resource") -> (appended path=w1869:path)
            n756 = call <vilib>:"Dflt Data Dir.vi"() -> ("App:Default Data Directory"=w1862:path)
            n757 = Read from Text File(file (use dialog)=w1851) -> (text=w1845:string)  [unwired: 3 in, 3 out]
            n758 = Build Path(base path=w1869, name or relative path="Framework") -> (appended path=w1868:path)
            n759 = call <vilib>:"Trim Whitespace.vi"("string"=w1845) -> ("trimmed string"=w1855:string)  [unwired: 1 in]
            n760 = Build Path(base path=w1862, name or relative path="Glyphs") -> (appended path=w1861:path)
            n761 = Build Path(base path=w1868, name or relative path="Providers") -> (appended path=w1859:path)
            n762 = Spreadsheet String To Array(delimiter (Tab)="\n", format string="%s", spreadsheet string=w1855, array type (2D Dbl)=string[] []) -> (array=w1875:string[])
            n763 = Build Path(base path=w1859, name or relative path="Icons") -> (appended path=w1873:path)
            n764 = Build Path(base path=w1881, name or relative path="Glyphs") -> (appended path=w1879:path)
            n765 = Build Path(base path=w1881, name or relative path="Icons") -> (appended path=w1882:path)
            n766 = Path To String(path=w1873) -> (string=w1871:string)
            n767 = Path To String(path=w1879) -> (string=w1872:string)
            n768 = Path To String(path=w1882) -> (string=w1883:string)
            n769 = Path To String(path=w1861) -> (string=w1837:string)
            n770 = Build Array(w1871, w1872, w1883, w1837) -> (w1874:string[])
            n771 = Build Array (concatenate)(w1874, w1875) -> (w1876:string[])
            n772 = for {
              tunnel: w1876 -> [w1885] mode=indexing
              tunnel: [w1888] -> w1878 mode=indexing
              tunnel: [w1884] -> w1877 mode=indexing
              n773 = String To Path(string=w1885) -> (path=w1888:path)
              n774 = String Length(string=w1885) -> (length=w1886:i32)
              n775 = Subtract(x=w1886, y=45) -> (x-y=w1887:i32)
              n776 = case shown="1.." w1887 {
                selector: w1887 -> [_ w1897]
                tunnel: w1886 -> [_ _]
                tunnel: w1885 -> [w1890 w1895]
                tunnel: [w1890 w1892] -> w1884
                frame 0, Default {
                }
                frame 1.. {
                  n777 = Add(x=w1897, y=3) -> (x+y=w1894:i32)
                  n778 = String Subset(string=w1895, offset (0)=w1894) -> (substring=w1893:string)  [unwired: 1 in]
                  n779 = Concatenate Strings("..." ("string"), w1893) -> (w1892:string)
                }
              }
            }
            n780 = for {
              tunnel: w1878 -> [w1902] mode=indexing
              shift-right: [w1907] -> w1854
              shift-left: path[] [] -> [w1903]
              shift-right: [w1906] -> w1857
              shift-left: string[] [] -> [w1905]
              tunnel: w1877 -> [w1904] mode=indexing
              n781 = Empty String/Path?(string/path=w1902) -> (empty?=w1900:bool)
              n782 = Search 1D Array(1D array=w1903, element=w1902) -> (index of element=w1901:i32)  [unwired: 1 in]
              n783 = Greater Or Equal To 0?(x=w1901) -> (x >= 0?=w1899:bool)
              n784 = Or(x=w1900, y=w1899) -> (x .or. y?=w1898:bool)
              n785 = case shown="False" w1898 {
                tunnel: w1902 -> [w1911 _]
                tunnel: w1903 -> [w1914 w1924]
                tunnel: [w1913 w1924] -> w1907
                tunnel: w1905 -> [w1909 w1923]
                tunnel: [w1910 w1923] -> w1906
                tunnel: w1904 -> [w1908 _]
                frame False {
                  n786 = call <vilib>:"Check if File or Folder Exists.vi"("path"=w1911) -> ("file or folder exists?"=w1912:bool)  [unwired: 8 in, 2 out]
                  n787 = case shown="True" w1912 {
                    tunnel: w1914 -> [w1916 w1922]
                    tunnel: [w1916 w1921] -> w1913
                    tunnel: w1911 -> [_ w1920]
                    tunnel: w1909 -> [w1915 w1918]
                    tunnel: [w1915 w1919] -> w1910
                    tunnel: w1908 -> [_ w1917]
                    frame False {
                    }
                    frame True {
                      n788 = Build Array (concatenate)(w1922, w1920) -> (w1921:path[])
                      n789 = Build Array (concatenate)(w1918, w1917) -> (w1919:string[])
                    }
                  }
                }
                frame True {
                }
              }
            }
            n790 = Build Array (concatenate)("<All icons>" ("y"), w1857) -> (w1850:string[])
            n791 = property on="_Folders" class="Ring (strict)"("Strings []"=w1850, "Value"=1) -> ()  [unwired: 2 in, 2 out]
            n792 = Bundle By Name(cluster=w1839, "Folders"=w1854) -> (w1838:T17)
          }
          frame "ReadIcons" {
            (unwired) "" ("Name")
            n793 = local read "_Folders"() -> (w1925:u16)
            n794 = Unbundle By Name(w1928) -> ("Folders"=w1932:path[])
            n795 = case shown="Default" w1925 {
              selector: w1925 -> [_ w1938]
              tunnel: w1932 -> [w1937 w1942]
              tunnel: [w1937 w1939] -> w1933
              frame 0 {
              }
              frame Default {
                n796 = Decrement(x=w1938) -> (x-1=w1941:u16)
                n797 = Index Array(array=w1942, index=w1941) -> (element=w1940:path)
                n798 = Build Array(w1940) -> (w1939:path[])
              }
            }
            n799 = call <vilib>:"Set Busy.vi"("error in (no error)"=w1931) -> ("error out"=w1934:errorcluster)  [unwired: 9 in, 1 out]
            n800 = for {
              tunnel: w1933 -> [w1947] mode=indexing
              shift-right: [w1943] -> w1936
              shift-left: cluster{i32, "path out":path}[] [] -> [w1944]
              shift-right: [w1948] -> w1930
              shift-left: w1934 -> [w1945]
              n801 = call <vilib>:"Check if File or Folder Exists.vi"("path"=w1947) -> ("file or folder exists?"=w1946:bool)  [unwired: 8 in, 2 out]
              n802 = case shown="True" w1946 {
                tunnel: [w1950 w1956] -> w1948
                tunnel: w1945 -> [w1950 w1955]
                tunnel: w1947 -> [_ w1954]
                tunnel: w1944 -> [w1949 w1951]
                tunnel: [w1949 w1953] -> w1943
                frame False {
                }
                frame True {
                  n803 = call <vilib>:"Recursive File List.vi"("pattern"="*.png", "error in (no error)"=w1955, "Folder Path"=w1954) -> ("error out"=w1958:errorcluster, "All Files in Dir"=w1959:path[])  [unwired: 4 in, 3 out]
                  n804 = for {
                    tunnel: w1959 -> [w1967] mode=indexing
                    tunnel: [w1965] -> w1952 mode=indexing
                    shift-right: [w1964] -> w1956
                    shift-left: w1958 -> [w1968]
                    n805 = File/Directory Info(path=w1967, error in=w1968) -> (path out=w1966:path, size=w1963:i64, error out=w1964:errorcluster)  [unwired: 4 out]
                    n806 = Divide(x=w1963, y=i64 100) -> (x/y=w1961:dbl)
                    n807 = To Long Integer(number=w1961) -> (32bit integer=w1960:i32)
                    n808 = Bundle(w1960, "path out"=w1966) -> (w1965:cluster{i32, "path out":path})  [unwired: 1 in]
                  }
                  n809 = Build Array (concatenate)(w1951, w1952) -> (w1953:cluster{i32, "path out":path}[])
                }
              }
            }
            n810 = Sort 1D Array(array=w1936) -> (sorted array=w1929:cluster{i32, "path out":path}[])
            n811 = Bundle By Name(cluster=w1928, "IconPaths"=w1929) -> (w1927:T17)
          }
          frame "PlaceIcon" {
            n812 = Unbundle By Name(w1972) -> ("Icons"=w1974:T15[], "IconSelected"=w1975:i32)
            n813 = Index Array(array=w1974, index=w1975) -> (element=w1976:T15)
            n814 = call <resource>:"GDSIconEditor_ImageDataTo8Bit.vi"("image data"=w1976) -> ("8-bit pixmap"=w1969:u8[][])  [unwired: 7 in, 3 out]
            n815 = Bundle By Name(cluster=w1972, "BgIcon"=w1969, "BgIconOffset"=cluster{"X":i32, "Y":i32} {"X"=0, "Y"=0}) -> (w1973:T17)
          }
          frame "DrawIcons", "DrawIcons:NoBusy" {
            w1988 = 0  # IconsPerRow
            w1984 = 10  # Border
            w1986 = 15  # Gap
            # "Y"
            # "X"
            n816 = case shown="\"DrawIcons:NoBusy\"" w1978 {
              tunnel: [w2005 w2006] -> w1999
              tunnel: w1982 -> [w2004 w2006]
              frame Default {
                n817 = call <vilib>:"Set Busy.vi"("error in (no error)"=w2004) -> ("error out"=w2005:errorcluster)  [unwired: 9 in, 1 out]
              }
              frame "DrawIcons:NoBusy" {
              }
            }
            n818 = Unbundle By Name(w1981) -> ("IconPaths"=w1998:cluster{i32, "path out":path}[])
            n819 = local read "_IconSearchText"() -> (w2000:string)
            n820 = property on="Icons" class="Pict"() -> ("Draw Area Size"=w1991:T18)  [unwired: 2 in, 2 out]
            n821 = Unbundle By Name(w1991) -> ("Width"=w1985:u32)
            n822 = property on="Icons" class="Pict"("Origin"=T30 {"Horizontal"=0, "Vertical"=0}) -> ()  [unwired: 2 in, 2 out]
            n823 = call <vilib>:"Trim Whitespace.vi"("string"=w2000) -> ("trimmed string"=w2001:string)  [unwired: 1 in]
            n824 = for {
              shift-right: [w2035] -> w1979
              shift-left: w1999 -> [w2018]
              shift-right: [w2022] -> _
              shift-left: w1984 -> [w2030]
              shift-right: [w2033] -> w2003
              shift-left: picture data[5B] ("new picture") -> [w2034]
              shift-right: [w2031] -> w1992
              shift-left: T15[] [] -> [w2032]
              shift-right: [w2023] -> _
              shift-left: w1988 -> [w2024]
              shift-right: [w2021] -> _
              shift-left: w1984 -> [w2025]
              shift-right: [w2026] -> _
              shift-left: TRUE -> [w2029]
              tunnel: w1986 -> [w2028]
              tunnel: w1985 -> [w2027]
              tunnel: w1984 -> [w2020]
              tunnel: w1998 -> [w2019] mode=indexing
              shift-right: [w2017] -> w1994
              shift-left: cluster{i32, i32, i32, i32}[] [] -> [w2016]
              shift-right: [w2014] -> w1997
              shift-left: string[] [] -> [w2015]
              tunnel: w2001 -> [w2013]
              n825 = Unbundle(w2019) -> (w2011:i32, "path out"=w2012:path)
              n826 = case shown="\"\"" w2013 {
                selector: w2013 -> [w2041 _]
                tunnel: w2012 -> [w2042 _]
                tunnel: [w2036 TRUE] -> w2008
                frame Default {
                  n827 = To Lower Case(string=w2041) -> (all lower case string=w2038:string)
                  n828 = call <vilib>:"Get File Extension.vi"("file"=w2042) -> ("filename without extension"=w2040:string)  [unwired: 6 in, 4 out]
                  n829 = To Lower Case(string=w2040) -> (all lower case string=w2039:string)
                  n830 = Match Pattern(string=w2039, regular expression=w2038) -> (offset past match=w2037:i32)  [unwired: 1 in, 3 out]
                  n831 = Greater Or Equal To 0?(x=w2037) -> (x >= 0?=w2036:bool)
                }
                frame "" {
                }
              }
              n832 = Less Or Equal?(x=w2011, y=50) -> (x <= y?=w2009:bool)
              n833 = And(x=w2008, y=w2009) -> (x .and. y?=w2007:bool)
              n834 = case shown="True" w2007 {
                tunnel: w2012 -> [_ w2056]
                tunnel: w2018 -> [w2052 w2085]
                tunnel: [w2052 w2084] -> w2035
                tunnel: w2034 -> [w2051 w2083]
                tunnel: [w2051 w2062] -> w2033
                tunnel: w2032 -> [w2050 w2068]
                tunnel: [w2050 w2082] -> w2031
                tunnel: w2030 -> [w2048 w2065]
                tunnel: w2029 -> [w2046 w2081]
                tunnel: w2028 -> [_ w2067]
                tunnel: w2027 -> [_ w2078]
                tunnel: [w2046 w2077] -> w2026
                tunnel: w2025 -> [w2047 w2072]
                tunnel: w2024 -> [w2049 w2071]
                tunnel: [w2049 w2070] -> w2023
                tunnel: [w2048 w2060] -> w2022
                tunnel: [w2047 w2064] -> w2021
                tunnel: w2020 -> [_ w2066]
                tunnel: w2016 -> [w2045 w2059]
                tunnel: [w2045 w2058] -> w2017
                tunnel: w2015 -> [w2044 w2054]
                tunnel: [w2044 w2055] -> w2014
                frame False {
                }
                frame True {
                  # "Place This Icon on a new row"
                  n835 = call <vilib>:"Read PNG File.vi"("error in (no error)"=w2085, "path to PNG file"=w2056) -> ("error out"=w2084:errorcluster, "image data"=w2076:T15)  [unwired: 7 in, 1 out]
                  n836 = Unbundle By Name(w2076) -> ("Rectangle"=w2075:T45)
                  n837 = Unbundle By Name(w2076) -> ("Rectangle.right"=w2063:i16)
                  n838 = Select(t=0, s=w2081, f=w2067) -> (s? t:f=w2080:i32)
                  n839 = Add(x=w2080, y=w2065) -> (x+y=w2073:i32)
                  n840 = Strip Path(path=w2056) -> (name=w2053:string)  [unwired: 1 out]
                  n841 = Add(x=w2073, y=w2063) -> (x+y=w2069:i32)
                  n842 = Greater?(x=w2069, y=w2078) -> (0:w2077:bool)
                  n843 = Build Array (concatenate)(w2068, w2076) -> (w2082:T15[])
                  n844 = case shown="True" w2077 {
                    tunnel: [w2090 w2096] -> w2074
                    tunnel: w2073 -> [w2087 _]
                    tunnel: w2072 -> [w2086 w2091]
                    tunnel: w2071 -> [w2089 w2099]
                    tunnel: [w2088 1] -> w2070
                    tunnel: w2068 -> [_ w2100]
                    tunnel: w2067 -> [_ w2094]
                    tunnel: w2066 -> [_ w2093]
                    tunnel: w2065 -> [_ _]
                    tunnel: [w2086 w2092] -> w2064
                    tunnel: w2063 -> [_ _]
                    frame False {
                      n845 = Bundle(w2087, "Border"=w2086, w2087, "Border"=w2086) -> (w2090:cluster{i32, "Border":i32, i32, "Border":i32})  [unwired: 1 in]
                      n846 = Increment(x=w2089) -> (x+1=w2088:i32)
                    }
                    frame True {
                      n847 = Delete From Array(array=w2100, length=w2099) -> (deleted portion=w2098:T15[])  [unwired: 1 in, 1 out]
                      n848 = for {
                        tunnel: w2098 -> [w2103] mode=indexing
                        tunnel: [w2102] -> w2097 mode=indexing
                        n849 = Unbundle By Name(w2103) -> ("Rectangle.bottom"=w2102:i16)
                      }
                      n850 = Array Max & Min(array=w2097) -> (max value=w2095:i16)  [unwired: 3 out]
                      n851 = Compound Arithmetic op=ADD(w2091, w2094, w2095) -> (w2092:i32)
                      n852 = Bundle("Border"=w2093, w2092, "Border"=w2093, w2092) -> (w2096:cluster{"Border":i32, i32, "Border":i32, i32})  [unwired: 1 in]
                    }
                  }
                  n853 = Add(x=w2074, y=w2075) -> (x+y=w2057:cluster{i32, i32, i32, i32})
                  n854 = Bundle By Name(cluster=w2076, "Rectangle"=w2057) -> (w2061:T15)
                  n855 = Build Array (concatenate)(w2059, w2057) -> (w2058:cluster{i32, i32, i32, i32}[])
                  n856 = Build Array (concatenate)(w2054, w2053) -> (w2055:string[])
                  n857 = Unbundle By Name(w2061) -> ("Rectangle.right"=w2060:i16)
                  n858 = call <vilib>:"Draw Flattened Pixmap.vi"("image data"=w2061, "picture"=w2083) -> ("new picture"=w2062:picture)  [unwired: 7 in]
                }
              }
            }
            "Icons" <- w2003
            n859 = property on="DragIcon" class="Pict"("Visible"=FALSE) -> ()  [unwired: 2 in, 2 out]
            n860 = Bundle By Name(cluster=w1981, "Icons"=w1992, "IconPos"=w1994, "IconNames"=w1997) -> (w1980:T17)
            n861 = call <vilib>:"Unset Busy.vi"("error in (no error)"=w1979) -> ()  [unwired: 10 in, 1 out]
          }
          frame "CreateMethodIcons" {
            w2132 = T40 {"BgIcon"=[], "BgIconOffset"={"X"=0, "Y"=0}, "BgIconMask"=[], "ColorsOkayforiconToBeOnTopOf"=[]}  # BgIcon
            n862 = Unbundle By Name(w2109) -> ("Frame thickness"=w2130:i32, "ConnectorPaneHeight"=w2122:i32[], "BodyIconHeight"=w2123:i32)
            n863 = Unbundle By Name(w2109) -> ("Frame"=w2114:u32, "Frame thickness"=w2115:i32, "HeaderIcon"=w2126:u8[][])
            n864 = local read "_IconSize"() -> (w2127:u16)
            n865 = local read "_BodyBk"() -> (w2120:T1)
            n866 = Unbundle By Name(w2120) -> ("Color"=w2139:u32)
            n867 = Unbundle By Name(w2109) -> ("BgIcon"=w2133:u8[][], "BgIconOffset"=w2134:cluster{"X":i32, "Y":i32}, "BgIconMask"=w2136:u8[], "HeaderBkColor"=w2137:u32)
            n868 = Unbundle By Name(w2109) -> ("MethodNames"=w2142:string[])
            n869 = Unbundle By Name(w2109) -> ("BodyIconHeight"=w2149:i32, "BodyIconWidth"=w2148:i32)
            n870 = case shown="1" w2127 {
              tunnel: w2126 -> [w2163 _]
              tunnel: [w2163 _] -> w2116
              frame Default {
              }
              frame 1 {
              }
            }
            n871 = call <resource>:"GDSLvIcon_Convert24bitTo8bitColor.vi"("Color 24bit In"=w2137) -> ("Color out(256)"=w2138:u8)  [unwired: 15 in, 3 out]
            n872 = call <resource>:"GDSLvIcon_Convert24bitTo8bitColor.vi"("Color 24bit In"=w2139) -> ("Color out(256)"=w2140:u8)  [unwired: 15 in, 3 out]
            n873 = Not Equal?(x=u16 0, y=w2127) -> (x != y?=w2128:bool)
            n874 = Array Size(array=w2116) -> (size(s)=w2124:i32[])
            n875 = Build Array(w2138, w2140) -> (w2135:u8[])
            n876 = Index Array(array=w2124) -> (element=w2125:i32)  [unwired: 1 in]
            n877 = Select(t=0, s=w2128, f=0) -> (s? t:f=w2112:i32)
            n878 = Multiply(x=w2130, y=u32 2) -> (x*y=w2131:u32)
            n879 = case shown="Default" w2127 {
              selector: w2127 -> [_ w2151 _]
              tunnel: w2123 -> [_ _ _]
              tunnel: w2122 -> [_ w2158 w2161]
              tunnel: [32 ("ImageRows(32)") w2155 w2162] -> w2113
              tunnel: w2125 -> [_ w2154 _]
              tunnel: w2131 -> [_ w2153 w2159]
              frame 0 {
              }
              frame Default {
                n880 = Decrement(x=w2151) -> ()  [unwired: 1 out]
                n881 = Array Subset(array=w2158, length=w2151) -> (w2157:i32[])  [unwired: 1 in]
                n882 = Add Array Elements(numeric array=w2157) -> (sum=w2156:i32)
                n883 = Increment(x=w2153) -> (x+1=w2152:u32)
                n884 = Compound Arithmetic op=ADD(w2152, w2154, w2156) -> (w2155:u32)
              }
              frame 1 {
                n885 = Index Array(array=w2161) -> (element=w2160:i32)  [unwired: 1 in]
                n886 = Compound Arithmetic op=ADD(w2159, w2160) -> (w2162:u32)
              }
            }
            n887 = Bundle By Name(cluster=w2132, "BgIcon"=w2133, "BgIconOffset"=w2134, "BgIconMask"=w2136, "ColorsOkayforiconToBeOnTopOf"=w2135) -> (w2117:T40)
            n888 = local read "_MethodIconName"() -> (w2111:string)
            n889 = local read "_Property"() -> (w2106:string[])
            n890 = Array Size(array=w2106) -> (size(s)=w2105:i32)
            n891 = Greater Or Equal?(x=w2105, y=2) -> (x >= y?=w2104:bool)
            n892 = Unbundle By Name(w2109) -> ("Offset"=w2110:cluster{"X":i32, "Y":i32})
            n893 = for {
              tunnel: w2149 -> [w2192]
              tunnel: w2148 -> [w2191]
              shift-right: [w2181] -> w2145
              shift-left: w2146 -> [w2186]
              shift-right: [w2184] -> w2141
              shift-left: u8[][] [] -> [w2185]
              tunnel: w2142 -> [w2167] mode=indexing
              tunnel: w2117 -> [w2180]
              tunnel: w2116 -> [w2179]
              tunnel: w2115 -> [w2178]
              tunnel: w2114 -> [w2177]
              tunnel: w2113 -> [w2176]
              tunnel: w2112 -> [w2175]
              tunnel: w2111 -> [w2171]
              tunnel: w2110 -> [w2173]
              tunnel: "^Read|^Get|^Write|^Set|" ("regular expression") -> [w2170]
              tunnel: w2104 -> [w2164]
              n894 = xnode "Match Regular Expression"("input string"=w2167, "regular expression"=w2170) -> ("whole match"=w2172:string)  [unwired: 4 in, 4 out]
              n895 = xnode "Match Regular Expression"("input string"=w2171, "regular expression"=w2170) -> ("before match"=w2169:string, "after match"=w2168:string)  [unwired: 4 in, 3 out]
              n896 = Concatenate Strings(w2172, w2169, w2168) -> (w2166:string)
              n897 = Select(t=w2167, s=w2164, f=w2166) -> (s? t:f=w2165:string)
              n898 = local read "_BodyBk"() -> (w2190:T1)
              n899 = local read "_BodyText"() -> (w2188:T1)
              n900 = local read "_FontCompression"() -> (w2195:enum16{"Auto", "On", "Off"})
              n901 = local read "_CapitalOnly"() -> (w2194:bool)
              n902 = Bundle By Name(cluster=T26 {"Text"="", "Allow Only Capital Chars"=FALSE, "Compression"=enum."Auto", "Alignment"=enum."Center"} ("Text"), "Text"=w2165, "Allow Only Capital Chars"=w2194, "Compression"=w2195) -> (w2193:T26)
              n903 = Unbundle(w2188) -> ("Color"=w2187:u32)  [unwired: 1 out]
              n904 = Unbundle(w2190) -> ("Color"=w2189:u32)  [unwired: 1 out]
              n905 = call <resource>:"GDSLvIcon_GenerateIconText.vi"("Text"=w2193, "TextPixelHeight(5-30)"=w2192, "Foreground color"=w2187, "Background color"=w2189, "error in (no error)"=w2186, "Offset"=w2173, "Text Pixel width(32-FrameThicknes*2))"=w2191) -> ("TextOut"=w2183:u8[][], "error out"=w2182:errorcluster)  [unwired: 8 in, 3 out]
              n906 = call <resource>:"GDSLvIcon_CreateIconPicture.vi"("FrameColor"=w2177, "FrameThickness(1)"=w2178, "HeaderIconIn"=w2179, "BodyIconIn"=w2183, "error in (no error)"=w2182, "ImageRows(32)"=w2176, "RowStart(0)"=w2175, "BgIcon"=w2180) -> ("BodyIconOut"=w2174:u8[][], "error out"=w2181:errorcluster)  [unwired: 6 in, 4 out]
              n907 = Build Array (concatenate)(w2185, w2174) -> (w2184:u8[][])
            }
            n908 = Bundle By Name(cluster=w2109, "BodyIconOut"=w2141) -> (w2147:T17)
          }
          frame "UpdateOverRideMethods" {
            w2419 = TRUE ("Visible")
            n909 = Unbundle By Name(w2422) -> ("OverRideLookUpDone"=w2425:bool)
            n910 = local write "_OverrideMethods"(-1 ("Override Methods")) -> ()
            n911 = property on="_Property" class="Tree (strict)"("Visible"=FALSE) -> ()  [unwired: 2 in, 2 out]
            n912 = property on="_OverrideMethods" class="LstBox (strict)"("Visible"=w2419) -> ()  [unwired: 2 in, 2 out]
            n913 = property on="Filter" class="Str"("Visible"=w2419) -> ()  [unwired: 2 in, 2 out]
            n914 = case shown="False" w2425 {
              tunnel: w2427 -> [w2440 w2452]
              tunnel: w2426 -> [w2449 _]
              tunnel: [w2437 w2452] -> w2420
              tunnel: w2422 -> [w2443 w2451]
              tunnel: [w2442 w2451] -> w2421
              tunnel: [w2436 _] -> _
              frame False {
                w2434 = "" ("Method Name")
                n915 = call <vilib>:"Set Busy.vi"("error in (no error)"=w2440) -> ("error out"=w2439:errorcluster)  [unwired: 9 in, 1 out]
                n916 = local write "_MethodName"(w2434) -> ()
                n917 = local write "_MethodIconName"(w2434) -> ()
                n918 = local write "Filter"("" ("Filter")) -> ()
                n919 = property on="_Loading" class="Str"(error in=w2439, "Visible"=TRUE) -> (error out=w2447:errorcluster)  [unwired: 1 in, 1 out]
                n920 = call <resource>:"GOOP_GetOverrideMethods.vi"("LvClassItem"=w2449, "error in (no error)"=w2447) -> ("IsAPropertyDefinitionVI"=w2433:bool[], "DynamicMethods(Names)"=w2430:string[], "DynamicMehods(Paths)"=w2441:path[], "Scope"=w2438:T31, "ConnectorPaneHeight"=w2435:i32[], "error out"=w2445:errorcluster)  [unwired: 12 in]
                n921 = property on="_OverrideMethods" class="LstBox (strict)"("Item Names"=w2430, "Top Row"=0) -> ()  [unwired: 2 in, 2 out]
                n922 = for {
                  tunnel: w2430 -> [_] mode=indexing
                  tunnel: [w2450] -> w2429 mode=indexing
                  i -> [w2450]
                }
                n923 = Bundle By Name(cluster=w2443, "OverrideMethodsIdx"=w2429, "OverrideMethodsNames"=w2430, "OverRideLookUpDone"=TRUE, "AllOverrideMethods"=w2441, "OverrideScope"=w2438, "ConnectorPaneHeight"=w2435, "IsAPropertyDefinitionVI"=w2433) -> (w2442:T17)
                n924 = property on="_Loading" class="Str"(error in=w2445, "Visible"=FALSE) -> (error out=w2437:errorcluster)  [unwired: 1 in, 1 out]
                n925 = call <vilib>:"Unset Busy.vi"("error in (no error)"=w2437) -> ("error out"=w2436:errorcluster)  [unwired: 10 in]
              }
              frame True {
              }
            }
          }
          frame "UpdateProperties" {
            (unwired) "" ("Property")
            w2453 = FALSE ("Visible")
            n926 = Unbundle By Name(w2460) -> ("PropertyLookUpDone"=w2461:bool)
            n927 = case shown="False" w2461 {
              tunnel: w2463 -> [w2471 w2477]
              tunnel: w2462 -> [w2476 _]
              tunnel: [w2466 w2477] -> w2454
              tunnel: w2456 -> [w2467 _]
              tunnel: [w2465 _] -> _
              frame False {
                w2472 = "" ("Method Name")
                n928 = control-ref of="_Property"() -> (w2469:refnum<vi>)
                n929 = call <vilib>:"Set Busy.vi"("error in (no error)"=w2471) -> ("error out"=w2470:errorcluster)  [unwired: 9 in, 1 out]
                n930 = property on="_Loading" class="Str"(error in=w2470, "Visible"=TRUE) -> (error out=w2474:errorcluster)  [unwired: 1 in, 1 out]
                n931 = call-dynamic "GetClassProperties.vi"("reference in"=w2467, "LvClassItem"=w2476, "TreeControl"=w2469, "error in (no error)"=w2474) -> ("error out"=w2468:errorcluster)  [unwired: 14 in, 1 out]
                n932 = local write "_MethodName"(w2472) -> ()
                n933 = local write "_MethodIconName"(w2472) -> ()
                n934 = property on="_Loading" class="Str"(error in=w2468, "Visible"=FALSE) -> (error out=w2466:errorcluster)  [unwired: 1 in, 1 out]
                n935 = call <vilib>:"Unset Busy.vi"("error in (no error)"=w2466) -> ("error out"=w2465:errorcluster)  [unwired: 10 in]
              }
              frame True {
              }
            }
            n936 = property on="_Property" class="Tree (strict)"("Visible"=TRUE) -> ()  [unwired: 2 in, 2 out]
            n937 = property on="_OverrideMethods" class="LstBox (strict)"("Visible"=w2453) -> ()  [unwired: 2 in, 2 out]
            n938 = property on="Filter" class="Str"("Visible"=w2453) -> ()  [unwired: 2 in, 2 out]
            n939 = local write "_Property"(string[] [] ("_Property")) -> ()
            n940 = Bundle By Name(cluster=w2460, "PropertyLookUpDone"=TRUE ("OverRideLookUpDone")) -> (w2459:T17)
          }
          frame "Generate icon", "UpdateIcon" {
            (unwired) T20."1 c-term high"  # _IconSize
            (unwired) 3  # TerminalHeight
            n941 = local read "_IconSize"() -> (w2510:u16)
            n942 = local read "_MethodIconName"() -> (w2481:string)
            n943 = local read "_MethodType"() -> (w2482:T2)
            n944 = Unbundle By Name(w2487) -> ("Offset"=w2496:cluster{"X":i32, "Y":i32}, "Frame"=w2512:u32, "Frame thickness"=w2526:i32, "HeaderIcon"=w2515:u8[][])
            n945 = Unbundle By Name(w2487) -> ("ConnectorPaneHeight"=w2511:i32[], "BodyIconHeight"=w2509:i32, "BodyIconWidth"=w2521:i32)
            n946 = Unbundle By Name(w2487) -> ("CurrentIcon"=w2486:T40)
            n947 = case shown="\"Property Node\"" w2482 {
              tunnel: w2481 -> [w2533 w2536]
              tunnel: [w2533 w2534] -> w2480
              frame Default {
              }
              frame "Property Node" {
                n948 = Match Pattern(string=w2536, regular expression="/") -> (before substring=w2534:string)  [unwired: 1 in, 3 out]
              }
            }
            n949 = case shown="Default" w2510 {
              tunnel: w2515 -> [w2578 _]
              tunnel: [w2578 _] -> w2506
              frame Default {
              }
              frame 1 {
              }
            }
            n950 = Array Size(array=w2506) -> (size(s)=w2507:i32[])
            n951 = Index Array(array=w2507) -> (element=w2505:i32)  [unwired: 1 in]
            n952 = Multiply(x=w2512, y=u32 2) -> (x*y=w2485:u32)
            n953 = Increment(x=w2485) -> (x+1=w2508:u32)
            n954 = case shown="1" w2510 {
              selector: w2510 -> [_ w2546 _]
              tunnel: w2509 -> [w2540 _ _]
              tunnel: [w2540 w2545 w2566] -> w2504
              tunnel: w2511 -> [_ w2547 w2567]
              tunnel: [32 ("ImageRows(32)") w2543 w2568] -> w2479
              tunnel: w2505 -> [_ w2542 _]
              tunnel: w2508 -> [_ w2544 w2569]
              tunnel: w2485 -> [_ w2541 w2565]
              frame 0 {
              }
              frame Default {
                n955 = disable-structure shown="Enabled" {
                  disable-tunnel: w2547 -> [w2555 w2559]
                  disable-tunnel: w2546 -> [w2554 w2556]
                  disable-tunnel: [w2552 w2560] -> w2545
                  disable-tunnel: w2544 -> [w2551 _]
                  disable-tunnel: [w2550 w2561] -> w2543
                  disable-tunnel: w2542 -> [w2548 w2557]
                  disable-tunnel: w2541 -> [_ w2558]
                  frame Disabled {
                    n956 = Decrement(x=w2554) -> (x-1=w2549:u16)
                    n957 = Array Subset(array=w2555, length=w2549) -> (w2553:i32[])  [unwired: 1 in]
                    n958 = Add Array Elements(numeric array=w2553) -> (sum=w2552:i32)
                    n959 = Compound Arithmetic op=ADD(w2551, w2548, w2552) -> (w2550:u32)
                  }
                  frame Enabled {
                    n960 = Decrement(x=w2556) -> ()  [unwired: 1 out]
                    n961 = Array Subset(array=w2559, length=w2556) -> (w2562:i32[])  [unwired: 1 in]
                    n962 = Add Array Elements(numeric array=w2562) -> (sum=w2561:i32)
                    n963 = Increment(x=w2558) -> (x+1=w2563:u32)
                    n964 = Compound Arithmetic op=ADD(w2563, w2557) -> (w2564:u32)
                    n965 = Subtract(x=w2561, y=w2564) -> (x-y=w2560:u32)
                  }
                }
              }
              frame 1 {
                n966 = disable-structure shown="Enabled" {
                  disable-tunnel: w2569 -> [w2573 _]
                  disable-tunnel: [w2572 w2575] -> w2568
                  disable-tunnel: w2567 -> [w2571 w2577]
                  disable-tunnel: [w2570 w2574] -> w2566
                  disable-tunnel: w2565 -> [_ w2576]
                  frame Disabled {
                    n967 = Index Array(array=w2571) -> (element=w2570:i32)  [unwired: 1 in]
                    n968 = Compound Arithmetic op=ADD(w2573, w2570) -> (w2572:u32)
                  }
                  frame Enabled {
                    n969 = Index Array(array=w2577) -> (element=w2575:i32)  [unwired: 1 in]
                    n970 = Subtract(x=w2575, y=w2576) -> (x-y=w2574:u32)
                  }
                }
              }
            }
            n971 = local read "_CapitalOnly"() -> (w2529:bool)
            n972 = local read "_TextAlignment"() -> (w2503:u16)
            n973 = local read "_BodyBk"() -> (w2519:T1)
            n974 = local read "_BodyText"() -> (w2517:T1)
            n975 = local read "_FontCompression"() -> (w2530:enum16{"Auto", "On", "Off"})
            n976 = Bundle By Name(cluster=T26 {"Text"="", "Allow Only Capital Chars"=FALSE, "Compression"=enum."Auto", "Alignment"=enum."Center"} ("Text"), "Alignment"=w2503, "Text"=w2480, "Allow Only Capital Chars"=w2529, "Compression"=w2530) -> (w2528:T26)
            n977 = Unbundle By Name(w2487) -> ("AF"=w2483:bool, "OldOffset.X"=w2498:i32, "OldOffset.Y"=w2497:i32)
            n978 = Unbundle(w2517) -> ("Color"=w2516:u32)  [unwired: 1 out]
            n979 = Unbundle(w2519) -> ("Color"=w2518:u32)  [unwired: 1 out]
            n980 = Unbundle By Name(w2496) -> ("X"=w2495:i32, "Y"=w2494:i32)
            n981 = call <resource>:"GDSLvIcon_GenerateIconText.vi"("Text"=w2528, "TextPixelHeight(5-30)"=w2504, "Foreground color"=w2516, "Background color"=w2518, "error in (no error)"=w2522, "Offset"=w2496, "Text Pixel width(32-FrameThicknes*2))"=w2521) -> ("X-Limited"=w2500:bool, "Y-Limited"=w2499:bool, "TextOut"=w2520:u8[][], "TextBounds"=w2490:T43, "error out"=w2532:errorcluster)  [unwired: 8 in]
            n982 = call <resource>:"GDSLvIcon_CreateIconPicture.vi"("FrameColor"=w2512, "FrameThickness(1)"=w2526, "HeaderIconIn"=w2506, "BodyIconIn"=w2520, "error in (no error)"=w2532, "ImageRows(32)"=w2479, "BigSizeIcon(x6)"=4, "BgIcon"=w2486) -> ("BodyIconOut"=w2484:u8[][], "LargeIconPictureOut(x6)"=→"_IconPreview":picture, "BodyOffset"=w2489:cluster{"X":i32, "Y":i32}, "error out"=w2523:errorcluster)  [unwired: 6 in, 2 out]
            n983 = Unbundle(w2489) -> ("X"=w2491:i32, "Y"=w2492:i32)
            n984 = Select(t=w2498, s=w2500, f=w2495) -> (s? t:f=w2501:i32)
            n985 = Select(t=w2497, s=w2499, f=w2494) -> (s? t:f=w2502:i32)
            n986 = Bundle("Y"=w2492, "X"=w2491, "Y"=w2492, "X"=w2491) -> (w2493:cluster{"Y":i32, "X":i32, "Y":i32, "X":i32})  [unwired: 1 in]
            n987 = Add(x=w2493, y=w2490) -> (x+y=w2488:cluster{i32, i32, i32, i32})
            n988 = Bundle By Name(cluster=w2487, "Offset.X"=w2501, "Offset.Y"=w2502, "MethodIcon"=w2520, "IconDetails.IconSize"=w2510, "IconDetails.ImageRows(32)"=w2479, "IconDetails.ConnectorPaneHeight"=w2511, "TextBounds"=w2488, "BodyIconOut"=w2484, "RowStart(0)"=0, "ImageRows(32)"=w2479) -> (w2514:T17)
            n989 = case shown="False" w2483 {
              tunnel: ["Idle" "ActorTemplates"] -> w2527
              frame False {
              }
              frame True {
              }
            }
          }
          frame "ActorTemplates" {
            w2598 = TRUE
            n990 = feedback-in #2(w2598) -> ()
            n991 = feedback #2() -> (w2599:bool)
            n992 = Not Equal?(x=w2598, y=w2599) -> (x != y?=w2597:bool)
            n993 = case shown="True" w2597 {
              tunnel: w2596 -> [_ w2657]
              tunnel: w2582 -> [w2642 w2648]
              tunnel: [w2642 w2645] -> w2586
              frame False {
              }
              frame True {
                n994 = call <resource>:"AF_GetClassAfInfo.vi"("DeriveFromClassRef"=w2657) -> ("AF Folder Path"=w2656:path)  [unwired: 5 in, 5 out]
                n995 = Build Path(base path=w2656, name or relative path="MethodTemplates") -> (appended path=w2643:path)
                n996 = Build Path(base path=w2643, name or relative path="Templates.ini") -> (appended path=w2653:path)
                n997 = call <vilib>:"Open Config Data.vi"("configuration file path"=w2653) -> ("error out"=w2652:errorcluster, "refnum"=w2651:T46)  [unwired: 8 in, 1 out]
                n998 = call <vilib>:"Get Section Names.vi"("error in (no error)"=w2652, "refnum"=w2651) -> ("error out"=w2649:errorcluster, "section names"=w2647:string[], "refnum out"=w2650:T46)  [unwired: 7 in]
                n999 = for {
                  tunnel: w2647 -> [w2663] mode=indexing
                  shift-right: [w2665] -> _
                  shift-left: w2649 -> [w2669]
                  shift-right: [w2666] -> _
                  shift-left: w2650 -> [w2670]
                  tunnel: [w2659] -> w2646 mode=indexing
                  tunnel: w2643 -> [w2658]
                  n1000 = call <vilib>:"Get Key Names.vi"("section"=w2663, "error in (no error)"=w2669, "refnum"=w2670) -> ("error out"=w2667:errorcluster, "key names"=w2664:string[], "refnum out"=w2668:T46)  [unwired: 5 in, 1 out]
                  n1001 = for {
                    shift-right: [w2681] -> w2666
                    shift-left: w2668 -> [w2683]
                    shift-right: [w2680] -> w2665
                    shift-left: w2667 -> [w2682]
                    tunnel: w2664 -> [w2671] mode=indexing
                    tunnel: w2663 -> [w2674]
                    tunnel: MethodType."AF-Method" ("Type") -> [w2678]
                    tunnel: T12 {"Type"=enum."Normal", "Name"="", "Path"=path "", "ExtraName"="", "Data"=variant} ("cluster") -> [w2677]
                    tunnel: [w2676] -> w2660 mode=indexing
                    tunnel: w2658 -> [w2675]
                    n1002 = Build Path(base path=w2675, name or relative path=w2671) -> (appended path=w2673:path)
                    n1003 = call-poly <vilib>:"Read Key.vi"("read raw string? (F)"=TRUE, "section"=w2674, "error in (no error)"=w2682, "key"=w2671, "refnum"=w2683) -> ("error out"=w2680:errorcluster, "value"=w2672:string, "refnum out"=w2681:T46)  [unwired: 3 in, 1 out]
                    n1004 = Bundle By Name(cluster=w2677, "Type"=w2678, "Name"=w2672, "Path"=w2673) -> (w2676:T12)
                  }
                  n1005 = Bundle(w2660) -> (w2659:cluster{T12[]})  [unwired: 1 in]
                }
                n1006 = To Lower Case(string=w2647) -> (all lower case string=w2644:string[])
                n1007 = Bundle By Name(cluster=w2648, "AF-MethodNames"=w2644, "AF-Methods"=w2646) -> (w2645:T17)
              }
            }
            n1008 = Unbundle By Name(w2582) -> ("AF"=w2581:bool)
            n1009 = local read "_MethodName"() -> (w2600:string)
            n1010 = call <vilib>:"Trim Whitespace.vi"("string"=w2600) -> ("trimmed string"=w2594:string)  [unwired: 1 in]
            n1011 = To Lower Case(string=w2594) -> (all lower case string=w2593:string)
            n1012 = Unbundle By Name(w2586) -> ("AF-MethodNames"=w2595:string[], "AF-Methods"=w2590:cluster{T12[]}[])
            n1013 = Search 1D Array(1D array=w2595, element=w2593) -> (index of element=w2583:i32)  [unwired: 1 in]
            n1014 = Index Array(array=w2590, index=w2583) -> (element=w2589:cluster{T12[]})
            n1015 = Unbundle(w2589) -> (w2588:T12[])
            n1016 = Greater Or Equal To 0?(x=w2583) -> (x >= 0?=w2584:bool)
            n1017 = feedback-in #3(w2584) -> ()
            n1018 = feedback #3() -> (w2592:bool)
            n1019 = Compound Arithmetic op=AND(invert w2584, w2592) -> (w2591:bool)
            n1020 = case shown="True" w2584 {
              tunnel: w2591 -> [w2606 _]
              tunnel: w2582 -> [w2605 _]
              tunnel: w2588 -> [_ w2634]
              tunnel: w2581 -> [w2604 _]
              tunnel: [w2603 w2632] -> w2580
              tunnel: [w2602 w2631] -> w2579
              frame False {
                n1021 = case shown="False" w2606 {
                  tunnel: w2605 -> [w2609 w2615]
                  tunnel: w2604 -> [_ w2612]
                  tunnel: [w2608 w2611] -> w2603
                  tunnel: [w2607 w2610] -> w2602
                  frame False {
                    n1022 = Unbundle By Name(w2609) -> ("MethodItemNames"=w2607:string[], "MethodVIs"=w2608:path[])
                  }
                  frame True {
                    n1023 = local write "_AddMessageClass"(w2612) -> ()
                    n1024 = local read "_MethodType"() -> (w2616:T2)
                    n1025 = case shown="\"Property Method\"" w2616 {
                      tunnel: w2615 -> [w2624 w2626 w2628 w2630]
                      tunnel: [w2623 w2625 w2627 w2629] -> w2613
                      frame "Normal Method", Default {
                        n1026 = Unbundle By Name(w2624) -> ("NormalMethods"=w2623:T12[])
                      }
                      frame "Override Method" {
                        n1027 = Unbundle By Name(w2626) -> ("OverrideMethods"=w2625:T12[])
                      }
                      frame "Property Method" {
                        n1028 = Unbundle By Name(w2628) -> ("PropertyMethods"=w2627:T12[])
                      }
                      frame "Property Node" {
                        n1029 = Unbundle By Name(w2630) -> ("PropertyNodeMethods"=w2629:T12[])
                      }
                    }
                    n1030 = for {
                      tunnel: w2613 -> [w2618] mode=indexing
                      tunnel: [w2620] -> w2614 mode=indexing
                      tunnel: [w2619] -> w2610 mode=indexing
                      tunnel: [w2617] -> w2611 mode=indexing
                      n1031 = Unbundle(w2618) -> ("Name"=w2619:string, "Path"=w2617:path)  [unwired: 3 out]
                      n1032 = case shown="\"\"" w2619 {
                        tunnel: [0 -1] -> w2620
                        frame Default {
                        }
                        frame "" {
                        }
                      }
                    }
                    n1033 = property on="_Method" class="LstBox (strict)"("Item Names"=w2610, "Item Symbols"=w2614) -> ()  [unwired: 2 in, 2 out]
                  }
                }
              }
              frame True {
                n1034 = local write "_AddMessageClass"(FALSE ("_AddMessageClass")) -> ()
                n1035 = for {
                  tunnel: w2634 -> [w2637] mode=indexing
                  tunnel: [w2639] -> w2635 mode=indexing
                  tunnel: [w2638] -> w2631 mode=indexing
                  tunnel: [w2636] -> w2632 mode=indexing
                  n1036 = Unbundle(w2637) -> ("Name"=w2638:string, "Path"=w2636:path)  [unwired: 3 out]
                  n1037 = case shown="\"\"" w2638 {
                    tunnel: [0 -1] -> w2639
                    frame Default {
                    }
                    frame "" {
                    }
                  }
                }
                n1038 = property on="_Method" class="LstBox (strict)"("Item Names"=w2631, "Item Symbols"=w2635) -> ()  [unwired: 2 in, 2 out]
              }
            }
            n1039 = Bundle By Name(cluster=w2586, "AF-Method"=w2583, "MethodVIs"=w2580, "MethodItemNames"=w2579) -> (w2585:T17)
          }
          frame "UpdateIcon:2" {
            w2712 = T40 {"BgIcon"=[], "BgIconOffset"={"X"=0, "Y"=0}, "BgIconMask"=[], "ColorsOkayforiconToBeOnTopOf"=[]}  # BgIcon
            n1040 = Unbundle By Name(w2688) -> ("Frame thickness"=w2709:i32, "ConnectorPaneHeight"=w2697:i32[], "BodyIconHeight"=w2698:i32, "MethodIcon"=w2687:u8[][])
            n1041 = Unbundle By Name(w2688) -> ("Frame"=w2704:u32, "Frame thickness"=w2695:i32, "HeaderIcon"=w2701:u8[][])
            n1042 = local read "_IconSize"() -> (w2705:u16)
            n1043 = local read "_BodyBk"() -> (w2691:T1)
            n1044 = Unbundle By Name(w2691) -> ("Color"=w2719:u32)
            n1045 = Unbundle By Name(w2688) -> ("BgIcon"=w2713:u8[][], "BgIconOffset"=w2714:cluster{"X":i32, "Y":i32}, "BgIconMask"=w2716:u8[], "HeaderBkColor"=w2717:u32)
            n1046 = case shown="Default" w2705 {
              tunnel: w2701 -> [w2736 _]
              tunnel: [w2736 _] -> w2702
              frame Default {
              }
              frame 1 {
              }
            }
            n1047 = Not Equal?(x=u16 0, y=w2705) -> (x != y?=w2706:bool)
            n1048 = Array Size(array=w2702) -> (size(s)=w2699:i32[])
            n1049 = Index Array(array=w2699) -> (element=w2700:i32)  [unwired: 1 in]
            n1050 = call <resource>:"GDSLvIcon_Convert24bitTo8bitColor.vi"("Color 24bit In"=w2717) -> ("Color out(256)"=w2718:u8)  [unwired: 15 in, 3 out]
            n1051 = call <resource>:"GDSLvIcon_Convert24bitTo8bitColor.vi"("Color 24bit In"=w2719) -> ("Color out(256)"=w2720:u8)  [unwired: 15 in, 3 out]
            n1052 = Select(t=0, s=w2706, f=0) -> (s? t:f=w2708:i32)
            n1053 = Multiply(x=w2709, y=u32 2) -> (x*y=w2710:u32)
            n1054 = case shown="1" w2705 {
              selector: w2705 -> [_ w2724 _]
              tunnel: w2698 -> [_ _ _]
              tunnel: w2697 -> [_ w2731 w2734]
              tunnel: [32 ("ImageRows(32)") w2728 w2735] -> w2703
              tunnel: w2700 -> [_ w2727 _]
              tunnel: w2710 -> [_ w2726 w2732]
              frame 0 {
              }
              frame Default {
                n1055 = Decrement(x=w2724) -> ()  [unwired: 1 out]
                n1056 = Array Subset(array=w2731, length=w2724) -> (w2730:i32[])  [unwired: 1 in]
                n1057 = Add Array Elements(numeric array=w2730) -> (sum=w2729:i32)
                n1058 = Increment(x=w2726) -> (x+1=w2725:u32)
                n1059 = Compound Arithmetic op=ADD(w2725, w2727, w2729) -> (w2728:u32)
              }
              frame 1 {
                n1060 = Index Array(array=w2734) -> (element=w2733:i32)  [unwired: 1 in]
                n1061 = Compound Arithmetic op=ADD(w2732, w2733) -> (w2735:u32)
              }
            }
            n1062 = Build Array(w2718, w2720) -> (w2715:u8[])
            n1063 = Bundle By Name(cluster=w2712, "BgIcon"=w2713, "BgIconOffset"=w2714, "BgIconMask"=w2716, "ColorsOkayforiconToBeOnTopOf"=w2715) -> (w2721:T40)
            n1064 = call <resource>:"GDSLvIcon_CreateIconPicture.vi"("FrameColor"=w2704, "FrameThickness(1)"=w2695, "HeaderIconIn"=w2702, "BodyIconIn"=w2687, "error in (no error)"=w2693, "ImageRows(32)"=w2703, "BigSizeIcon(x6)"=4, "RowStart(0)"=w2708, "BgIcon"=w2721) -> ("BodyIconOut"=w2684:u8[][], "WholeIconOut"=w2722:u8[][], "LargeIconPictureOut(x6)"=w2711:picture, "error out"=w2692:errorcluster)  [unwired: 5 in, 2 out]
            n1065 = local write "_IconPreview"(w2711) -> ()
            n1066 = Bundle By Name(cluster=w2688, "CurrentIcon"=w2721, "IconOut"=w2722, "BodyIconOut"=w2684) -> (w2690:T17)
          }
          frame "UpdateIconFromParentMethod" {
            w2769 = T40 {"BgIcon"=[], "BgIconOffset"={"X"=0, "Y"=0}, "BgIconMask"=[], "ColorsOkayforiconToBeOnTopOf"=[]}  # BgIcon
            n1067 = Unbundle By Name(w2741) -> ("OverrideMethod"=w2746:path)
            n1068 = call <resource>:"GDSLvIcon_AnalyseViIcon.vi"("ViRef/LvCLassRef/LvLibRef/ViPath/2D_Image"=w2746, "error in (no error)"=w2745) -> ("FrameThickness(1)"=w2744:u32, "BodyIcon"=w2743:u8[][], "BodyBkColor"=w2740:u32)  [unwired: 5 in, 10 out]
            n1069 = Unbundle By Name(w2741) -> ("Frame"=w2762:u32, "Frame thickness"=w2754:i32, "HeaderIcon"=w2759:u8[][])
            n1070 = Unbundle By Name(w2741) -> ("ConnectorPaneHeight"=w2756:i32[])  [unwired: 3 out]
            n1071 = local read "_BodyBk"() -> (w2752:T1)
            n1072 = Unbundle By Name(w2752) -> ("Color"=w2738:u32)
            n1073 = local read "_IconSize"() -> (w2763:u16)
            n1074 = call <resource>:"GDSLvIcon_Convert24bitTo8bitColor.vi"("Color 24bit In"=w2738) -> ("Color out(256)"=w2739:u8)  [unwired: 15 in, 3 out]
            n1075 = call <resource>:"GDSLvIcon_ReplaceIconColor.vi"("IconIn"=w2743, "OldColor"=w2740, "NewColor"=w2738) -> ("IconOut"=w2742:u8[][])  [unwired: 15 in, 1 out]
            n1076 = Unbundle By Name(w2741) -> ("BgIcon"=w2770:u8[][], "BgIconOffset"=w2771:cluster{"X":i32, "Y":i32}, "BgIconMask"=w2773:u8[], "HeaderBkColor"=w2774:u32)
            n1077 = case shown="Default" w2763 {
              tunnel: w2759 -> [w2791 _]
              tunnel: [w2791 _] -> w2760
              frame Default {
              }
              frame 1 {
              }
            }
            n1078 = Not Equal?(x=u16 0, y=w2763) -> (x != y?=w2764:bool)
            n1079 = Array Size(array=w2760) -> (size(s)=w2757:i32[])
            n1080 = Index Array(array=w2757) -> (element=w2758:i32)  [unwired: 1 in]
            n1081 = call <resource>:"GDSLvIcon_Convert24bitTo8bitColor.vi"("Color 24bit In"=w2774) -> ("Color out(256)"=w2775:u8)  [unwired: 15 in, 3 out]
            n1082 = Select(t=0, s=w2764, f=0) -> (s? t:f=w2766:i32)
            n1083 = Multiply(x=w2744, y=u32 2) -> (x*y=w2767:u32)
            n1084 = case shown="Default" w2763 {
              selector: w2763 -> [_ w2779 _]
              tunnel: w2756 -> [_ w2786 w2789]
              tunnel: [32 ("ImageRows(32)") w2783 w2790] -> w2761
              tunnel: w2758 -> [_ w2782 _]
              tunnel: w2767 -> [_ w2781 w2787]
              frame 0 {
              }
              frame Default {
                n1085 = Array Subset(array=w2786, length=w2779) -> (w2785:i32[])  [unwired: 1 in]
                n1086 = Add Array Elements(numeric array=w2785) -> (sum=w2784:i32)
                n1087 = Increment(x=w2781) -> (x+1=w2780:u32)
                n1088 = Compound Arithmetic op=ADD(w2780, w2782, w2784) -> (w2783:u32)
              }
              frame 1 {
                n1089 = Index Array(array=w2789) -> (element=w2788:i32)  [unwired: 1 in]
                n1090 = Compound Arithmetic op=ADD(w2787, w2788) -> (w2790:u32)
              }
            }
            n1091 = Build Array(w2775, w2739) -> (w2772:u8[])
            n1092 = Bundle By Name(cluster=w2769, "BgIcon"=w2770, "BgIconOffset"=w2771, "BgIconMask"=w2773, "ColorsOkayforiconToBeOnTopOf"=w2772) -> (w2776:T40)
            n1093 = call <resource>:"GDSLvIcon_CreateIconPicture.vi"("FrameColor"=w2762, "FrameThickness(1)"=w2754, "HeaderIconIn"=w2760, "BodyIconIn"=w2742, "error in (no error)"=w2745, "ImageRows(32)"=w2761, "BigSizeIcon(x6)"=4, "RowStart(0)"=w2766, "BgIcon"=w2776) -> ("BodyIconOut"=w2747:u8[][], "WholeIconOut"=w2777:u8[][], "LargeIconPictureOut(x6)"=w2768:picture, "error out"=w2737:errorcluster)  [unwired: 5 in, 2 out]
            n1094 = local write "_IconPreview"(w2768) -> ()
            n1095 = Bundle By Name(cluster=w2741, "CurrentIcon"=w2776, "IconOut"=w2777, "BodyIconOut"=w2747) -> (w2751:T17)
            n1096 = call <vilib>:"Unset Busy.vi"("error in (no error)"=w2737) -> ()  [unwired: 10 in, 1 out]
          }
          frame "ShowDragIcon", "ShowDragIcon:UpdateIcon" {
            w2810 = 2.0 ("Waveform Chart")
            w2821 = 4 ("x")
            n1097 = Unbundle By Name(w2796) -> ("IconNames"=w2835:string[], "Icons"=w2799:T15[], "IconSelected"=w2836:i32, "IconPos"=w2802:T41)
            n1098 = Index Array(array=w2835, index=w2836) -> (element=→"_IconName":string)
            n1099 = Index Array(array=w2799, index=w2836) -> (element=w2793:T15)
            n1100 = Index Array(array=w2802, index=w2836) -> (element=w2803:T45)
            n1101 = Unbundle By Name(w2803) -> ("left"=w2804:i16, "top"=w2808:i16, "right"=w2805:i16, "bottom"=w2807:i16)
            n1102 = call <resource>:"GDSIconEditor_ShrinkImage.vi"("image data"=w2793) -> ("image subset"=w2792:T15)  [unwired: 9 in]
            n1103 = Unbundle By Name(w2792) -> ("Rectangle.right"=w2828:i16, "Rectangle.bottom"=w2827:i16)
            n1104 = call <vilib>:"Draw Flattened Pixmap.vi"("image data"=w2792) -> ("new picture"=w2819:picture)  [unwired: 8 in]
            n1105 = property on="Icons" class="Pict"() -> ("Position"=w2833:T29)  [unwired: 2 in, 2 out]
            n1106 = property on="Icons" class="Pict"() -> ("Origin"=w2832:T30)  [unwired: 2 in, 2 out]
            n1107 = Add(x=w2808, y=w2807) -> (x+y=w2809:i16)
            n1108 = Add(x=w2804, y=w2805) -> (x+y=w2806:i16)
            n1109 = Divide(x=w2809, y=w2810) -> (x/y=w2812:dbl)
            n1110 = Divide(x=w2806, y=w2810) -> (x/y=w2811:dbl)
            n1111 = Subtract(x=w2833, y=w2832) -> (x-y=w2834:T29)
            n1112 = Bundle("right"=w2828, "bottom"=w2827) -> (w2820:cluster{"right":i16, "bottom":i16})  [unwired: 1 in]
            n1113 = Bundle(w2811, w2812) -> (w2813:cluster{dbl, dbl})  [unwired: 1 in]
            n1114 = Increment(x=w2820) -> (x+1=w2801:cluster{"right":i16, "bottom":i16})
            n1115 = Add(x=w2813, y=w2834) -> (x+y=w2814:cluster{dbl, dbl})
            n1116 = Divide(x=w2801, y=2.0 ("Waveform Chart")) -> (x/y=w2822:cluster{"right":dbl, "bottom":dbl})
            n1117 = Multiply(x=w2821, y=w2822) -> (x*y=w2823:cluster{"right":dbl, "bottom":dbl})
            n1118 = Subtract(x=w2814, y=w2823) -> (x-y=w2830:cluster{dbl, dbl})
            n1119 = Multiply(x=w2821, y=w2828) -> (x*y=w2817:i32)
            n1120 = Multiply(x=w2821, y=w2827) -> (x*y=w2818:i32)
            n1121 = Equal?(x=w2798, y="ShowDragIcon:UpdateIcon") -> (x = y?=w2831:bool)
            n1122 = Bundle(w2817, w2818) -> (w2816:cluster{i32, i32})  [unwired: 1 in]
            n1123 = Select(t="UpdateIcon", s=w2831, f="Idle" ("y")) -> (s? t:f=w2797:string)
            n1124 = property on="DragIcon" class="Pict"("Draw Area Size"=w2816, "Value"=w2819, "Visible"=TRUE) -> (error out=w2829:errorcluster)  [unwired: 2 in, 1 out]
            n1125 = case shown="False" w2831 {
              tunnel: w2829 -> [w2838 _]
              tunnel: w2830 -> [w2837 _]
              frame False {
                n1126 = property on="DragIcon" class="Pict"(error in=w2838, "Position"=w2837) -> ()  [unwired: 1 in, 2 out]
              }
              frame True {
              }
            }
          }
          frame "Error", "Exit", Default {
            n1127 = Unbundle By Name(w2842) -> ("Cancel"=w2841:bool)
            n1128 = Unbundle By Name(w2843) -> ("status"=w2840:bool)
            n1129 = Or(x=w2841, y=w2840) -> (x .or. y?=w2839:bool)
            n1130 = Bundle By Name(cluster=w2842, "Cancel"=w2839) -> (w2845:T17)
          }
        }
      }
    }
    frame Error {
    }
  }
  "error out" <- w32
  n1131 = call <resource>:"GDSString_AddStatesToQueue.vi"() -> ()  [unwired: 15 in, 1 out]
  n1132 = Generate User Event(user event=w5, event data cluster="Stop" ("Stop")) -> (user event out=w10:refnum<user-event>)  [unwired: 2 in, 1 out]
  n1133 = Destroy User Event(user event=w10) -> ()  [unwired: 1 in, 1 out]
  n1134 = stacked-sequence {
    tunnel: w44 -> [w2912]
    tunnel: [w2924] -> w43
    tunnel: [w2890] -> w36
    tunnel: [w2923] -> w37
    tunnel: [w2874] -> w35
    tunnel: [w2894] -> w38
    tunnel: [w2921] -> w39
    tunnel: [w2920] -> w40
    tunnel: [w2858] -> w34
    tunnel: ["_DynamicDispatch"] -> w33
    tunnel: [w2914] -> w31
    tunnel: [w2915] -> w30
    tunnel: ["_MustOverride"] -> w27
    tunnel: ["_MustCallParent"] -> w26
    tunnel: [w2883] -> w25
    tunnel: [w2882] -> w20
    tunnel: [w2862] -> w15
    frame #0 {
      n1135 = Unbundle By Name(w2912) -> ("OverrideMethodsIdx"=w2850:i32[], "AF-Method"=w2877:i32, "AllOverrideMethods"=w2876:path[], "AF"=w2881:bool, "ActorVersion"=w2880:string, "IsAPropertyDefinitionVI"=w2868:bool[])
      n1136 = Unbundle By Name(w2912) -> ("Signatures.SignatureName"=w2908:string[], "Signatures.SignatureText"=w2909:string[], "Signatures.Current"=w2911:i32)
      n1137 = Unbundle By Name(w2912) -> ("FolderNames"=w2919:string[], "IconDetails"=w2883:T5, "Open"=w2915:bool, "Cancel"=w2924:bool, "RelFolderPath"=w2873:path[], "BodyIconOut"=w2920:u8[][], "MethodNames"=w2871:string[])
      n1138 = local read "_MethodSignature"() -> (w2907:u16)
      n1139 = local read "_Visibility"() -> (w2922:T7)
      n1140 = local read "_MethodName"() -> (w2852:string)
      n1141 = local read "_MethodType"() -> (w2916:T2)
      n1142 = property on="_Visibility" class="RadioBtnsControl (strict)"() -> ("Disabled"=w2878:T19)  [unwired: 2 in, 2 out]
      n1143 = local read "_MethodType"() -> (w2866:T2)
      n1144 = local read "_MethodLocation"() -> (w2918:i32)
      n1145 = Index Array(array=w2919, index=w2918) -> (element=w2872:string)
      n1146 = Match Pattern(string=w2852, regular expression="\\2E[Vv][Ii][Mm]*") -> (before substring=w2851:string)  [unwired: 1 in, 3 out]
      n1147 = local read "_Method"() -> (w2870:i32[])
      n1148 = Array Size(array=w2870) -> (size(s)=w2869:i32)
      n1149 = case shown="-1" w2877 {
        selector: w2877 -> [w2938 _]
        tunnel: w2916 -> [_ w2949]
        tunnel: w2876 -> [_ w2948]
        tunnel: [_ w2947] -> w2913
        tunnel: w2912 -> [w2940 w2946]
        tunnel: [w2936 w2945] -> w2906
        tunnel: w2851 -> [_ w2944]
        tunnel: w2869 -> [_ w2943]
        tunnel: w2868 -> [_ w2942]
        tunnel: [_ w2941] -> w2864
        frame 0, Default {
          n1150 = Unbundle By Name(w2940) -> ("AF-Methods"=w2939:cluster{T12[]}[])
          n1151 = Index Array(array=w2939, index=w2938) -> (element=w2937:cluster{T12[]})
          n1152 = Unbundle(w2937) -> (w2936:T12[])
        }
        frame -1 {
          n1153 = case shown="\"Override Method\"" w2949 {
            tunnel: w2948 -> [_ w2960 _ _]
            tunnel: [_ w2959 w2970 w2991] -> w2947
            tunnel: w2946 -> [w2951 w2958 w2969 w2990]
            tunnel: [w2950 w2957 w2968 w2989] -> w2945
            tunnel: w2944 -> [_ _ _ w2982]
            tunnel: w2943 -> [_ _ w2963 w2979]
            tunnel: w2942 -> [_ w2956 _ _]
            tunnel: [_ w2955 _ _] -> w2941
            frame "Normal Method", Default {
              n1154 = Unbundle By Name(w2951) -> ("NormalMethods"=w2950:T12[])
            }
            frame "Override Method" {
              n1155 = local read "_OverrideMethods"() -> (w2954:i32)
              n1156 = Unbundle By Name(w2958) -> ("OverrideMethods"=w2957:T12[], "OverrideMethodsIdx"=w2953:i32[])
              n1157 = Index Array(array=w2953, index=w2954) -> (element=w2952:i32)
              n1158 = Index Array(array=w2956, index=w2952) -> (element=w2955:bool)
              n1159 = Index Array(array=w2960, index=w2952) -> (element=w2959:path)
            }
            frame "Property Method" {
              n1160 = local read "_Property"() -> (w2962:string[])
              n1161 = Unbundle By Name(w2969) -> ("PropertyMethods"=w2968:T12[])
              n1162 = for {
                tunnel: w2962 -> [w2975] mode=indexing
                tunnel: w2963 -> [w2974]
                shift-right: [w2973] -> w2961
                shift-left: string[] [] -> [w2972]
                n1163 = Initialize Array(w2975, w2974) -> (w2971:string[])
                n1164 = Build Array (concatenate)(w2972, w2971) -> (w2973:string[])
              }
              n1165 = Bundle(cluster=T9 {"AttributeNames"=[], "PropertyNode"=FALSE, "FolderNames"=[]}, "AttributeNames"=w2961, "PropertyNode"=FALSE) -> (w2966:T9)  [unwired: 1 in]
              n1166 = To Variant(anything=w2966) -> (Variant=w2970:variant)
            }
            frame "Property Node" {
              w2978 = string[] []
              n1167 = Unbundle By Name(w2990) -> ("PropertyNodeMethods"=w2989:T12[])
              n1168 = local read "_Property"() -> (w2977:string[])
              n1169 = Spreadsheet String To Array(delimiter (Tab)="/", format string="%s", spreadsheet string=w2982, array type (2D Dbl)=string[] []) -> (array=w2983:string[])
              n1170 = for {
                tunnel: w2977 -> [w2996] mode=indexing
                tunnel: w2979 -> [w2995]
                shift-right: [w2994] -> w2976
                shift-left: w2978 -> [w2993]
                n1171 = Initialize Array(w2996, w2995) -> (w2992:string[])
                n1172 = Build Array (concatenate)(w2993, w2992) -> (w2994:string[])
              }
              n1173 = for {
                tunnel: w2983 -> [w3001] mode=indexing
                tunnel: w2979 -> [w3000]
                shift-right: [w2999] -> w2980
                shift-left: w2978 -> [w2998]
                n1174 = Initialize Array(w3001, w3000) -> (w2997:string[])
                n1175 = Build Array (concatenate)(w2998, w2997) -> (w2999:string[])
              }
              n1176 = Bundle(cluster=T9 {"AttributeNames"=[], "PropertyNode"=FALSE, "FolderNames"=[]}, "AttributeNames"=w2976, "PropertyNode"=TRUE, "FolderNames"=w2980) -> (w2987:T9)
              n1177 = To Variant(anything=w2987) -> (Variant=w2991:variant)
            }
          }
        }
      }
      n1178 = case shown="\"Disabled and Grayed Out\"" w2878 {
        tunnel: w2922 -> [_ w3054]
        tunnel: [GOOP300_MethodScopeType."Use Parent Folder Scope" ("Scope/Visibility") w3053] -> w2921
        frame "Disabled and Grayed Out" {
        }
        frame Default {
          n1179 = case shown="\"Community\"" w3054 {
            tunnel: [GOOP300_MethodScopeType."Protected" ("Scope/Visibility") GOOP300_MethodScopeType."Private" ("Scope/Visibility") GOOP300_MethodScopeType."Public" ("Scope/Visibility") GOOP300_MethodScopeType."Community" ("Scope/Visibility")] -> w3053
            frame "Protected" {
            }
            frame "Private" {
            }
            frame "Public" {
            }
            frame "Community" {
            }
          }
        }
      }
      n1180 = Index Array(array=w2873, index=w2918) -> (element=w2875:path)
      n1181 = Not Equal?(x=w2911, y=w2907) -> (x != y?=w2910:bool)
      n1182 = local read "_MethodDescription"() -> (w2923:string)
      n1183 = Equal?(x=T2."Property Node" ("_MethodType"), y=w2866) -> (x = y?=w2865:bool)
      n1184 = Build Array(w2851) -> (w2896:string[])
      n1185 = Empty Array?(array=w2871) -> (empty?=w2895:bool)
      n1186 = Select(t=w2896, s=w2895, f=w2871) -> (s? t:f=w2856:string[])
      n1187 = Or(x=w2865, y=w2864) -> (x .or. y?=w2863:bool)
      n1188 = case shown="True" w2863 {
        tunnel: w2875 -> [_ w2935]
        tunnel: [w2932 w2935] -> w2874
        tunnel: w2873 -> [w2933 _]
        tunnel: w2872 -> [_ w2934]
        tunnel: [w2931 w2934] -> w2857
        frame True {
          w2931 = "properties"
          n1189 = Index Array(array=w2933) -> ()  [unwired: 1 in, 1 out]
          n1190 = String To Path(string=w2931) -> (path=w2932:path)
        }
        frame False {
        }
      }
      n1191 = local read ".vim"() -> (w2854:bool)
      n1192 = case shown="True" w2854 {
        tunnel: w2856 -> [w2925 w2927]
        tunnel: [w2925 w2926] -> w2855
        frame False {
        }
        frame True {
          n1193 = for {
            tunnel: w2927 -> [w2930] mode=indexing
            tunnel: [w2928] -> w2926 mode=indexing
            n1194 = Concatenate Strings(w2930, ".vim" ("string")) -> (w2928:string)
          }
        }
      }
      n1195 = for {
        tunnel: w2906 -> [w3018]
        tunnel: [w3016] -> w2905
        tunnel: [w3015] -> w2887 mode=indexing
        tunnel: [w3014] -> w2904
        tunnel: [w3013] -> w2862
        tunnel: [w3012] -> w2903
        tunnel: [w3011] -> w2902
        tunnel: w2870 -> [w3010] mode=indexing
        n1196 = Index Array(array=w3018, index=w3010) -> (element=w3017:T12)
        n1197 = Unbundle By Name(w3017) -> ("Type"=w3016:T13, "Name"=w3014:string, "Path"=w3013:path, "ExtraName"=w3011:string, "Data"=w3012:variant)
        n1198 = Strip Path(path=w3013) -> (name=w3015:string)  [unwired: 1 out]
      }
      n1199 = case shown="True" w2910 {
        tunnel: w2909 -> [_ w3043]
        tunnel: w2908 -> [_ w3042]
        tunnel: w2907 -> [_ w3041]
        frame False {
        }
        frame True {
          n1200 = Array Size(array=w3043) -> (size(s)=w3049:i32)
          n1201 = call <resource>:"GOOP_GetGDSConfigFolder.vi"() -> ("GDSFolderPath"=w3050:path)
          n1202 = Max & Min(x=w3049, y=w3041) -> (min(x,y)=w3048:i32)  [unwired: 1 out]
          n1203 = Build Path(base path=w3050, name or relative path="MethodSignatures.xml") -> (appended path=w3046:path)
          n1204 = Bundle("SignatureName"=w3042, "SignatureText"=w3043, w3048) -> (w3047:T48)  [unwired: 1 in]
          n1205 = Delete(path (use dialog)=w3046) -> (deleted path=w3045:path)  [unwired: 4 in, 2 out]
          n1206 = Flatten To XML(6:w3047) -> (2:w3044:string)
          n1207 = Write to Text File(file (use dialog)=w3045, text=w3044) -> ()  [unwired: 2 in, 3 out]
        }
      }
      n1208 = case shown="True" w2881 {
        tunnel: [_ w3006] -> w2882
        tunnel: w2880 -> [_ w3004]
        tunnel: cluster{"Add":bool, "ActorVersion":string} {"Add"=FALSE, "ActorVersion"=""} ("cluster") -> [_ w3002]
        frame False {
        }
        frame True {
          n1209 = Bundle(cluster=w3002, "Add"="_AddMessageClass", "ActorVersion"=w3004) -> (w3003:cluster{"Add":bool, "ActorVersion":string})
          n1210 = To Variant(anything=w3003) -> (Variant=w3006:variant)
        }
      }
      n1211 = Array Size(array=w2856) -> (size(s)=w2885:i32)
      n1212 = Array Size(array=w2887) -> (size(s)=w2886:i32)
      n1213 = Equal?(x=w2857, y="<class root>") -> (x = y?=w2860:bool)
      n1214 = Divide(x=w2885, y=w2886) -> (x/y=w2884:dbl)
      n1215 = for {
        N: w2884 -> [_]
        shift-right: [w3008] -> w2889
        shift-left: string[] [] -> [w3009]
        tunnel: w2887 -> [w3007]
        n1216 = Build Array (concatenate)(w3009, w3007) -> (w3008:string[])
      }
      n1217 = Select(t="", s=w2860, f=w2857) -> (s? t:f=w2858:string)
      n1218 = case shown="\"AF-Method\"" w2905 {
        selector: w2905 -> [_ w3027 _ _]
        tunnel: [w3019 w3025 w3032 w3040] -> w2914
        tunnel: w2913 -> [w3019 _ _ _]
        tunnel: w2904 -> [_ _ w3031 w3038]
        tunnel: w2862 -> [_ w3026 _ w3037]
        tunnel: w2903 -> [_ _ w3030 w3036]
        tunnel: w2902 -> [_ _ _ w3034]
        tunnel: w2876 -> [_ w3024 _ _]
        tunnel: w2850 -> [_ w3022 _ _]
        frame "Normal", Default {
        }
        frame "AF-Method" {
          n1219 = local read "_OverrideMethods"() -> (w3021:i32)
          n1220 = Index Array(array=w3022, index=w3021) -> (element=w3020:i32)
          n1221 = Index Array(array=w3024, index=w3020) -> (element=w3023:path)
          n1222 = Bundle("Type"=w3027, "Path"=w3026, "Path"=w3023) -> (w3025:cluster{"Type":T13, "Path":path, "Path":path})  [unwired: 1 in]
        }
        frame "MethodPlugIn" {
          n1223 = Variant To Data(type=" ", Variant=w3030) -> (data=w3028:string)  [unwired: 1 in, 1 out]
          n1224 = Bundle(cluster=T47 {"PlugInName"="", "MethodSelected"=""}, "PlugInName"=w3028, "MethodSelected"=w3031) -> (w3032:T47)
        }
        frame "DesignPattern" {
          n1225 = Bundle(cluster=T10 {"Type"=enum."DesignPattern", "ID"="", "Version"="", "Path"=path "", "Name"="", "Data"=variant}, "Type"=GDSLvClass_PlugInTypes."DesignPattern", "ID"=w3038, "Path"=w3037, "Name"=w3034, "Data"=w3036) -> (w3040:T10)  [unwired: 1 in]
        }
      }
      n1226 = Array To Spreadsheet String(delimiter (Tab)="\n", array=w2855, 3:"%s" ("format string")) -> (spreadsheet string=w2892:string)
      n1227 = call <vilib>:"Trim Whitespace.vi"("string"=w2892) -> ("trimmed string"=w2890:string)  [unwired: 1 in]
      n1228 = Array To Spreadsheet String(delimiter (Tab)="\n", array=w2889, 3:"%s" ("format string")) -> (spreadsheet string=w2898:string)
      n1229 = call <vilib>:"Trim Whitespace.vi"("string"=w2898) -> ("trimmed string"=w2894:string)  [unwired: 1 in]
    }
  }
  "Cancelled" <- w43
  n1230 = Bundle By Name(cluster=T3 {"MethodName"="", "RelativeMethodPath"=path "", "MethodDescription"="", "Scope/Visibility"=enum."Use Parent Folder Scope", "MethodTemplateName"="", "IconOut"=[], "RelativeProjectClassPath"="", "OpenViAfterCreation"=FALSE, "DynamicDispatchVi"=FALSE, "ExtraCreateParameters"=variant, "MustOverride"=FALSE, "MustCallParent"=FALSE, "IconDetails"={"IconSize"=enum."Full", "ImageRows(32)"=0, "ConnectorPaneHeight"=[]}, "AF-Option"=variant, "TemplatePath"=path ""} ("CreateMethodData"), "IconDetails"=w25, "RelativeProjectClassPath"=w34, "OpenViAfterCreation"=w30, "RelativeMethodPath"=w35, "MethodName"=w36, "MethodDescription"=w37, "IconOut"=w40, "Scope/Visibility"=w39, "MethodTemplateName"=w38, "DynamicDispatchVi"=w33, "ExtraCreateParameters"=w31, "MustOverride"=w27, "MustCallParent"=w26, "AF-Option"=w20, "TemplatePath"=w15) -> (→"CreateMethodData":T3)
  "_DubMethodName" <- "" ("_DubMethodName")
  "_MethodsLlocationOverrideInfo" <- "" ("_MethodsLlocationOverrideInfo")
